vi "Beampointing_BELLA_PICObooster2.vi"() -> ()   [LabVIEW 2013]
uses:
  shared programs/GUI_Template/GUI_master/tcp_new_data_event.ctl
  shared programs/GUI_Template/GUI_master/tcp new data cluster.ctl
  Ctrs/beam detection.ctl
  GUI_Beampointing_single_TRA/Ctrs/move.ctl
  GUI_Stage_Cameras/Controls/Crosshair type def.ctl
  <vilib>/Utility/file.llb/Read From Spreadsheet File (string).vi
  <userlib>/_OpenG.lib/array/array.llb/Filter 1D Array with Scalar (String)__ogtk.vi
  <vilib>/Utility/file.llb/Write To Spreadsheet File (string).vi
  <vilib>/Analysis/NI_AALBase.lvlib
  <vilib>/vision/NI_Vision_Development_Module.lvlib
panel:
  in  "Position.Axis 121::98":dbl caption="Motor Axis 1" min=-10000.0 max=10000.0 format="%#_6f"
  in  "Position.Axis 122::98":dbl caption="Motor Axis 1" min=-10000.0 max=10000.0 format="%#_6f"
  in  "Position.Axis 111::98":dbl caption="Motor Axis 1" min=-10000.0 max=10000.0 format="%#_6f"
  in  "Position.Axis 112::98":dbl caption="Motor Axis 1" min=-10000.0 max=10000.0 format="%#_6f"
  in  "GUIdevice 98":string="LB-Picopad1"
  in  "Position.device 1::99":dbl=20.0 caption="Motor Axis 1" min=-10000.0 max=10000.0 format="%#_6f"
  in  "Position.device 2::99":dbl=-20.0 caption="Motor Axis 1" min=-10000.0 max=10000.0 format="%#_6f"
  in  "Position.device 4::99":dbl caption="Motor Axis 1" min=-10000.0 max=10000.0 format="%#_6f"
  in  "Position.device 5::99":dbl caption="Motor Axis 1" min=-10000.0 max=10000.0 format="%#_6f"
  out "error out 3":errorcluster
  out "error out":errorcluster
  out "Array 3":sgl[](array[numeric])=[35.01637, 16.987305, 27.281555, 56.5656, 0.0, 12.310791, 0.0, 0.0, 0.0, 0.0, 0.0, 0.0]
  in  "save path":path=path "W:/BP_DATA"
  out "size(s) 6":i32=12
  out "config path":string
  out "motor refs 7":refnum<vi>[](array[refnum])
  out "Moving Y":string
  out "Moving X":string
  out "particles":T1(array[cluster])=[{"Area"=13625.0, "Number of Holes"=0.0, "Bounding Rect"={"Left"=100.0, "Top"=93.0, "Right"=241.0, "Bottom"=225.0}, "Center of Mass"={"X"=171.3850275229358, "Y"=158.37277064220183}, "Orientation"=31.450434142859965, "Dimensions"={"Width"=141.0, "Height"=132.0}}]
  out "motor refs 6":refnum<vi>[](array[refnum])
  out "millisecond timer value":u32=150056294
  out "motor refs 5":refnum<vi>[](array[refnum])
  out "appended path":path=path "C:/Users/loasis.BELLANET/Documents/000 Labview/Developers Version/Interface/GUI_Beampointing_multi/defaultDevices_PICObooster.txt"
  out "motor refs 4":refnum<vi>[](array[refnum])
  in  "active Axis ref 3":cluster{"Ref X":refnum<vi>, "Ref Y":refnum<vi>}
  out "motor refs 3":refnum<vi>[](array[refnum])
  in  "active man refs":cluster{"Ref X":refnum<vi>, "Ref Y":refnum<vi>}
  out "motor refs 2":refnum<vi>[](array[refnum])
  in  "Numeric":dbl=2.0
  out "Current State":string="Exit"
  in  "output cluster 2":T5 {"detection para"."smal para"."Measurement Parameter" items=["Center of Mass X", "Center of Mass Y", "First Pixel X", "First Pixel Y", "Bounding Rect Left", "Bounding Rect Top", "Bounding Rect Right", "Bounding Rect Bottom", "Max Feret Diameter Start X", "Max Feret Diameter Start Y", "Max Feret Diameter End X", "Max Feret Diameter End Y", "Max Horiz. Segment Length Left", "Max Horiz. Segment Length Right", "Max Horiz. Segment Length Row", "-", "Bounding Rect Width", "Bounding Rect Height", "Bounding Rect Diagonal", "Perimeter", "Convex Hull Perimeter", "Holes' Perimeter", "Max Feret Diameter", "Equivalent Ellipse Major Axis", "Equivalent Ellipse Minor Axis", "Equivalent Ellipse Minor Axis (Feret)", "Equivalent Rect Long Side", "Equivalent Rect Short Side", "Equivalent Rect Diagonal", "Equivalent Rect Short Side (Feret)", "Average Horiz. Segment Length", "Average Vert. Segment Length", "Hydraulic Radius", "Waddel Disk Diameter", "-", "Area", "Holes' Area", "Particle & Holes' Area", "Convex Hull Area", "Image Area", "-", "Number of Holes", "Number of Horiz. Segments", "Number of Vert. Segments", "-", "Orientation", "Max Feret Diameter Orientation", "-", "% Area/Image Area", "% Area/(Particle & Holes' Area)", "Ratio of Equivalent Ellipse Axes", "Ratio of Equivalent Rect Sides", "-", "Elongation Factor", "Compactness Factor", "Heywood Circularity Factor", "Type Factor", "-", "Sum X", "Sum Y", "Sum XX", "Sum XY", "Sum YY", "Sum XXX", "Sum XXY", "Sum XYY", "Sum YYY", "-", "Moment of Inertia XX", "Moment of Inertia XY", "Moment of Inertia YY", "Moment of Inertia XXX", "Moment of Inertia XXY", "Moment of Inertia XYY", "Moment of Inertia YYY", "Norm. Moment of Inertia XX", "Norm. Moment of Inertia XY", "Norm. Moment of Inertia YY", "Norm. Moment of Inertia XXX", "Norm. Moment of Inertia XXY", "Norm. Moment of Inertia XYY", "Norm. Moment of Inertia YYY", "Hu Moment 1", "Hu Moment 2", "Hu Moment 3", "Hu Moment 4", "Hu Moment 5", "Hu Moment 6", "Hu Moment 7"]; "detection para"."smal para"."Range Lower Value" format="%.2f"; "detection para"."smal para"."Range Upper Value" format="%.2f"; "detection para"."detection method" items=["clustering", "entropy", "metric", "moments", "inter-class variance"]; "detection para"."Filter" items=["No Filter", "Median Filter", "Low Pass Filter"]}
  out "CCDs":string[](array[string])=["RegenCam", "BoosterCam", "PreampCam", "Amp1Cam", "Amp2Cam", "Amp3Cam", "", "", "", "", "", ""]
  in  "GUIdevice 12":string
  in  "GUIdevice 11":string
  in  "GUIdevice 10":string
  in  "GUIdevice 9":string
  out "error out 2":errorcluster
  in  "active cams":string[](array[string])
  in  "Motor Y":dbl[][](array[numeric])
  in  "Motor X":dbl[][](array[numeric])
  out "Names":string[](array[string])=["device12", "device45", "", ""]
  in  "Offset X stats":dbl[][](array[numeric])
  in  "Offset Y stats":dbl[][](array[numeric])
  out "Box":T6(array[cluster])=[{"Left"=100.0, "Top"=93.0, "Right"=241.0, "Bottom"=225.0}, {"Left"=87.0, "Top"=22.0, "Right"=220.0, "Bottom"=185.0}, {"Left"=80.0, "Top"=37.0, "Right"=220.0, "Bottom"=176.0}, {"Left"=78.0, "Top"=52.0, "Right"=221.0, "Bottom"=209.0}, {"Left"=0.0, "Top"=0.0, "Right"=0.0, "Bottom"=0.0}]
  in  "Tab Control 2":enum32{"Config ", "Main", "History"}(tab)=enum."Main"
  in  "associated motors":T7={"Motor CCD 1"=0, "Motor CCD 2"=0, "Motor CCD 3"=1, "Motor CCD 4"=0, "Motor CCD 5"=0, "Motor CCD 6"=0, "Motor CCD 7"=0, "Motor CCD 8"=0, "Motor CCD 9"=0, "Motor CCD 10"=0, "Motor CCD 11"=0, "Motor CCD 12"=0} {"Motor CCD 12" items=["Booster_pico", "Preamp_pico", "M21_pico", "Amp1out_pico"]; "Motor CCD 11" items=["Booster_pico", "Preamp_pico", "M21_pico", "Amp1out_pico"]; "Motor CCD 10" items=["Booster_pico", "Preamp_pico", "M21_pico", "Amp1out_pico"]; "Motor CCD 9" items=["Booster_pico", "Preamp_pico", "M21_pico", "Amp1out_pico"]; "Motor CCD 8" items=["Booster_pico", "Preamp_pico", "M21_pico", "Amp1out_pico"]; "Motor CCD 7" items=["Booster_pico", "Preamp_pico", "M21_pico", "Amp1out_pico"]; "Motor CCD 6" items=["Booster_pico", "Preamp_pico", "M21_pico", "Amp1out_pico"]; "Motor CCD 5" items=["Booster_pico", "Preamp_pico", "M21_pico", "Amp1out_pico"]; "Motor CCD 4" items=["Booster_pico", "Preamp_pico", "M21_pico", "Amp1out_pico"]; "Motor CCD 3" items=["Booster_pico", "Preamp_pico", "M21_pico", "Amp1out_pico"]; "Motor CCD 2" items=["Booster_pico", "Preamp_pico", "M21_pico", "Amp1out_pico"]; "Motor CCD 1" items=["Booster_pico", "Preamp_pico", "M21_pico", "Amp1out_pico"]}
  out "Cameras":T8={"[0]"="RegenCam", "[1]"="BoosterCam", "[2]"="PreampCam", "[3]"="Amp1Cam", "[4]"="Amp2Cam", "[5]"="Amp3Cam", "[6]"="", "[7]"="", "[8]"="", "[8] 2"="", "[8] 3"="", "[8] 4"=""}
  out "Status":cluster{i32, i32, "Centroid X":dbl[][]}(graph)={0, 1, "Centroid X"=[[171.87383691112902, 0.0, 0.0], [153.80799798158193, 0.0, 0.0], [147.97157969527117, 0.0, 0.0], [147.97285865350722, 0.0, 0.0], [0.0, 0.0, 0.0], [0.0, 0.0, 0.0], [0.0, 0.0, 0.0], [0.0, 0.0, 0.0], [0.0, 0.0, 0.0], [0.0, 0.0, 0.0], [0.0, 0.0, 0.0], [0.0, 0.0, 0.0]]}
  in  "Exposure:12":dbl=0.095 min=0.0001 max=1.0 format="%#_6f"
  in  "Triggerdelay::12":dbl=0.003 min=0.0 max=0.09 format="%#_6f"
  in  "Exposure::11":dbl=0.095 min=0.0001 max=1.0 format="%#_6f"
  in  "Triggerdelay::11":dbl=0.003 min=0.0 max=0.09 format="%#_6f"
  in  "Exposure::10":dbl=0.095 min=0.0001 max=1.0 format="%#_6f"
  in  "Triggerdelay::10":dbl=0.003 min=0.0 max=0.09 format="%#_6f"
  in  "Exposure::9":dbl=0.095 min=0.0001 max=1.0 format="%#_6f"
  in  "Triggerdelay::9":dbl=0.003 min=0.0 max=0.09 format="%#_6f"
  in  "Trigger::9":bool
  in  "Trigger::10":bool caption="Trigger:10"
  in  "Trigger::11":bool
  in  "Trigger::12":bool
  in  "Target.Y::9":dbl=45.0 caption="T9y" min=0.0 max=2000.0 format="%#_6f"
  in  "Target.X::9":dbl=47.0 caption="Tx9" min=0.0 max=2000.0 format="%#_6f"
  in  "Target.Y::10":dbl=45.0 caption="T10y" min=0.0 max=2000.0 format="%#_6f"
  in  "Target.X::10":dbl=47.0 caption="T10x" min=0.0 max=2000.0 format="%#_6f"
  in  "Target.Y::11":dbl=45.0 caption="T11y" min=0.0 max=2000.0 format="%#_6f"
  in  "Target.X::11":dbl=47.0 caption="T11x" min=0.0 max=2000.0 format="%#_6f"
  in  "Target.Y::12":dbl=45.0 caption="T12y" min=0.0 max=2000.0 format="%#_6f"
  in  "Target.X::12":dbl=47.0 caption="T12x" min=0.0 max=2000.0 format="%#_6f"
  in  "Exposure::8":dbl=0.095 min=0.0001 max=1.0 format="%#_6f"
  in  "Triggerdelay::8":dbl=0.003 min=0.0 max=0.09 format="%#_6f"
  in  "Trigger::8":bool
  in  "Target.Y::8":dbl=45.0 caption="T8y" min=0.0 max=2000.0 format="%#_6f"
  in  "Target.X::8":dbl=47.0 caption="T8x" min=0.0 max=2000.0 format="%#_6f"
  in  "Target.Y::7":dbl=45.0 caption="T7x" min=0.0 max=2000.0 format="%#_6f"
  in  "Target.X::7":dbl=47.0 caption="T7y" min=0.0 max=2000.0 format="%#_6f"
  in  "Target.Y::6":dbl=142.0 caption="T6y" min=0.0 max=5000.0 format="%#_6f"
  in  "Target.X::6":dbl=123.0 caption="T6x" min=0.0 max=5000.0 format="%#_6f"
  in  "Target.Y::5":dbl=108.0 caption="T5y" min=0.0 max=2000.0 format="%#_6f"
  in  "Target.X::5":dbl=172.0 caption="T5x" min=0.0 max=2000.0 format="%#_6f"
  in  "Target.Y::4":dbl=130.0 caption="T4y" min=0.0 max=5000.0 format="%#_6f"
  in  "Target.X::4":dbl=148.0 caption="T4x" min=0.0 max=5000.0 format="%#_6f"
  in  "Target.Y::3":dbl=110.0 caption="T3y" min=0.0 max=5000.0 format="%#_6f"
  in  "Target.X::3":dbl=154.0 caption="T3x" min=0.0 max=5000.0 format="%#_6f"
  in  "Target.Y::2":dbl=106.0 caption="T2y" min=0.0 max=5000.0 format="%#_6f"
  in  "Target.X::2":dbl=163.0 caption="T2x" min=0.0 max=5000.0 format="%#_6f"
  in  "Target.Y::1":dbl=162.0 caption="T1y" min=0.0 max=5000.0 format="%#_6f"
  in  "Target.X::1":dbl=171.0 caption="T1x" min=0.0 max=5000.0 format="%#_6f"
  in  "Exposure::7":dbl=0.095 min=3.8e-05 max=1.0 format="%#_6f"
  in  "Triggerdelay::7":dbl=0.003 min=0.0 max=0.09 format="%#_6f"
  in  "Trigger::7":bool
  in  "Exposure::6":dbl=0.095 min=3.8e-05 max=1.0 format="%#_6f"
  in  "Triggerdelay::6":dbl=0.003 min=0.0 max=0.09 format="%#_6f"
  in  "Trigger::6":bool
  in  "Exposure::5":dbl=0.095 min=3.8e-05 max=1.0 format="%#_6f"
  in  "Triggerdelay::5":dbl=0.003 min=0.0 max=0.09 format="%#_6f"
  in  "Trigger::5":bool
  in  "Exposure::4":dbl=0.095 min=3.8e-05 max=1.0 format="%#_6f"
  in  "Triggerdelay::4":dbl=0.003 min=0.0 max=0.09 format="%#_6f"
  in  "Trigger::4":bool
  in  "Exposure::3":dbl=0.095 min=3.8e-05 max=1.0 format="%#_6f"
  in  "Triggerdelay::3":dbl=0.003 min=0.0 max=0.09 format="%#_6f"
  in  "Trigger::3":bool
  in  "Exposure::2":dbl=0.095 min=3.8e-05 max=2.0 format="%#_6f"
  in  "Triggerdelay::2":dbl=0.003 min=0.0 max=0.09 format="%#_6f"
  in  "Trigger::2":bool
  out "image::1":T9(plugin-control) caption="RegenCam"
  out "image::2":T9(plugin-control) caption="BoosterCam"
  out "image::3":T9(plugin-control) caption="PreampCam"
  out "image::4":T9(plugin-control) caption="Amp1Cam"
  out "image::5":T9(plugin-control) caption="Tel4_Cam"
  out "image::6":T9(plugin-control)
  out "image::7":T9(plugin-control)
  out "image::8":T9(plugin-control)
  in  "Exposure::1":dbl=0.095 min=3.8e-05 max=1.0 format="%#_6f"
  in  "Triggerdelay::1":dbl=0.003 min=0.0 max=0.09 format="%#_6f"
  in  "Trigger::1":bool
  in  "UDP error message":string
  out "required Y":bool[](array[boolean])=[FALSE, TRUE, FALSE, FALSE, FALSE]
  out "required X":bool[](array[boolean])=[FALSE, TRUE, FALSE, FALSE, FALSE]
  out "detected":bool[](array[boolean])=[TRUE, TRUE, TRUE, TRUE, FALSE]
  out "name array":string[](array[string])=["RegenCam", "BoosterCam", "PreampCam", "Amp1Cam", "Amp3Cam"]
  out "image::9":T9(plugin-control)
  out "image::10":T9(plugin-control)
  out "image::11":T9(plugin-control)
  out "image::12":T9(plugin-control)
  out "speedmode X":bool[](array[boolean])=[TRUE, TRUE, TRUE, TRUE, FALSE]
  out "speedmode Y":bool[](array[boolean])=[TRUE, FALSE, TRUE, TRUE, FALSE]
  out "CCD 9":cluster{timestamp[], dbl[]}[](graph)=[{[timestamp(3549547983.3591223 s since 1904-01-01)], [0.0]}, {[timestamp(3549547983.3591223 s since 1904-01-01)], [0.0]}, {[timestamp(3549547983.3591223 s since 1904-01-01)], [20.0]}, {[timestamp(3549547983.3591223 s since 1904-01-01)], [-20.0, -20.0, -20.0, -20.0]}]
  out "CCD 10":cluster{timestamp[], dbl[]}[](graph)=[{[timestamp(3549547983.360123 s since 1904-01-01)], [0.0]}, {[timestamp(3549547983.360123 s since 1904-01-01)], [0.0]}, {[timestamp(3549547983.360123 s since 1904-01-01)], [20.0]}, {[timestamp(3549547983.360123 s since 1904-01-01)], [-20.0, -20.0, -20.0, -20.0]}]
  out "CCD 11":cluster{timestamp[], dbl[]}[](graph)=[{[timestamp(3549547983.360123 s since 1904-01-01)], [0.0]}, {[timestamp(3549547983.360123 s since 1904-01-01)], [0.0]}, {[timestamp(3549547983.360123 s since 1904-01-01)], [20.0]}, {[timestamp(3549547983.360123 s since 1904-01-01)], [-20.0, -20.0, -20.0, -20.0]}]
  out "CCD 12":cluster{timestamp[], dbl[]}[](graph)=[{[timestamp(3549547983.360123 s since 1904-01-01)], [0.0]}, {[timestamp(3549547983.360123 s since 1904-01-01)], [0.0]}, {[timestamp(3549547983.360123 s since 1904-01-01)], [20.0]}, {[timestamp(3549547983.360123 s since 1904-01-01)], [-20.0, -20.0, -20.0, -20.0]}]
  out "CCD 5":cluster{timestamp[], dbl[]}[](graph)=[{[timestamp(3549547983.358122 s since 1904-01-01)], [0.0]}, {[timestamp(3549547983.358122 s since 1904-01-01)], [0.0]}, {[timestamp(3549547983.358122 s since 1904-01-01)], [20.0]}, {[timestamp(3549547983.358122 s since 1904-01-01)], [-20.0, -20.0, -20.0, -20.0]}] caption="Tel4_Cam"
  out "CCD 6":cluster{timestamp[], dbl[]}[](graph)=[{[timestamp(3549547983.3591223 s since 1904-01-01)], [0.0]}, {[timestamp(3549547983.3591223 s since 1904-01-01)], [0.0]}, {[timestamp(3549547983.3591223 s since 1904-01-01)], [20.0]}, {[timestamp(3549547983.3591223 s since 1904-01-01)], [-20.0, -20.0, -20.0, -20.0]}]
  out "CCD 7":cluster{timestamp[], dbl[]}[](graph)=[{[timestamp(3549547983.3591223 s since 1904-01-01)], [0.0]}, {[timestamp(3549547983.3591223 s since 1904-01-01)], [0.0]}, {[timestamp(3549547983.3591223 s since 1904-01-01)], [20.0]}, {[timestamp(3549547983.3591223 s since 1904-01-01)], [-20.0, -20.0, -20.0, -20.0]}]
  out "CCD 8":cluster{timestamp[], dbl[]}[](graph)=[{[timestamp(3549547983.3591223 s since 1904-01-01)], [0.0]}, {[timestamp(3549547983.3591223 s since 1904-01-01)], [0.0]}, {[timestamp(3549547983.3591223 s since 1904-01-01)], [20.0]}, {[timestamp(3549547983.3591223 s since 1904-01-01)], [-20.0, -20.0, -20.0, -20.0]}]
  out "CCD 2":cluster{timestamp[], dbl[]}[](graph)=[{[timestamp(3549547983.358122 s since 1904-01-01)], [3.0783937413765585]}, {[timestamp(3549547983.358122 s since 1904-01-01)], [8.883046862591215]}, {[timestamp(3549547983.358122 s since 1904-01-01)], [20.0]}, {[timestamp(3549547983.358122 s since 1904-01-01)], [-20.0, -20.0, -20.0, -20.0]}] caption="BoosterCam"
  out "CCD 1":cluster{timestamp[], dbl[]}[](graph)=[{[timestamp(3549547983.357121 s since 1904-01-01)], [3.1654865062995725]}, {[timestamp(3549547983.357121 s since 1904-01-01)], [-0.42630614615123363]}, {[timestamp(3549547983.357121 s since 1904-01-01)], [20.0]}, {[timestamp(3549547983.357121 s since 1904-01-01)], [-20.0, -20.0, -20.0, -20.0]}] caption="RegenCam"
  out "CCD 3":cluster{timestamp[], dbl[]}[](graph)=[{[timestamp(3549547983.358122 s since 1904-01-01)], [5.607599326451648]}, {[timestamp(3549547983.358122 s since 1904-01-01)], [4.73033759911138]}, {[timestamp(3549547983.358122 s since 1904-01-01)], [0.0]}, {[timestamp(3549547983.358122 s since 1904-01-01)], [0.0, 0.0, 0.0, 0.0]}] caption="PreampCam"
  out "CCD 4":cluster{timestamp[], dbl[]}[](graph)=[{[timestamp(3549547983.358122 s since 1904-01-01)], [1.2734976836249814]}, {[timestamp(3549547983.358122 s since 1904-01-01)], [-0.6350086940318818]}, {[timestamp(3549547983.358122 s since 1904-01-01)], [20.0]}, {[timestamp(3549547983.358122 s since 1904-01-01)], [-20.0, -20.0, -20.0, -20.0]}] caption="Amp1Cam"
  in  "History Size":i32=2000
  out "History Index":i32=1
  in  "Feedback Global":bool
  in  "detection para":T3[](array[typedef])=[{"Filter"=1, "Filter Para"={"X Size"=5, "Y Size"=5, "% Tolerance"=1}, "detection method"=4, "smal para"=[{"Measurement Parameter"=35, "Range Lower Value"=0.0, "Range Upper Value"=0.0, "Range"=TRUE, "Measurement Type"=FALSE}], "Remove small Objects"=TRUE, "Restrict to round Objects"=FALSE}, {"Filter"=1, "Filter Para"={"X Size"=5, "Y Size"=5, "% Tolerance"=1}, "detection method"=4, "smal para"=[{"Measurement Parameter"=35, "Range Lower Value"=0.0, "Range Upper Value"=500.0, "Range"=FALSE, "Measurement Type"=FALSE}], "Remove small Objects"=TRUE, "Restrict to round Objects"=FALSE}, {"Filter"=1, "Filter Para"={"X Size"=5, "Y Size"=5, "% Tolerance"=1}, "detection method"=4, "smal para"=[{"Measurement Parameter"=35, "Range Lower Value"=0.0, "Range Upper Value"=500.0, "Range"=TRUE, "Measurement Type"=FALSE}], "Remove small Objects"=TRUE, "Restrict to round Objects"=FALSE}, {"Filter"=1, "Filter Para"={"X Size"=5, "Y Size"=5, "% Tolerance"=1}, "detection method"=4, "smal para"=[{"Measurement Parameter"=35, "Range Lower Value"=0.0, "Range Upper Value"=500.0, "Range"=TRUE, "Measurement Type"=FALSE}], "Remove small Objects"=TRUE, "Restrict to round Objects"=FALSE}, {"Filter"=1, "Filter Para"={"X Size"=5, "Y Size"=5, "% Tolerance"=1}, "detection method"=4, "smal para"=[{"Measurement Parameter"=35, "Range Lower Value"=0.0, "Range Upper Value"=500.0, "Range"=TRUE, "Measurement Type"=FALSE}], "Remove small Objects"=TRUE, "Restrict to round Objects"=FALSE}, {"Filter"=1, "Filter Para"={"X Size"=5, "Y Size"=5, "% Tolerance"=1}, "detection method"=4, "smal para"=[{"Measurement Parameter"=35, "Range Lower Value"=0.0, "Range Upper Value"=500.0, "Range"=TRUE, "Measurement Type"=FALSE}], "Remove small Objects"=TRUE, "Restrict to round Objects"=FALSE}, {"Filter"=1, "Filter Para"={"X Size"=5, "Y Size"=5, "% Tolerance"=1}, "detection method"=4, "smal para"=[{"Measurement Parameter"=35, "Range Lower Value"=0.0, "Range Upper Value"=500.0, "Range"=TRUE, "Measurement Type"=FALSE}], "Remove small Objects"=TRUE, "Restrict to round Objects"=FALSE}, {"Filter"=1, "Filter Para"={"X Size"=5, "Y Size"=5, "% Tolerance"=1}, "detection method"=3, "smal para"=[{"Measurement Parameter"=35, "Range Lower Value"=0.0, "Range Upper Value"=0.0, "Range"=FALSE, "Measurement Type"=FALSE}], "Remove small Objects"=TRUE, "Restrict to round Objects"=FALSE}, {"Filter"=1, "Filter Para"={"X Size"=5, "Y Size"=5, "% Tolerance"=1}, "detection method"=4, "smal para"=[{"Measurement Parameter"=35, "Range Lower Value"=0.0, "Range Upper Value"=0.0, "Range"=FALSE, "Measurement Type"=FALSE}], "Remove small Objects"=TRUE, "Restrict to round Objects"=FALSE}, {"Filter"=1, "Filter Para"={"X Size"=5, "Y Size"=5, "% Tolerance"=1}, "detection method"=4, "smal para"=[{"Measurement Parameter"=35, "Range Lower Value"=0.0, "Range Upper Value"=500.0, "Range"=TRUE, "Measurement Type"=FALSE}], "Remove small Objects"=TRUE, "Restrict to round Objects"=FALSE}, {"Filter"=1, "Filter Para"={"X Size"=5, "Y Size"=5, "% Tolerance"=1}, "detection method"=4, "smal para"=[{"Measurement Parameter"=35, "Range Lower Value"=0.0, "Range Upper Value"=500.0, "Range"=TRUE, "Measurement Type"=FALSE}], "Remove small Objects"=TRUE, "Restrict to round Objects"=FALSE}, {"Filter"=1, "Filter Para"={"X Size"=5, "Y Size"=5, "% Tolerance"=1}, "detection method"=4, "smal para"=[{"Measurement Parameter"=35, "Range Lower Value"=0.0, "Range Upper Value"=500.0, "Range"=TRUE, "Measurement Type"=FALSE}], "Remove small Objects"=TRUE, "Restrict to round Objects"=FALSE}] {"smal para"."Measurement Parameter" items=["Center of Mass X", "Center of Mass Y", "First Pixel X", "First Pixel Y", "Bounding Rect Left", "Bounding Rect Top", "Bounding Rect Right", "Bounding Rect Bottom", "Max Feret Diameter Start X", "Max Feret Diameter Start Y", "Max Feret Diameter End X", "Max Feret Diameter End Y", "Max Horiz. Segment Length Left", "Max Horiz. Segment Length Right", "Max Horiz. Segment Length Row", "-", "Bounding Rect Width", "Bounding Rect Height", "Bounding Rect Diagonal", "Perimeter", "Convex Hull Perimeter", "Holes' Perimeter", "Max Feret Diameter", "Equivalent Ellipse Major Axis", "Equivalent Ellipse Minor Axis", "Equivalent Ellipse Minor Axis (Feret)", "Equivalent Rect Long Side", "Equivalent Rect Short Side", "Equivalent Rect Diagonal", "Equivalent Rect Short Side (Feret)", "Average Horiz. Segment Length", "Average Vert. Segment Length", "Hydraulic Radius", "Waddel Disk Diameter", "-", "Area", "Holes' Area", "Particle & Holes' Area", "Convex Hull Area", "Image Area", "-", "Number of Holes", "Number of Horiz. Segments", "Number of Vert. Segments", "-", "Orientation", "Max Feret Diameter Orientation", "-", "% Area/Image Area", "% Area/(Particle & Holes' Area)", "Ratio of Equivalent Ellipse Axes", "Ratio of Equivalent Rect Sides", "-", "Elongation Factor", "Compactness Factor", "Heywood Circularity Factor", "Type Factor", "-", "Sum X", "Sum Y", "Sum XX", "Sum XY", "Sum YY", "Sum XXX", "Sum XXY", "Sum XYY", "Sum YYY", "-", "Moment of Inertia XX", "Moment of Inertia XY", "Moment of Inertia YY", "Moment of Inertia XXX", "Moment of Inertia XXY", "Moment of Inertia XYY", "Moment of Inertia YYY", "Norm. Moment of Inertia XX", "Norm. Moment of Inertia XY", "Norm. Moment of Inertia YY", "Norm. Moment of Inertia XXX", "Norm. Moment of Inertia XXY", "Norm. Moment of Inertia XYY", "Norm. Moment of Inertia YYY", "Hu Moment 1", "Hu Moment 2", "Hu Moment 3", "Hu Moment 4", "Hu Moment 5", "Hu Moment 6", "Hu Moment 7"]; "smal para"."Range Lower Value" format="%.2f"; "smal para"."Range Upper Value" format="%.2f"; "detection method" items=["clustering", "entropy", "metric", "moments", "inter-class variance"]; "Filter" items=["No Filter", "Median Filter", "Low Pass Filter"]}
  in  "GUIdevice 8":string
  in  "Tab Control":T10(tab)
  in  "new tdms":bool
  in  "Save Stats":bool
  in  "Save Config":bool
  in  "Load Config":bool
  in  "update speed [ms]":i32=2000
  in  "img to avg":i32=6 min=3 max=200
  in  "Reset History":bool
  in  "autodetect":bool
  in  "Detection Rate":dbl=0.8 min=0.001 max=1.0
  in  "Center":bool
  in  "Align":bool
  in  "Speedmode @":dbl=5.0 min=1.0 max=20.0
  in  "device ini":bool
  in  "beam detection para":T3={"Filter"=1, "Filter Para"={"X Size"=5, "Y Size"=5, "% Tolerance"=1}, "detection method"=4, "smal para"=[{"Measurement Parameter"=35, "Range Lower Value"=0.0, "Range Upper Value"=500.0, "Range"=FALSE, "Measurement Type"=FALSE}], "Remove small Objects"=TRUE, "Restrict to round Objects"=FALSE} {"smal para"."Measurement Parameter" items=["Center of Mass X", "Center of Mass Y", "First Pixel X", "First Pixel Y", "Bounding Rect Left", "Bounding Rect Top", "Bounding Rect Right", "Bounding Rect Bottom", "Max Feret Diameter Start X", "Max Feret Diameter Start Y", "Max Feret Diameter End X", "Max Feret Diameter End Y", "Max Horiz. Segment Length Left", "Max Horiz. Segment Length Right", "Max Horiz. Segment Length Row", "-", "Bounding Rect Width", "Bounding Rect Height", "Bounding Rect Diagonal", "Perimeter", "Convex Hull Perimeter", "Holes' Perimeter", "Max Feret Diameter", "Equivalent Ellipse Major Axis", "Equivalent Ellipse Minor Axis", "Equivalent Ellipse Minor Axis (Feret)", "Equivalent Rect Long Side", "Equivalent Rect Short Side", "Equivalent Rect Diagonal", "Equivalent Rect Short Side (Feret)", "Average Horiz. Segment Length", "Average Vert. Segment Length", "Hydraulic Radius", "Waddel Disk Diameter", "-", "Area", "Holes' Area", "Particle & Holes' Area", "Convex Hull Area", "Image Area", "-", "Number of Holes", "Number of Horiz. Segments", "Number of Vert. Segments", "-", "Orientation", "Max Feret Diameter Orientation", "-", "% Area/Image Area", "% Area/(Particle & Holes' Area)", "Ratio of Equivalent Ellipse Axes", "Ratio of Equivalent Rect Sides", "-", "Elongation Factor", "Compactness Factor", "Heywood Circularity Factor", "Type Factor", "-", "Sum X", "Sum Y", "Sum XX", "Sum XY", "Sum YY", "Sum XXX", "Sum XXY", "Sum XYY", "Sum YYY", "-", "Moment of Inertia XX", "Moment of Inertia XY", "Moment of Inertia YY", "Moment of Inertia XXX", "Moment of Inertia XXY", "Moment of Inertia XYY", "Moment of Inertia YYY", "Norm. Moment of Inertia XX", "Norm. Moment of Inertia XY", "Norm. Moment of Inertia YY", "Norm. Moment of Inertia XXX", "Norm. Moment of Inertia XXY", "Norm. Moment of Inertia XYY", "Norm. Moment of Inertia YYY", "Hu Moment 1", "Hu Moment 2", "Hu Moment 3", "Hu Moment 4", "Hu Moment 5", "Hu Moment 6", "Hu Moment 7"]; "smal para"."Range Lower Value" format="%.2f"; "smal para"."Range Upper Value" format="%.2f"; "detection method" items=["clustering", "entropy", "metric", "moments", "inter-class variance"]; "Filter" items=["No Filter", "Median Filter", "Low Pass Filter"]}
  in  "move config":T2={"Tolerance [%]"=0.1, "Stepsize"=0.0001, "Invert Axis"=TRUE, "Invert Direction X"=FALSE, "Invert Direction Y"=TRUE, "enable feedback"=FALSE, "Set Centriod Target"=FALSE}
  in  "Position 2":dbl=-20.0 caption="Stepsize" min=0.0 max=999999.0 format="%_6f"
  in  "Position 1":dbl=20.0 caption="Stepsize" min=0.0 max=999999.0 format="%_6f"
  in  "Right":bool caption="RelativeMove.Axis 1.CCW::1"
  in  "Left":bool caption="RelativeMove.Axis 1.CW::1"
  in  "Down":bool caption="RelativeMove.Axis. 2.CCW::1"
  in  "Up":bool caption="RelativeMove.Axis 2.CW::1"
  in  "StepSize":dbl=5.0 caption="Stepsize" min=0.0 max=500.0 format="%#.4f"
  in  "active axis refs 2":T11(array[cluster])
  in  "active Axis ref":cluster{"Ref X":refnum<vi>, "Ref Y":refnum<vi>}
  in  "CCDs":u16(ring) items=["RegenCam", "BoosterCam", "PreampCam", "Amp1Cam", "Tel4_Cam", "", "", "", "", "", "", ""]
  out "motor refs":refnum<vi>[](array[refnum])
  in  "GUIdevice 99":string="LB-Pico-Booster"
  in  "move properties":T2[](array[typedef])=[{"Tolerance [%]"=0.1, "Stepsize"=0.0001, "Invert Axis"=TRUE, "Invert Direction X"=FALSE, "Invert Direction Y"=TRUE, "enable feedback"=FALSE, "Set Centriod Target"=FALSE}, {"Tolerance [%]"=0.1, "Stepsize"=0.0001, "Invert Axis"=TRUE, "Invert Direction X"=FALSE, "Invert Direction Y"=TRUE, "enable feedback"=FALSE, "Set Centriod Target"=FALSE}, {"Tolerance [%]"=0.1, "Stepsize"=0.0001, "Invert Axis"=TRUE, "Invert Direction X"=FALSE, "Invert Direction Y"=TRUE, "enable feedback"=FALSE, "Set Centriod Target"=FALSE}, {"Tolerance [%]"=0.1, "Stepsize"=0.0001, "Invert Axis"=TRUE, "Invert Direction X"=FALSE, "Invert Direction Y"=TRUE, "enable feedback"=FALSE, "Set Centriod Target"=FALSE}, {"Tolerance [%]"=0.1, "Stepsize"=0.0001, "Invert Axis"=TRUE, "Invert Direction X"=FALSE, "Invert Direction Y"=TRUE, "enable feedback"=FALSE, "Set Centriod Target"=FALSE}, {"Tolerance [%]"=0.1, "Stepsize"=0.0001, "Invert Axis"=TRUE, "Invert Direction X"=FALSE, "Invert Direction Y"=TRUE, "enable feedback"=FALSE, "Set Centriod Target"=FALSE}, {"Tolerance [%]"=0.1, "Stepsize"=0.0001, "Invert Axis"=TRUE, "Invert Direction X"=FALSE, "Invert Direction Y"=TRUE, "enable feedback"=FALSE, "Set Centriod Target"=FALSE}, {"Tolerance [%]"=0.1, "Stepsize"=0.0001, "Invert Axis"=TRUE, "Invert Direction X"=FALSE, "Invert Direction Y"=TRUE, "enable feedback"=FALSE, "Set Centriod Target"=FALSE}, {"Tolerance [%]"=0.1, "Stepsize"=0.0001, "Invert Axis"=TRUE, "Invert Direction X"=FALSE, "Invert Direction Y"=TRUE, "enable feedback"=FALSE, "Set Centriod Target"=FALSE}, {"Tolerance [%]"=0.1, "Stepsize"=0.0001, "Invert Axis"=TRUE, "Invert Direction X"=FALSE, "Invert Direction Y"=TRUE, "enable feedback"=FALSE, "Set Centriod Target"=FALSE}, {"Tolerance [%]"=0.1, "Stepsize"=0.0001, "Invert Axis"=TRUE, "Invert Direction X"=FALSE, "Invert Direction Y"=TRUE, "enable feedback"=FALSE, "Set Centriod Target"=FALSE}, {"Tolerance [%]"=0.1, "Stepsize"=0.0001, "Invert Axis"=TRUE, "Invert Direction X"=FALSE, "Invert Direction Y"=TRUE, "enable feedback"=FALSE, "Set Centriod Target"=FALSE}, {"Tolerance [%]"=0.1, "Stepsize"=0.0001, "Invert Axis"=TRUE, "Invert Direction X"=FALSE, "Invert Direction Y"=TRUE, "enable feedback"=FALSE, "Set Centriod Target"=FALSE}]
  in  "Time":timestamp[][](array[timestamp])
  in  "Mean Size":dbl[][](array[numeric])
  in  "Size":dbl[][](array[numeric])
  in  "active CCDs":i32(listbox)=-1
  in  "Offset Y":dbl[][](array[numeric])
  in  "Offset X":dbl[][](array[numeric])
  in  "Mean Centroid X":dbl[][](array[numeric])
  in  "Mean Centroid Y":dbl[][](array[numeric])
  in  "Centroid Y":dbl[][](array[numeric])
  in  "Centroid X":dbl[][](array[numeric])
  in  "GUIdevice 7":string
  in  "GUIdevice 6":string="Amp3Cam"
  in  "GUIdevice 5":string="Amp2Cam"
  in  "GUIdevice 4":string="Amp1Cam"
  in  "GUIdevice 3":string="PreampCam"
  in  "GUIdevice 2":string="BoosterCam"
  in  "insert tag":bool=TRUE
  in  "stop":bool
  in  "GUIdevice 1":string="RegenCam"
  out "tcp data event":T12
  out "error IO 2":errorcluster
  # "x [Tolerance]"
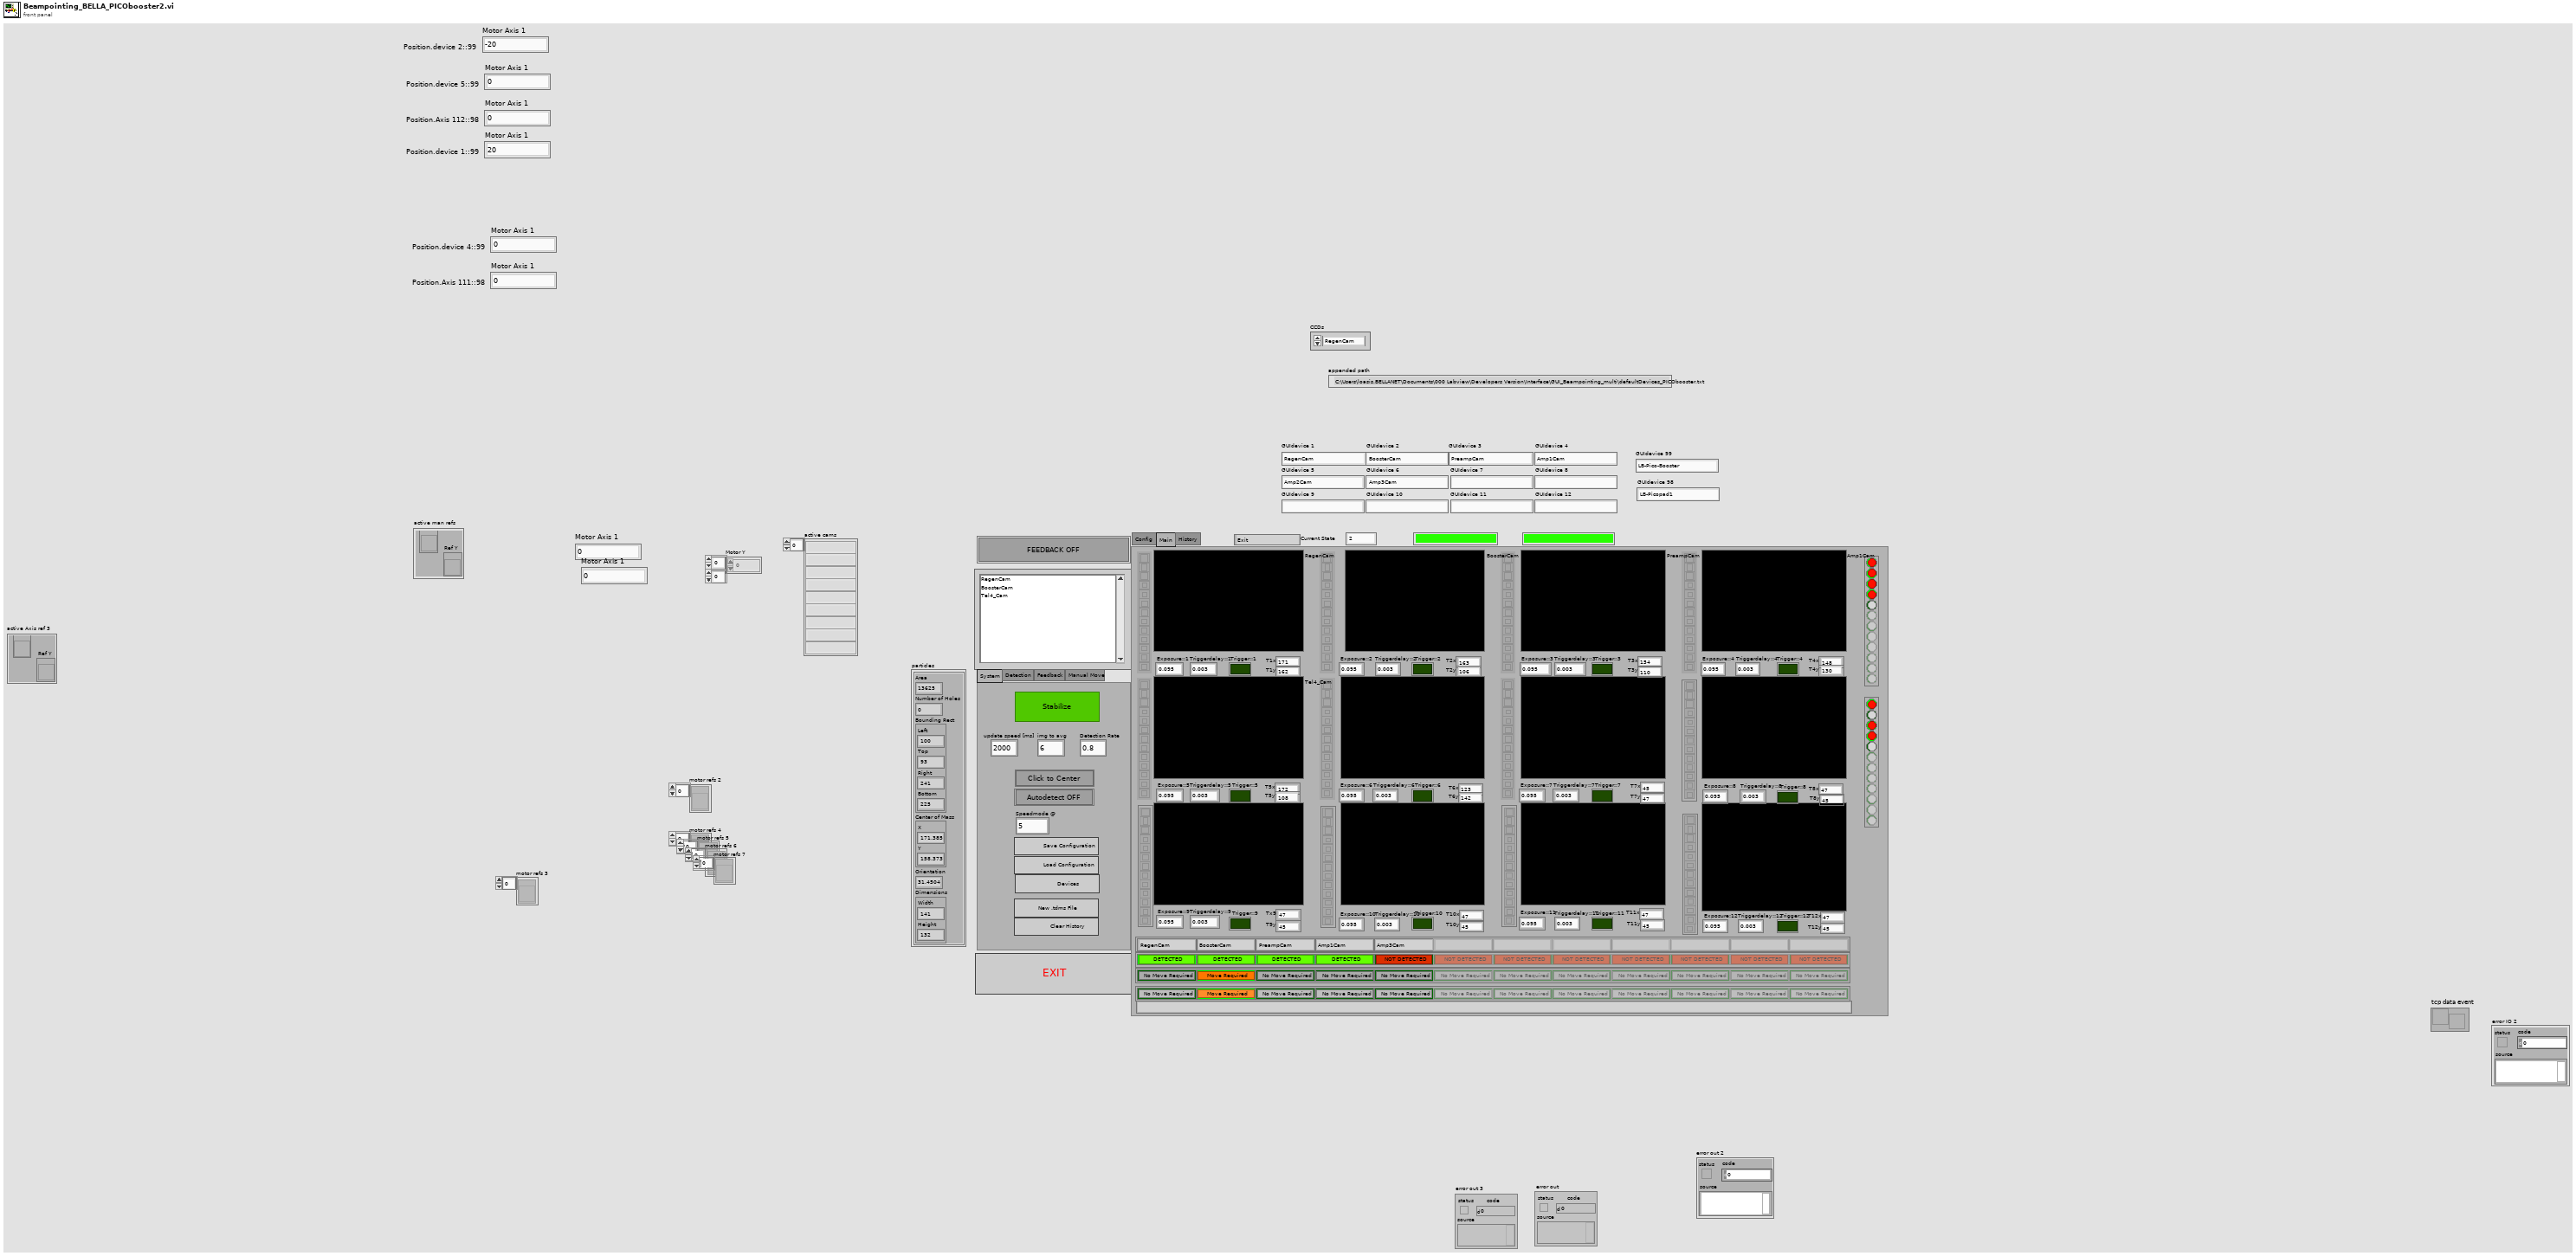
[diagram p1: front panel]
types:
  T1 = cluster{"Area":dbl, "Number of Holes":dbl, "Bounding Rect":cluster{"Left":dbl, "Top":dbl, "Right":dbl, "Bottom":dbl}, "Center of Mass":cluster{"X":dbl, "Y":dbl}, "Orientation":dbl, "Dimensions":cluster{"Width":dbl, "Height":dbl}}[]
  T2 = typedef "move.ctl" = cluster{"Tolerance [%]":dbl, "Stepsize":dbl, "Invert Axis":bool, "Invert Direction X":bool, "Invert Direction Y":bool, "enable feedback":bool, "Set Centriod Target":bool}
  T3 = typedef "beam detection.ctl" = cluster{"Filter":u16, "Filter Para":cluster{"X Size":i32, "Y Size":i32, "% Tolerance":i32}, "detection method":i32, "smal para":cluster{"Measurement Parameter":T4, "Range Lower Value":dbl, "Range Upper Value":dbl, "Range":bool, "Measurement Type":bool}[], "Remove small Objects":bool, "Restrict to round Objects":bool}
  T4 = typedef "Particle Parameters" = i32
  T5 = cluster{"CCDs":string[], "move properties":T2[], "detection para":T3[], "thresholds":cluster{"Lower value":sgl, "Upper value":sgl}[], "Value":cluster{"Motor CCD 1":u16, "Motor CCD 2":u16, "Motor CCD 3":u16, "Motor CCD 4":u16, "Motor CCD 5":u16, "Motor CCD 6":u16, "Motor CCD 7":u16, "Motor CCD 8":u16, "Motor CCD 9":u16, "Motor CCD 10":u16, "Motor CCD 11":u16, "Motor CCD 12":u16}}
  T6 = cluster{"Left":dbl, "Top":dbl, "Right":dbl, "Bottom":dbl}[]
  T7 = cluster{"Motor CCD 1":u16, "Motor CCD 2":u16, "Motor CCD 3":u16, "Motor CCD 4":u16, "Motor CCD 5":u16, "Motor CCD 6":u16, "Motor CCD 7":u16, "Motor CCD 8":u16, "Motor CCD 9":u16, "Motor CCD 10":u16, "Motor CCD 11":u16, "Motor CCD 12":u16}
  T8 = cluster{"[0]":string, "[1]":string, "[2]":string, "[3]":string, "[4]":string, "[5]":string, "[6]":string, "[7]":string, "[8]":string, "[8] 2":string, "[8] 3":string, "[8] 4":string}
  T9 = typedef "IMAQ Image.ctl" = refnum<image>
  T10 = enum32{"System", "Detection", "Feedback", "Manual Move"}
  T11 = cluster{"Ref X":refnum<vi>, "Ref Y":refnum<vi>}[]
  T12 = typedef "tcp_new_data_event.ctl" = refnum<user-event>
  T13 = typedef "tcp new data cluster.ctl" = cluster{"EventEnum":enum16{"new data", "connection status update"}, "Device name":string}
  T14 = typedef "Crosshair type def.ctl" = cluster{"Draw":bool, "Target":cluster{"x":dbl, "y":dbl}, "Size":cluster{"x":dbl, "y":dbl}, "Angle":dbl, "Color":u32}
  T15 = cluster{"Left":i32, "Top":i32, "Right":i32, "Bottom":i32}
  T16 = enum32{"invalid app kind", "Development System", "Run Time System", "Student Edition", "Embedded LabVIEW", "Evaluation", "Custom"}
  T17 = enum16{"open", "open or create", "create or replace", "create", "open (read-only)"}
  T18 = enum32{"Invalid", "Standard", "Closed", "Hidden", "Minimized", "Maximized"}
  T19 = enum16{"open", "replace", "create", "open or create", "replace or create", "replace or create with confirmation"}
  T20 = enum8{"Enabled", "Disabled", "Disabled and Grayed Out"}
  T21 = typedef "Image Type" = u32
  T22 = cluster{"[0]":string, "[1]":string, "[2]":string, "[3]":string, "[4]":string, "[5]":string, "[6]":string, "[7]":string, "[8]":string, "[9]":string, "[10]":string, "[11]":string}
  T23 = cluster{"Target.X::1":refnum<vi>, "Target.Y::1":refnum<vi>}
  T24 = cluster{"Target.X::2":refnum<vi>, "Target.Y::2":refnum<vi>}
  T25 = cluster{"Target.X::3":refnum<vi>, "Target.Y::3":refnum<vi>}
  T26 = cluster{"Target.X::4":refnum<vi>, "Target.Y::4":refnum<vi>}
  T27 = cluster{"Target.X::5":refnum<vi>, "Target.Y::5":refnum<vi>}
  T28 = cluster{"Target.X::6":refnum<vi>, "Target.Y::6":refnum<vi>}
  T29 = cluster{"Target.X::7":refnum<vi>, "Target.Y::7":refnum<vi>}
  T30 = cluster{"Target.X::8":refnum<vi>, "Target.Y::8":refnum<vi>}
  T31 = cluster{"Target.X::12":refnum<vi>, "Target.Y::12":refnum<vi>}
  T32 = cluster{"Target.X::9":refnum<vi>, "Target.Y::9":refnum<vi>}
  T33 = cluster{"Target.X::10":refnum<vi>, "Target.Y::10":refnum<vi>}
  T34 = cluster{"Target.X::11":refnum<vi>, "Target.Y::11":refnum<vi>}
  T35 = cluster{"Target.X::12":refnum<vi>, "Target.Y::12":refnum<vi>}[]
  T36 = cluster{"Left":dbl, "Top":dbl, "Right":dbl, "Bottom":dbl}
  T37 = cluster{"Core":cluster{"Current VI Reference":refnum<vi>, "Close Panel on Exit?":bool}, "detection para":T3[], "thresholds":cluster{"Lower value":sgl, "Upper value":sgl}[], "Centroid X":dbl[][], "Centroid Y":dbl[][], "img to avg":i32, "Mean Centroid X":dbl[][], "Mean Centroid Y":dbl[][], "Offset X":dbl[][], "Offset Y":dbl[][], "Offset X stats ":dbl[][], "Offset Y stats ":dbl[][], "Size":dbl[][], "Mean Size":dbl[][], "Time":timestamp[][], "move properties":T2[], "active axis refs 2":cluster{"Ref X":refnum<vi>, "Ref Y":refnum<vi>}[], "active ccd":i32, "Feedback global":bool, "Motor X":dbl[][], "Motor Y":dbl[][], "active cams":string[], "Data Value Reference out":refnum<k34>, "active man refs":cluster{"Ref X":refnum<vi>, "Ref Y":refnum<vi>}, "detected":bool[], "speedmode X":bool[], "speedmode Y":bool[], "steps speed X":dbl[], "steps speed Y":dbl[]}
  T38 = cluster{"Current VI Reference":refnum<vi>, "Close Panel on Exit?":bool}
  T39 = cluster{"appended array":timestamp[], "appended array":dbl[]}
  T40 = cluster{"appended array":timestamp[], "appended array":dbl[]}[]
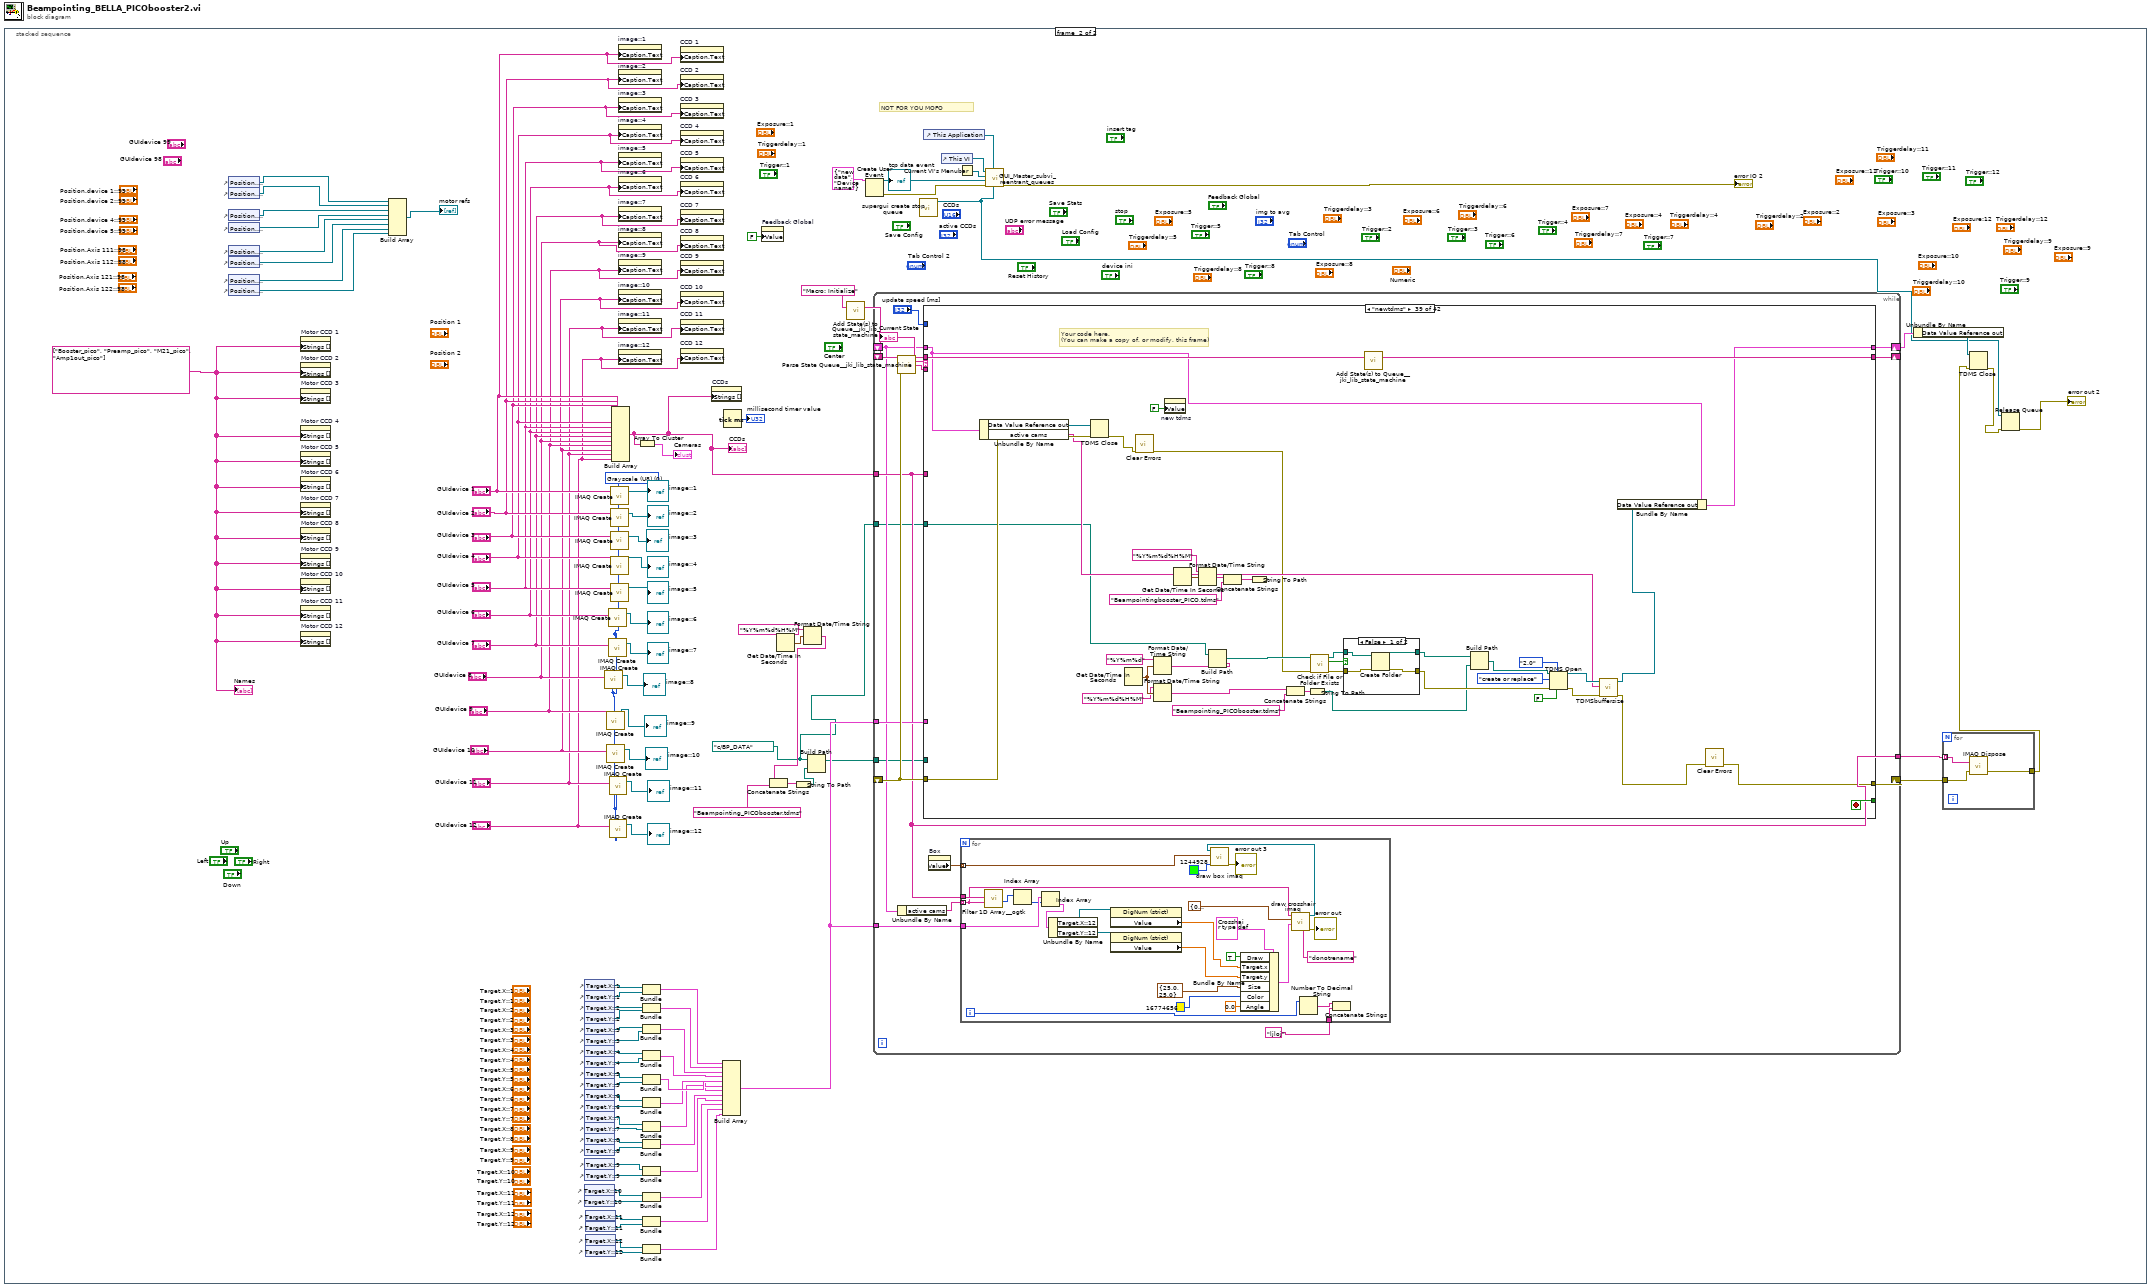
[diagram p0: block diagram]
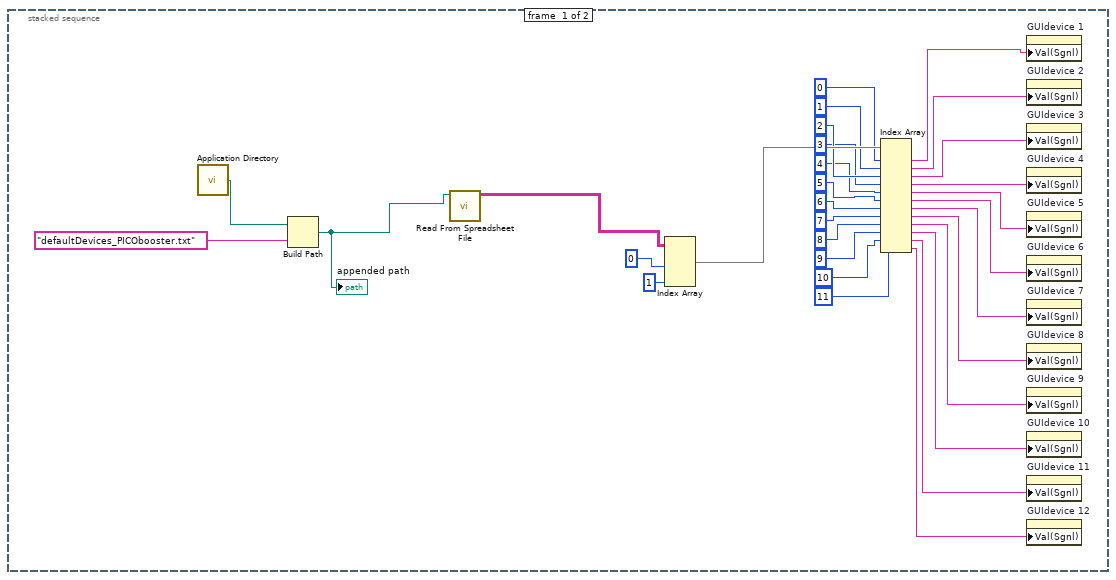
[diagram p2: hidden frame]
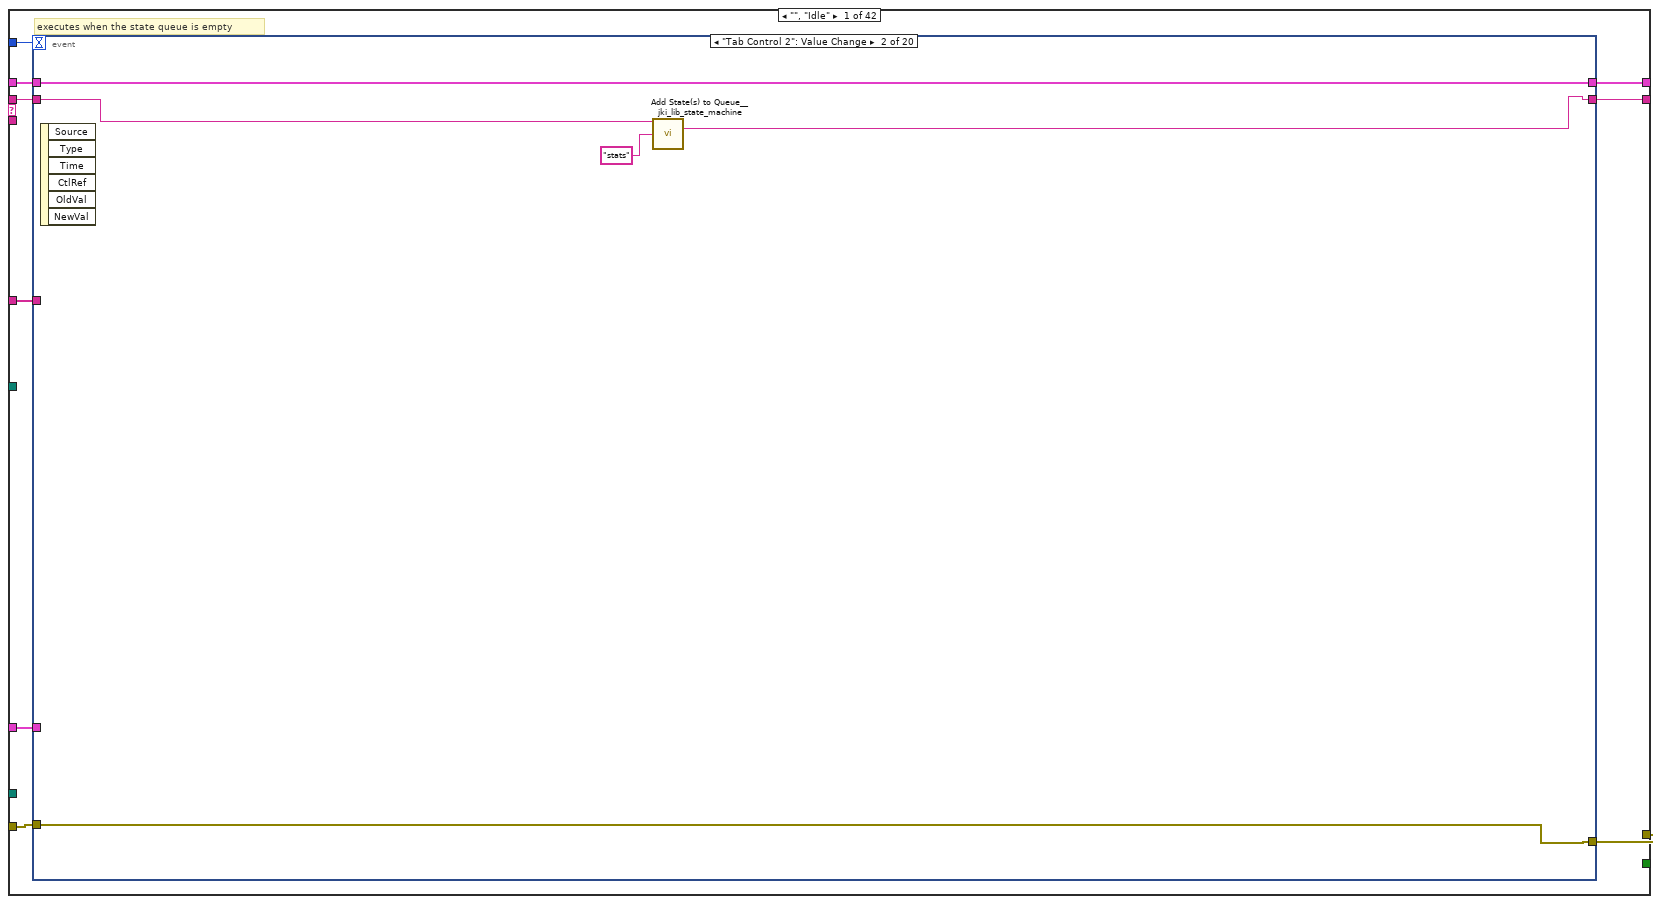
[diagram p3: hidden frame]
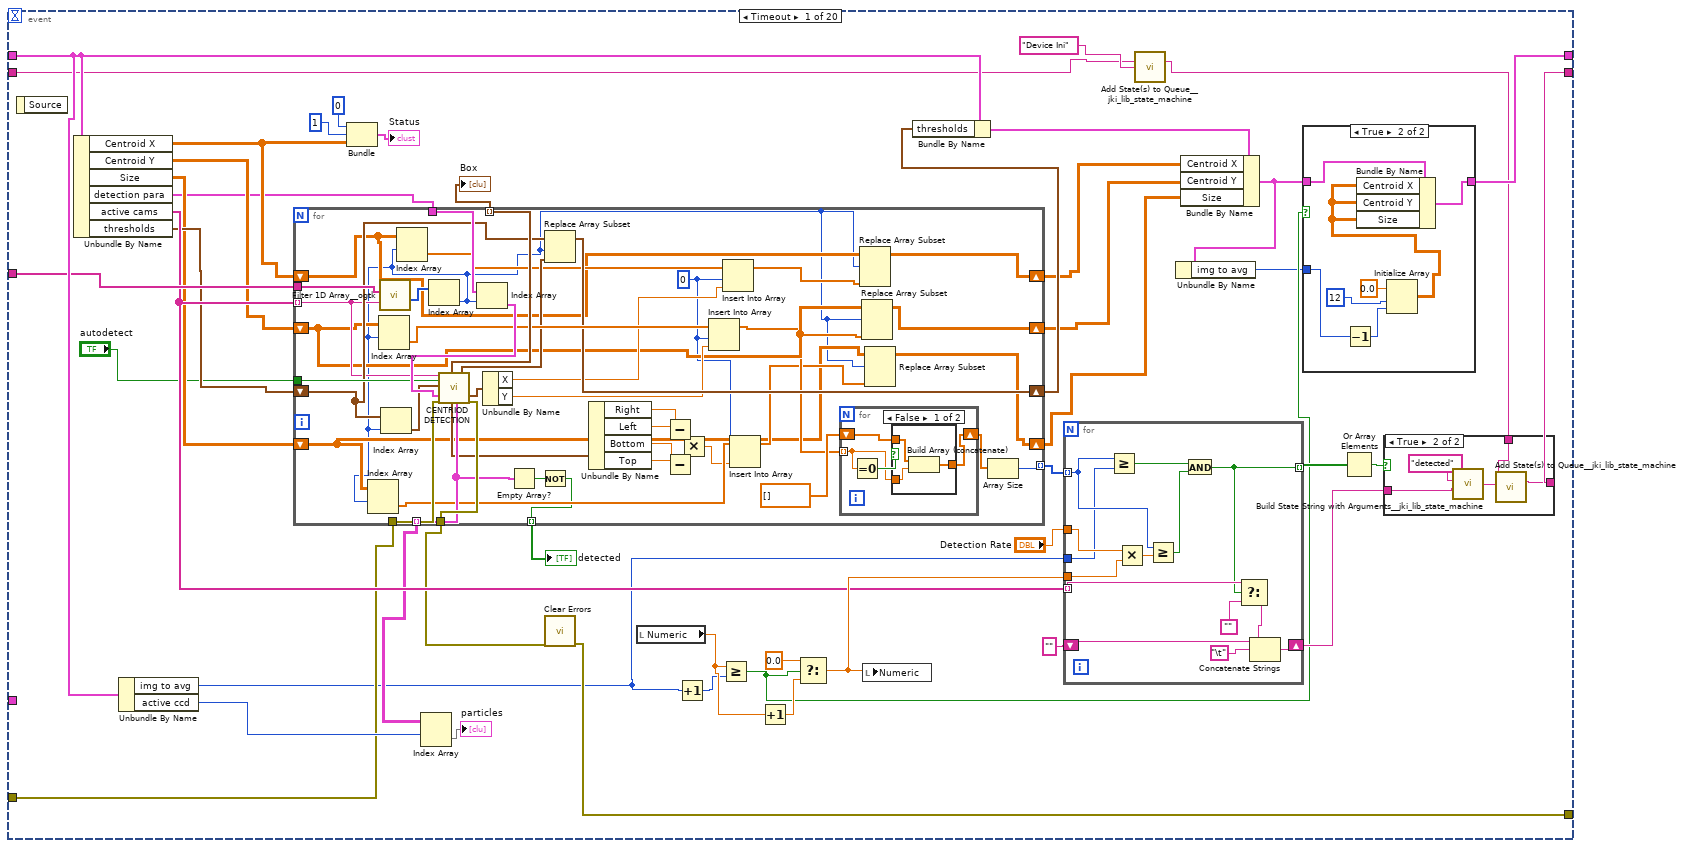
[diagram p4: hidden frame]
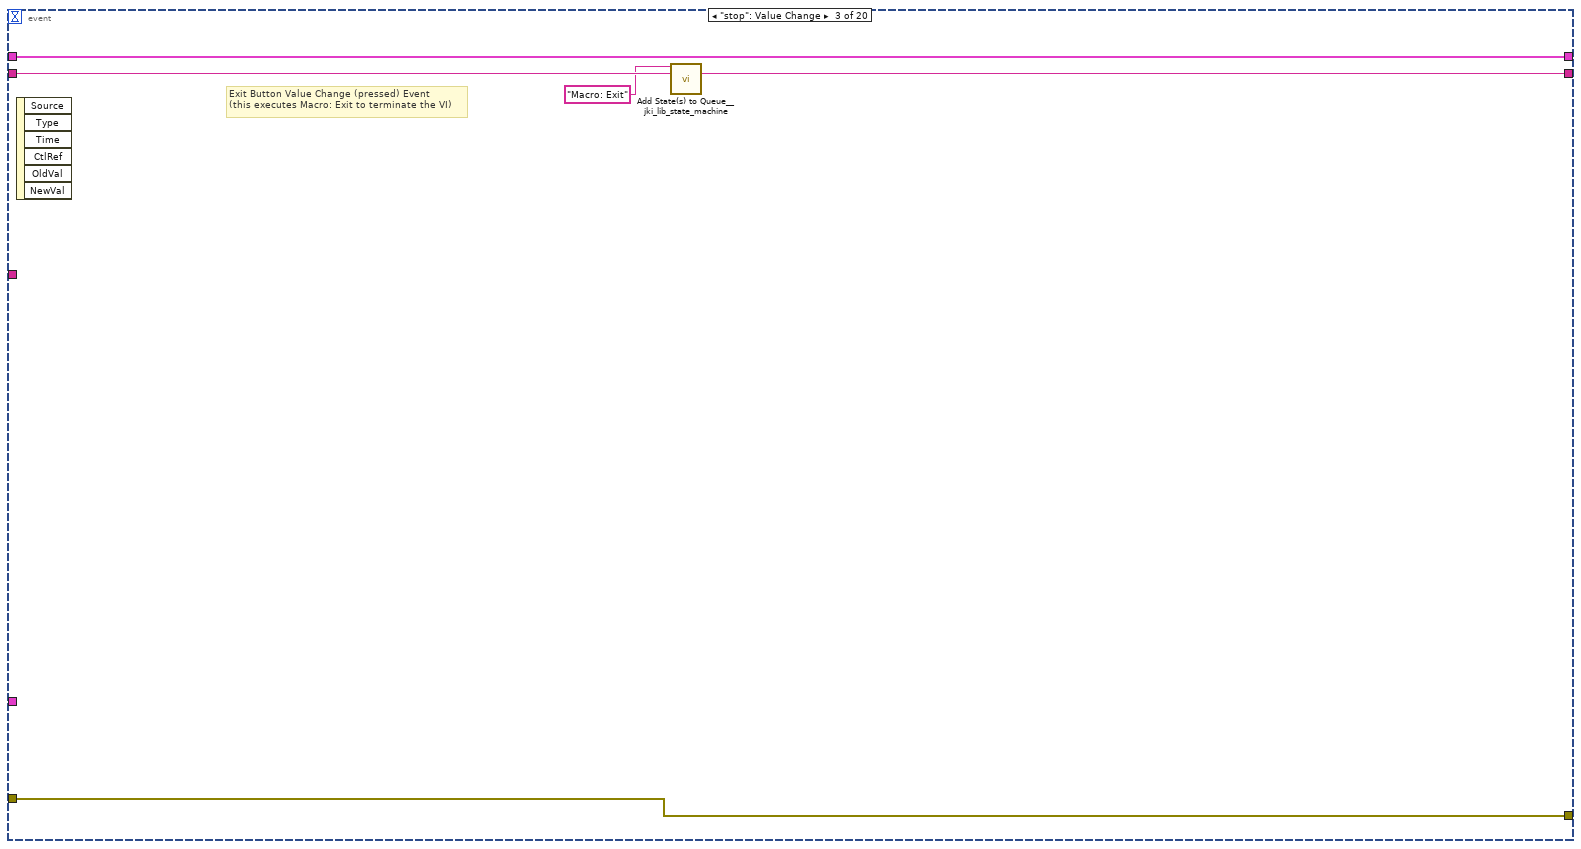
[diagram p8: hidden frame]
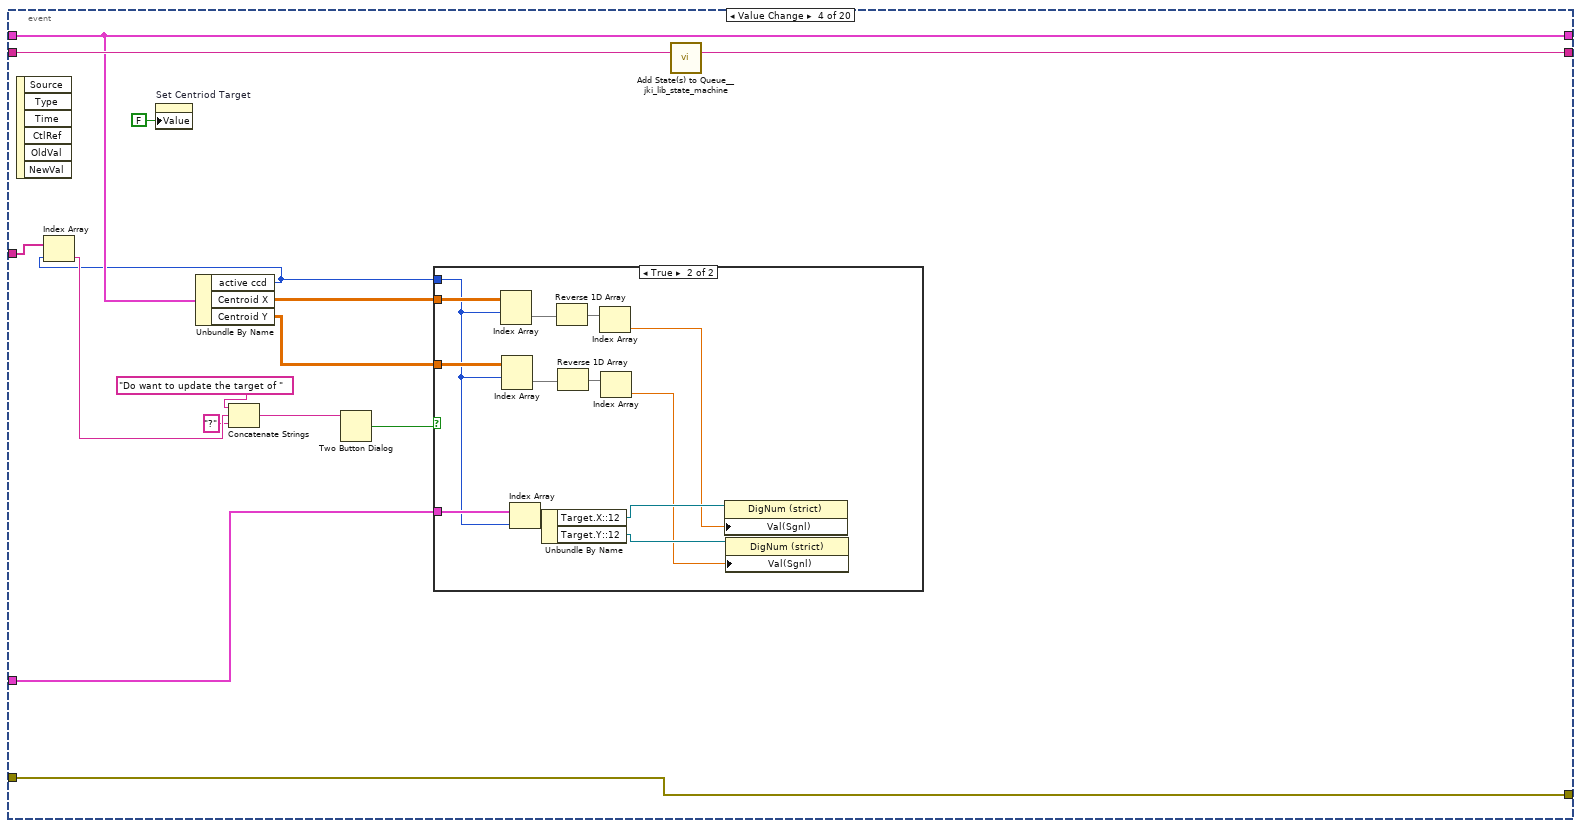
[diagram p9: hidden frame]
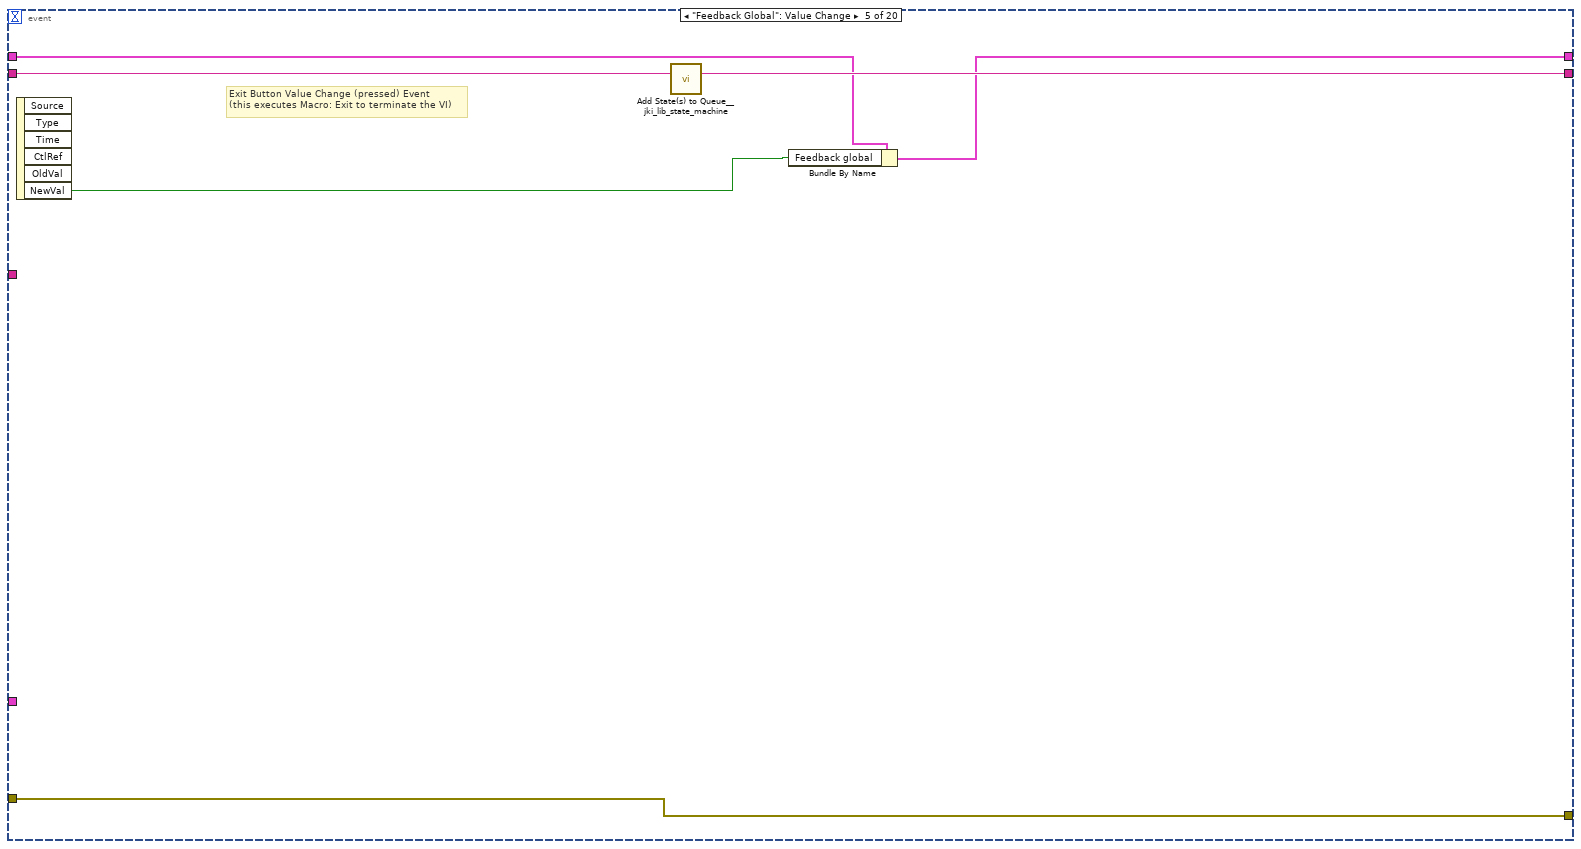
[diagram p11: hidden frame]
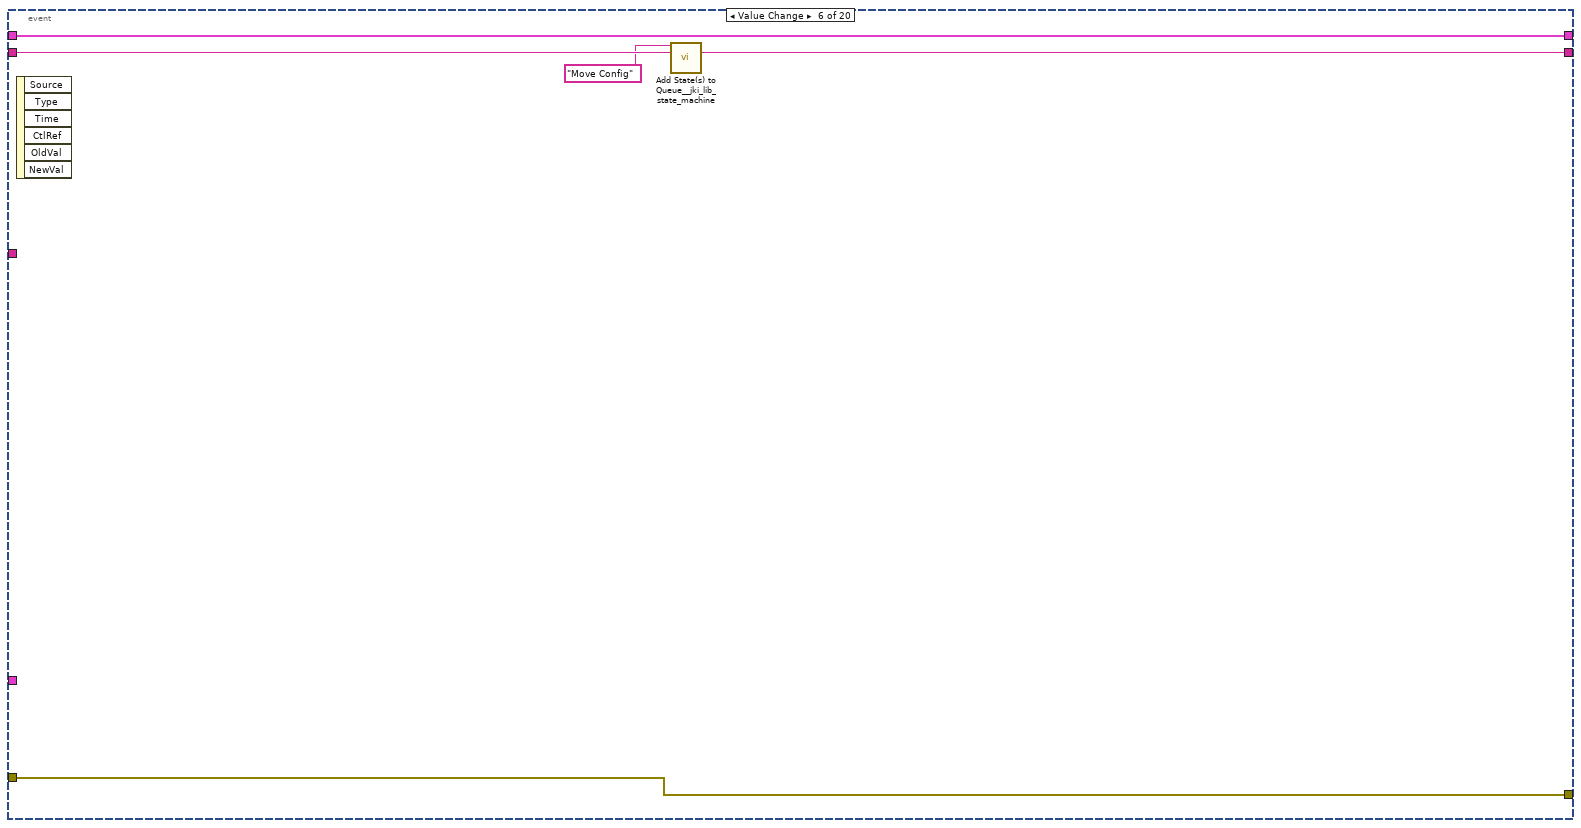
[diagram p12: hidden frame]
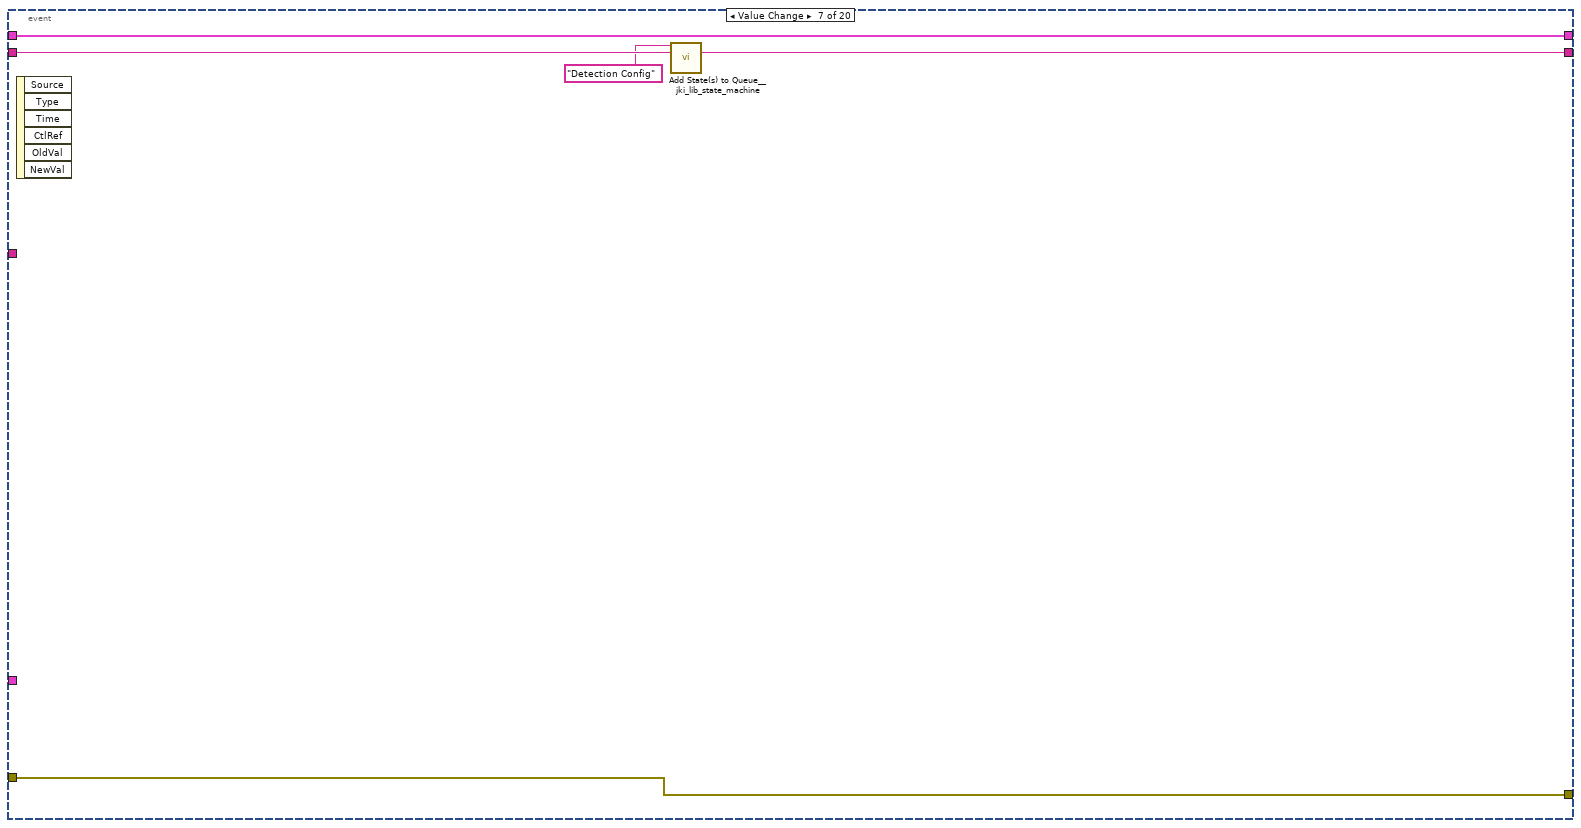
[diagram p13: hidden frame]
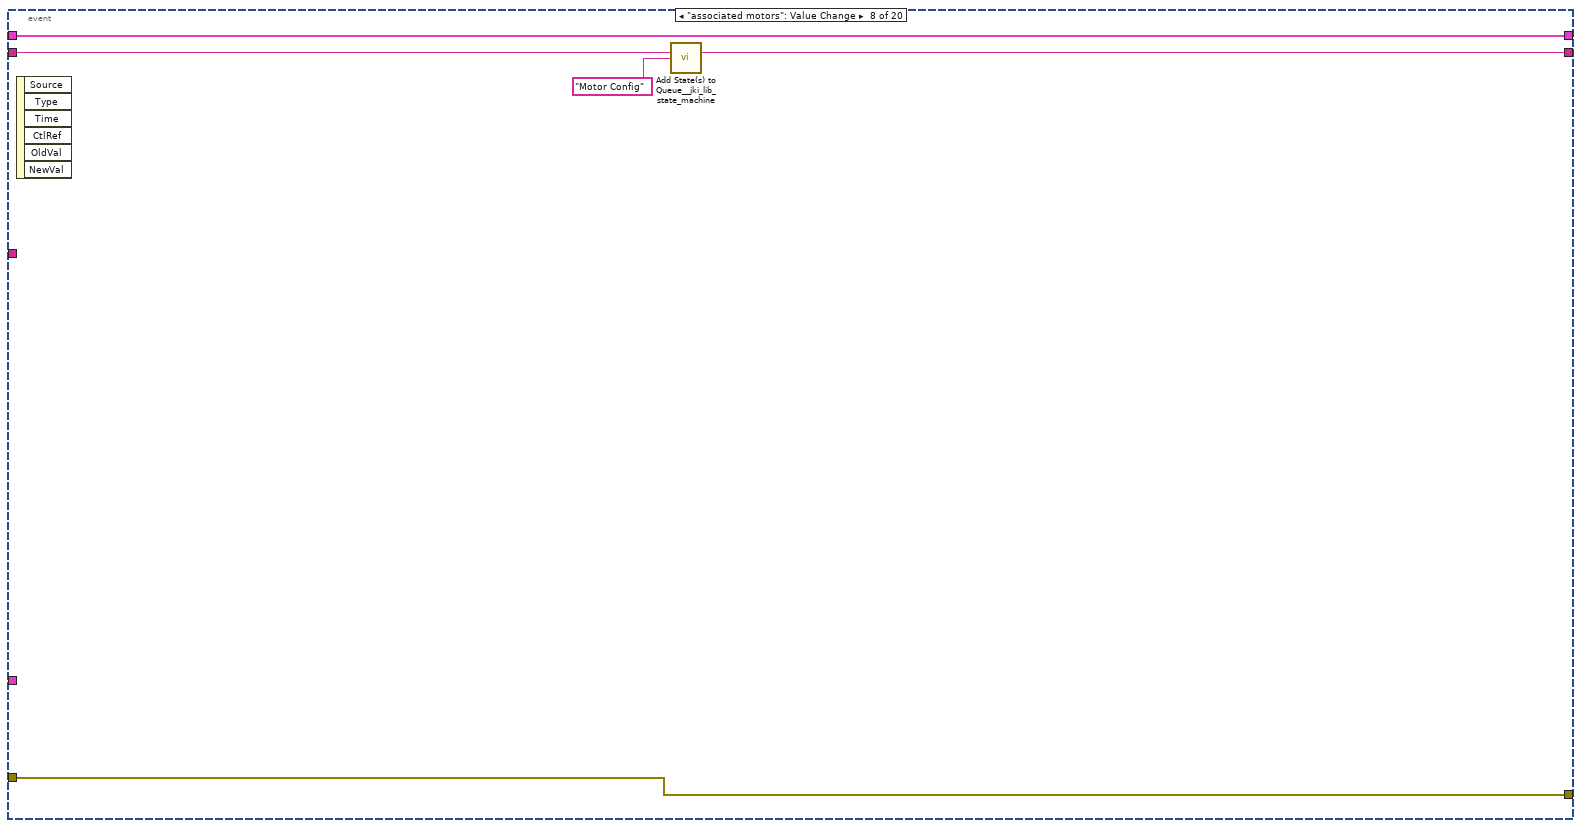
[diagram p14: hidden frame]
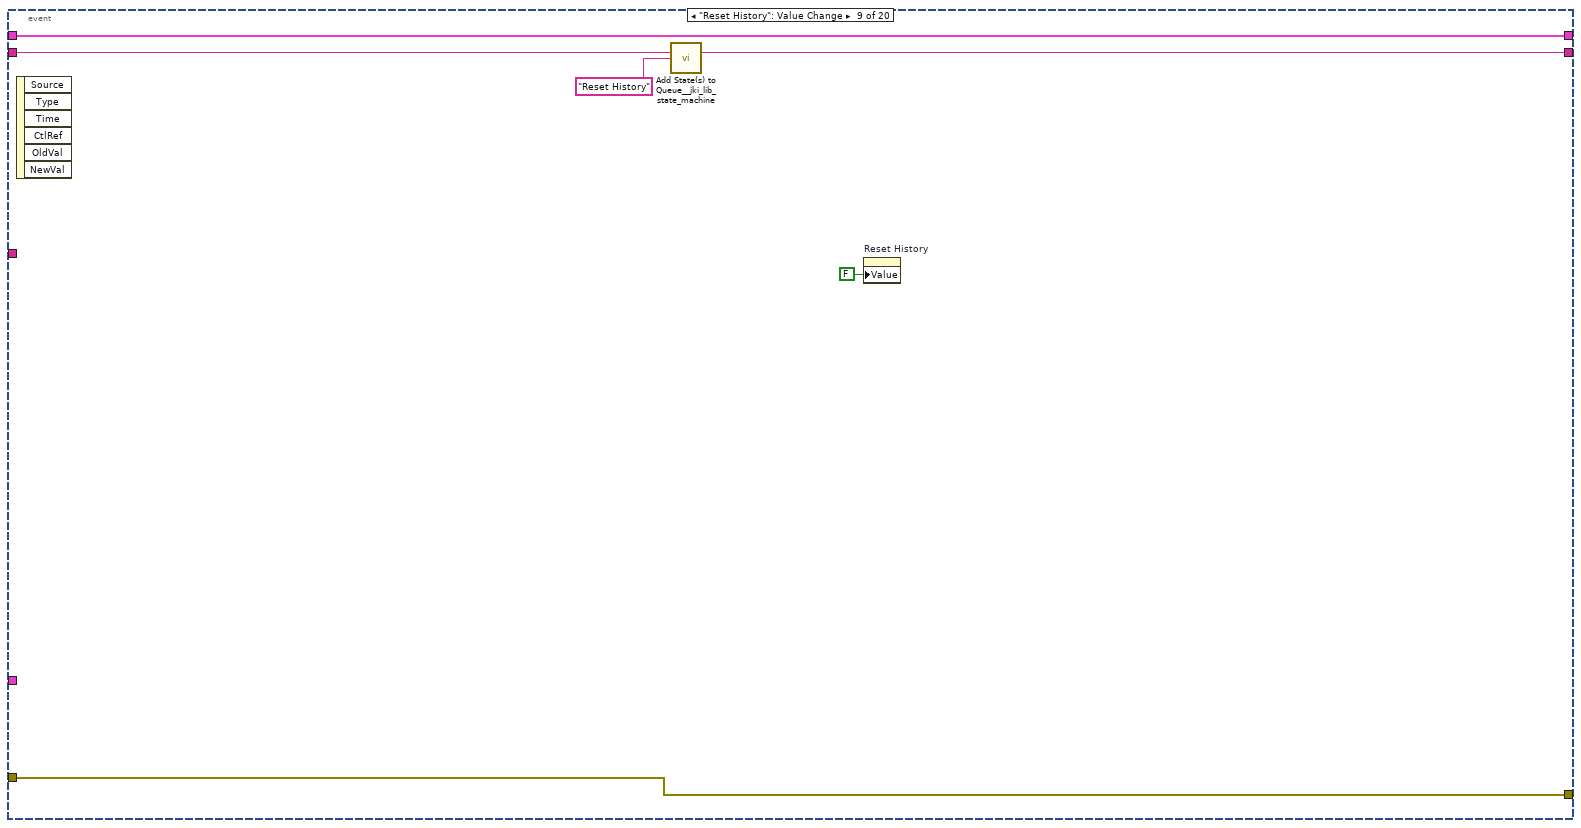
[diagram p15: hidden frame]
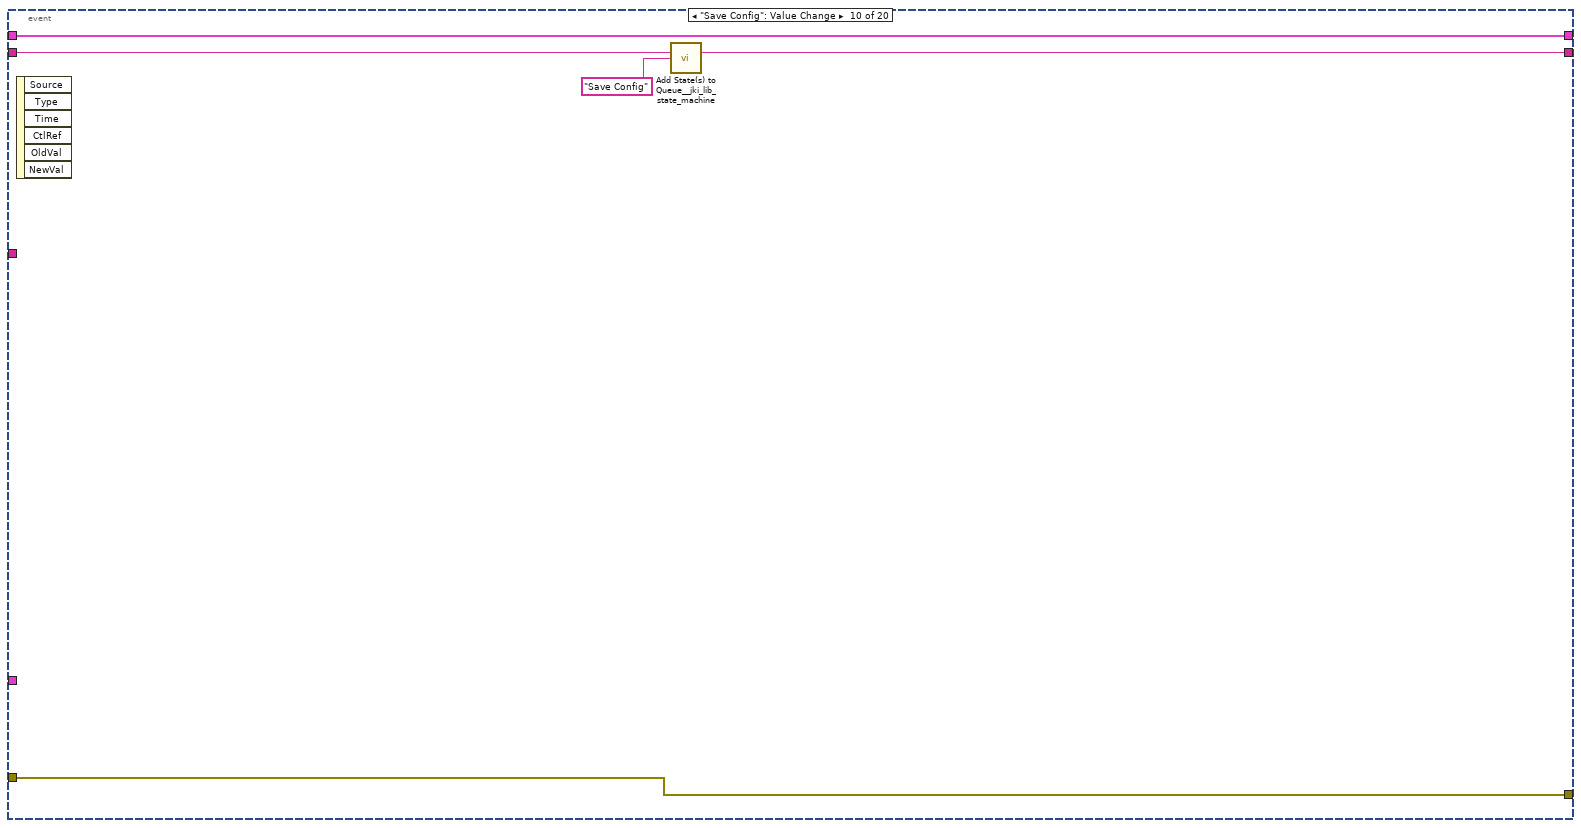
[diagram p16: hidden frame]
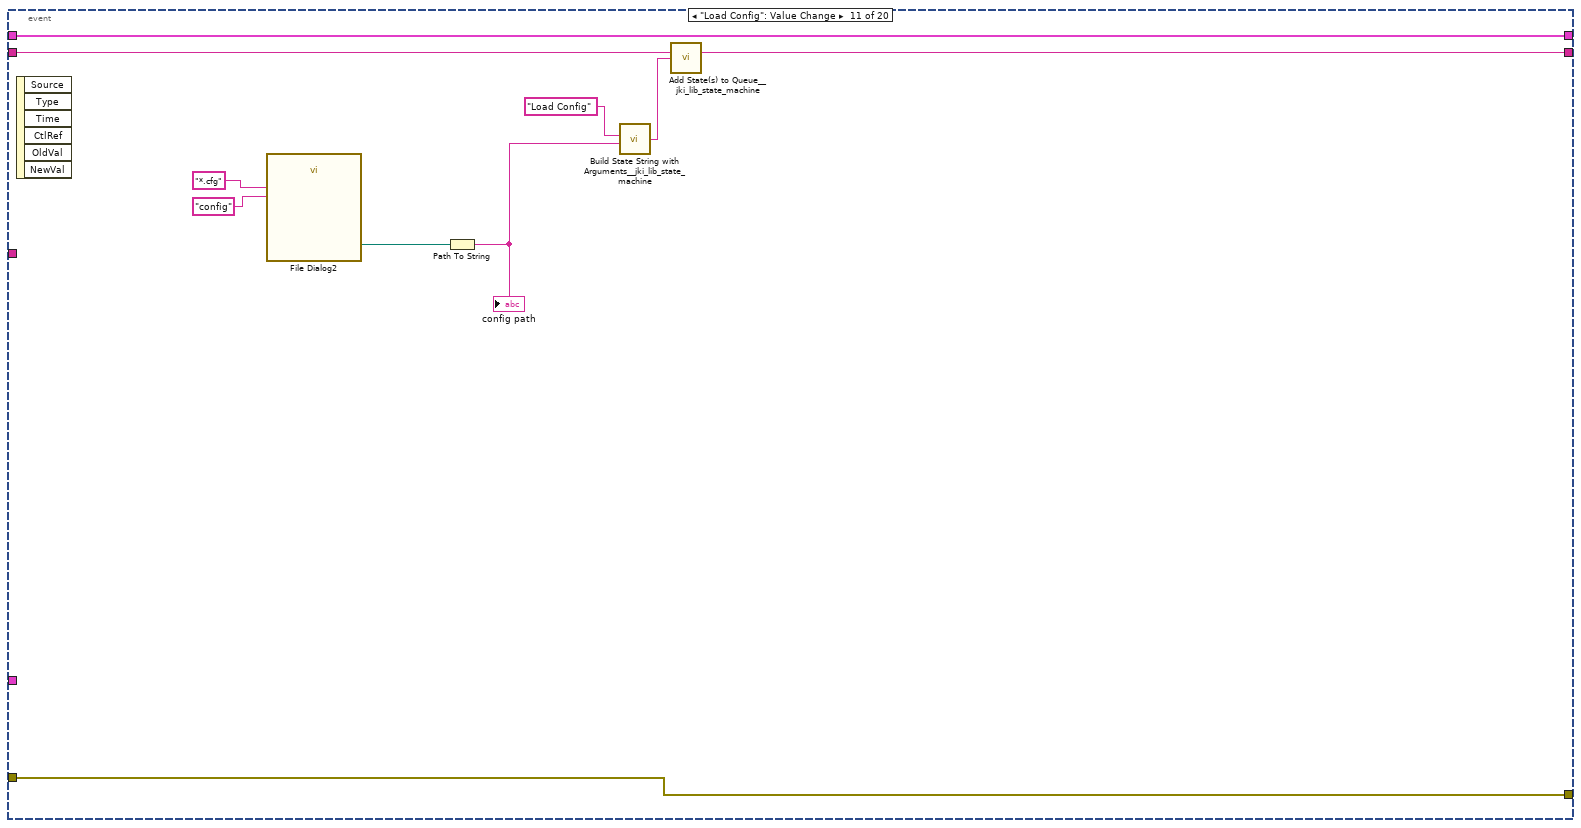
[diagram p17: hidden frame]
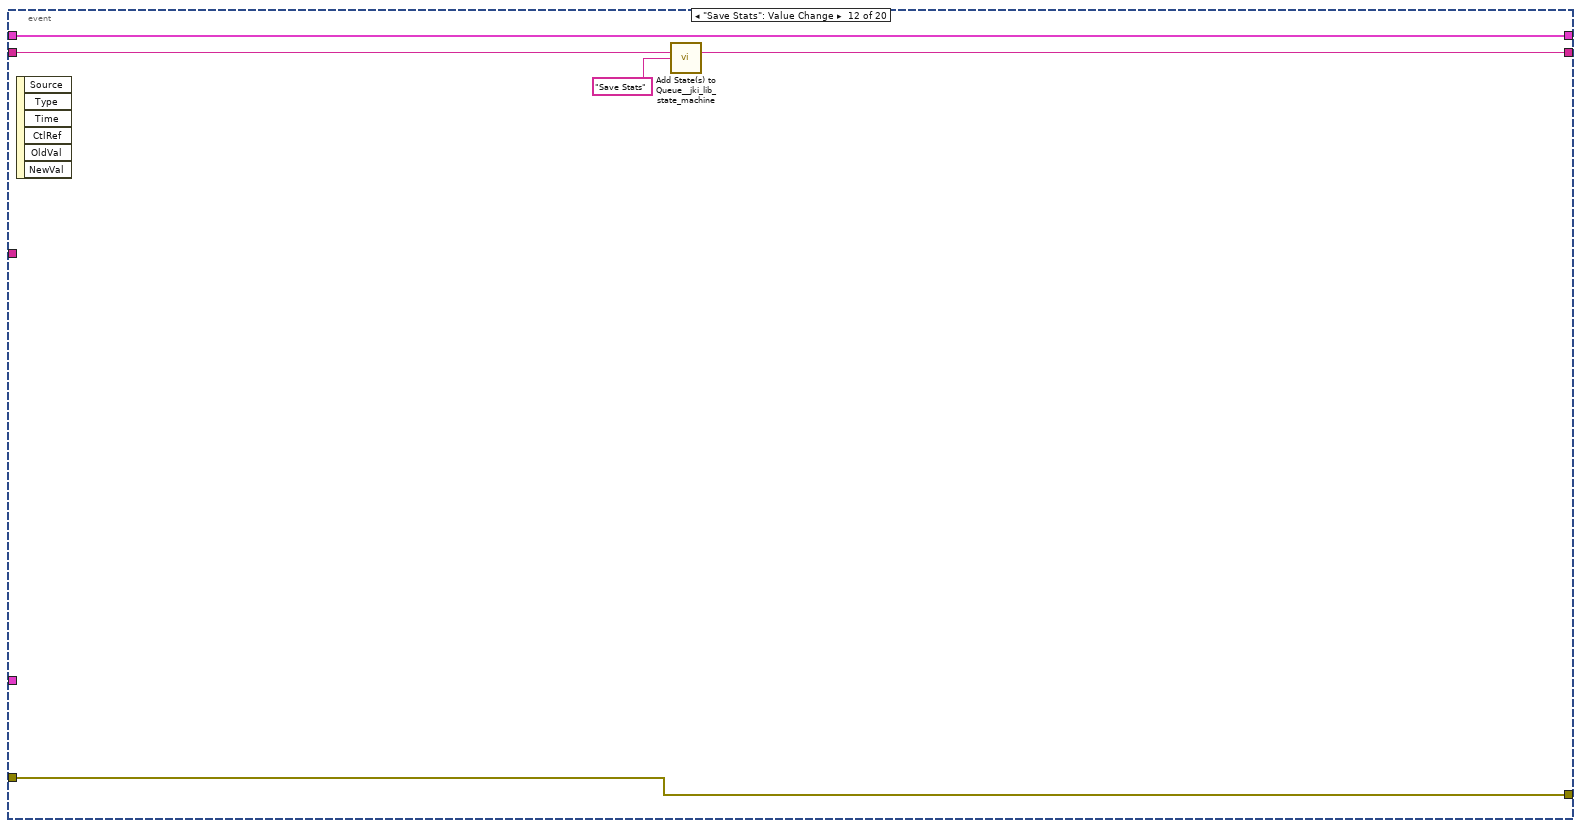
[diagram p18: hidden frame]
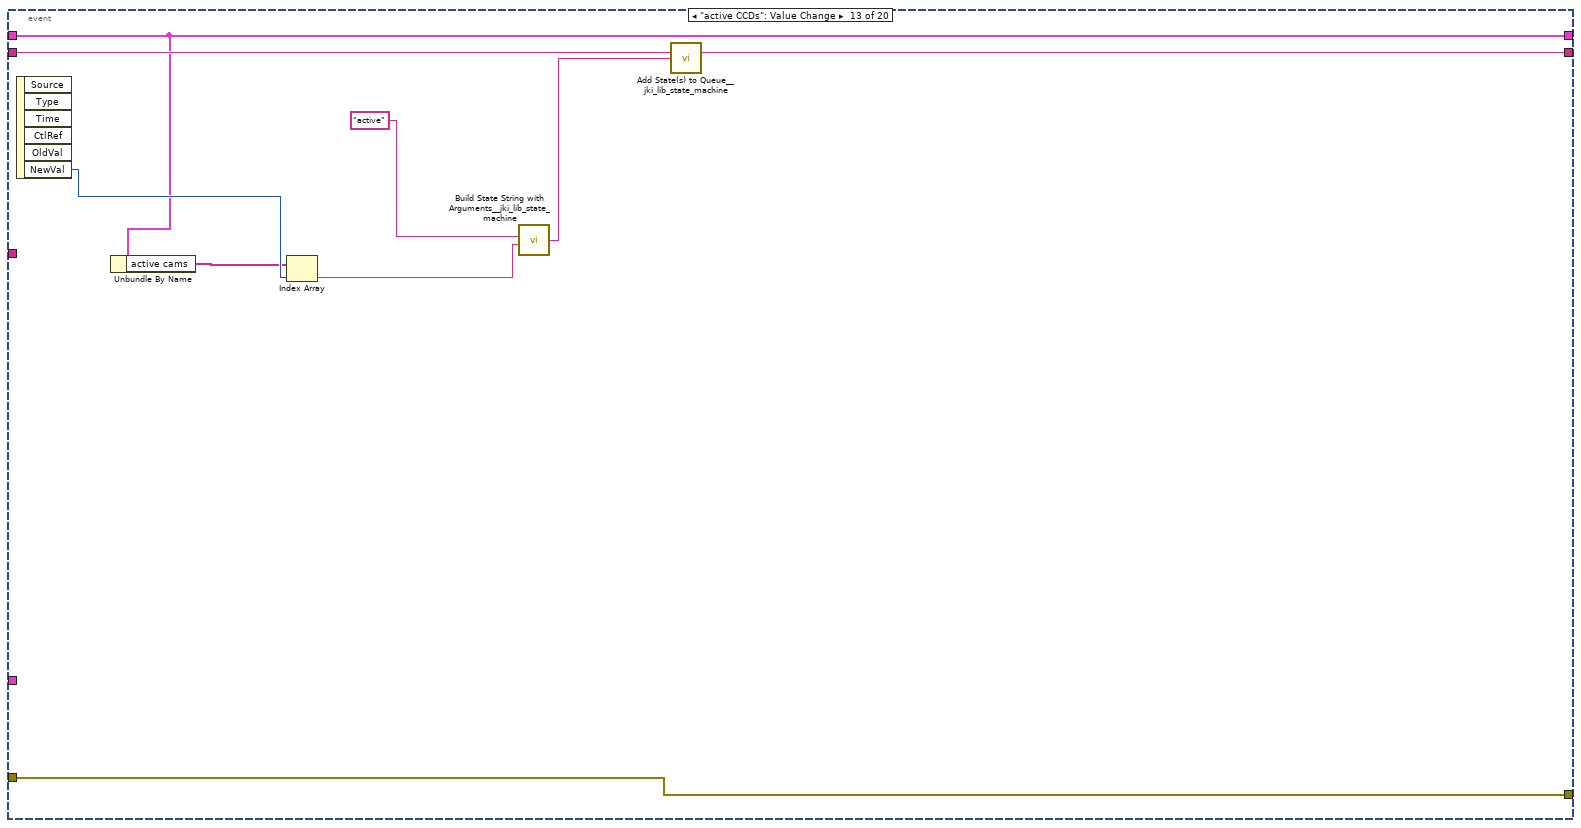
[diagram p19: hidden frame]
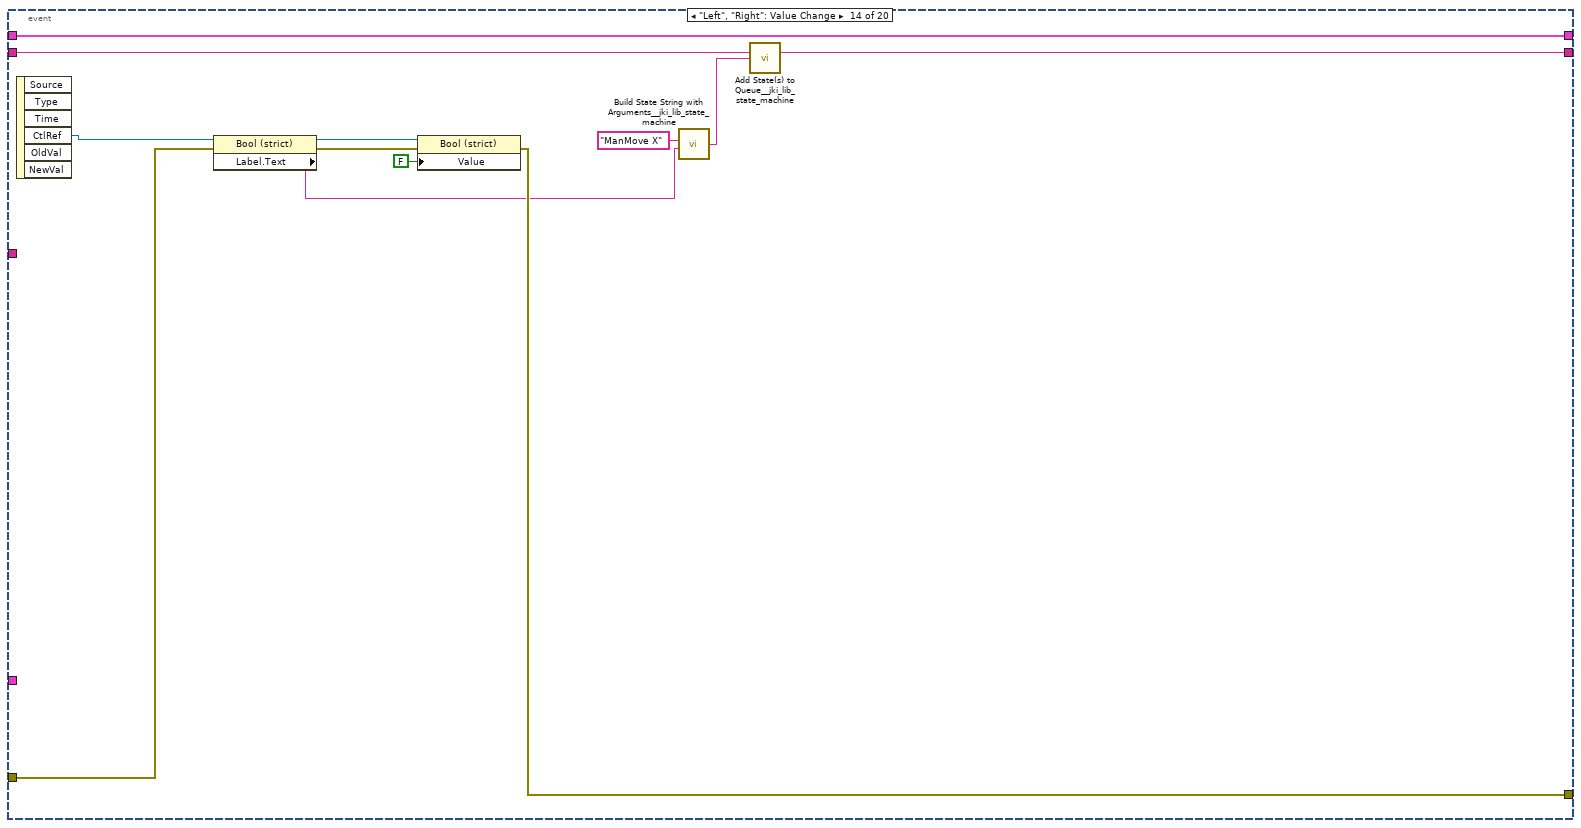
[diagram p20: hidden frame]
diagram:
  n1 = stacked-sequence {
    frame #0 {
      n2 = call <vilib>:"Application Directory.vi"() -> ("Application Directory"=w31:path)
      n3 = Build Path(base path=w31, name or relative path="defaultDevices_PICObooster.txt") -> (appended path=w29:path)
      "appended path" <- w29
      n4 = call-poly <vilib>:"Read From Spreadsheet File.vi"("file path (dialog if empty)"=w29) -> ("all rows"=w28:string[][])  [unwired: 6 in, 4 out]
      n5 = Index Array(array=w28, index (col) #1=0 ("disabled index (col)"), index (col) #2=1 ("index (col)")) -> (element #1=w25:string[])  [unwired: 2 in, 1 out]
      n6 = Index Array(array=w25, index #1=0 ("index"), index #2=1 ("index"), index #3=2 ("index"), index #4=3 ("index"), index #5=4 ("index"), index #6=5 ("index"), index #7=6 ("index"), index #8=7 ("index"), index #9=8 ("index"), index #10=9 ("index"), index #11=10 ("index"), index #12=11 ("index")) -> (element #1=w12:string, element #2=w11:string, element #3=w10:string, element #4=w9:string, element #5=w8:string, element #6=w7:string, element #7=w6:string, element #8=w5:string, element #9=w4:string, element #10=w3:string, element #11=w2:string, element #12=w1:string)
      n7 = property on="GUIdevice 1" class="Str"("Val(Sgnl)"=w12) -> ()  [unwired: 2 in, 2 out]
      n8 = property on="GUIdevice 2" class="Str"("Val(Sgnl)"=w11) -> ()  [unwired: 2 in, 2 out]
      n9 = property on="GUIdevice 3" class="Str"("Val(Sgnl)"=w10) -> ()  [unwired: 2 in, 2 out]
      n10 = property on="GUIdevice 4" class="Str"("Val(Sgnl)"=w9) -> ()  [unwired: 2 in, 2 out]
      n11 = property on="GUIdevice 5" class="Str"("Val(Sgnl)"=w8) -> ()  [unwired: 2 in, 2 out]
      n12 = property on="GUIdevice 6" class="Str"("Val(Sgnl)"=w7) -> ()  [unwired: 2 in, 2 out]
      n13 = property on="GUIdevice 7" class="Str"("Val(Sgnl)"=w6) -> ()  [unwired: 2 in, 2 out]
      n14 = property on="GUIdevice 8" class="Str"("Val(Sgnl)"=w5) -> ()  [unwired: 2 in, 2 out]
      n15 = property on="GUIdevice 9" class="Str"("Val(Sgnl)"=w4) -> ()  [unwired: 2 in, 2 out]
      n16 = property on="GUIdevice 10" class="Str"("Val(Sgnl)"=w3) -> ()  [unwired: 2 in, 2 out]
      n17 = property on="GUIdevice 11" class="Str"("Val(Sgnl)"=w2) -> ()  [unwired: 2 in, 2 out]
      n18 = property on="GUIdevice 12" class="Str"("Val(Sgnl)"=w1) -> ()  [unwired: 2 in, 2 out]
    }
    frame #1 {
      w55 = path "c:/BP_DATA" ("base path")
      w57 = string[] ["Booster_pico", "Preamp_pico", "M21_pico", "Amp1out_pico"] ("elements")
      w58 = T21 0 items=["Grayscale (U8)", "Grayscale (I16)", "Grayscale (SGL)", "Complex (CSG)", "RGB (U32)", "HSL (U32)", "RGB (U64)", "Grayscale (U16)"] ("Image Type")
      # "NOT FOR YOU MOFO"
      n19 = control-ref of="Position.device 1::99"() -> (w51:refnum<vi>)
      n20 = control-ref of="Position.device 2::99"() -> (w50:refnum<vi>)
      n21 = control-ref of="Position.device 4::99"() -> (w49:refnum<vi>)
      n22 = control-ref of="Position.device 5::99"() -> (w48:refnum<vi>)
      n23 = control-ref of="Position.Axis 111::98"() -> (w47:refnum<vi>)
      n24 = control-ref of="Position.Axis 112::98"() -> (w46:refnum<vi>)
      n25 = control-ref of="Position.Axis 121::98"() -> (w45:refnum<vi>)
      n26 = control-ref of="Position.Axis 122::98"() -> (w44:refnum<vi>)
      n27 = property on="Motor CCD 1" class="Ring (strict)"("Strings []"=w57) -> ()  [unwired: 2 in, 2 out]
      n28 = property on="Motor CCD 2" class="Ring (strict)"("Strings []"=w57) -> ()  [unwired: 2 in, 2 out]
      n29 = property on="Motor CCD 3" class="Ring (strict)"("Strings []"=w57) -> ()  [unwired: 2 in, 2 out]
      n30 = property on="Motor CCD 4" class="Ring (strict)"("Strings []"=w57) -> ()  [unwired: 2 in, 2 out]
      n31 = property on="Motor CCD 5" class="Ring (strict)"("Strings []"=w57) -> ()  [unwired: 2 in, 2 out]
      n32 = property on="Motor CCD 6" class="Ring (strict)"("Strings []"=w57) -> ()  [unwired: 2 in, 2 out]
      n33 = property on="Motor CCD 7" class="Ring (strict)"("Strings []"=w57) -> ()  [unwired: 2 in, 2 out]
      n34 = property on="Motor CCD 8" class="Ring (strict)"("Strings []"=w57) -> ()  [unwired: 2 in, 2 out]
      n35 = property on="Motor CCD 9" class="Ring (strict)"("Strings []"=w57) -> ()  [unwired: 2 in, 2 out]
      n36 = property on="Motor CCD 10" class="Ring (strict)"("Strings []"=w57) -> ()  [unwired: 2 in, 2 out]
      n37 = property on="Motor CCD 11" class="Ring (strict)"("Strings []"=w57) -> ()  [unwired: 2 in, 2 out]
      n38 = property on="Motor CCD 12" class="Ring (strict)"("Strings []"=w57) -> ()  [unwired: 2 in, 2 out]
      n39 = Build Array(w51, w50, w49, w48, w47, w46, w45, w44) -> (→"motor refs":refnum<vi>[])
      n40 = control-ref of="Target.X::1"() -> (w111:refnum<vi>)
      n41 = control-ref of="Target.Y::1"() -> (w110:refnum<vi>)
      n42 = control-ref of="Target.X::2"() -> (w109:refnum<vi>)
      n43 = control-ref of="Target.Y::2"() -> (w108:refnum<vi>)
      n44 = control-ref of="Target.X::3"() -> (w107:refnum<vi>)
      n45 = control-ref of="Target.Y::3"() -> (w106:refnum<vi>)
      n46 = control-ref of="Target.X::4"() -> (w105:refnum<vi>)
      n47 = control-ref of="Target.Y::4"() -> (w104:refnum<vi>)
      n48 = control-ref of="Target.X::5"() -> (w103:refnum<vi>)
      n49 = control-ref of="Target.Y::5"() -> (w102:refnum<vi>)
      n50 = control-ref of="Target.X::6"() -> (w101:refnum<vi>)
      n51 = control-ref of="Target.Y::6"() -> (w100:refnum<vi>)
      n52 = control-ref of="Target.X::7"() -> (w99:refnum<vi>)
      n53 = control-ref of="Target.Y::7"() -> (w98:refnum<vi>)
      n54 = control-ref of="Target.X::8"() -> (w97:refnum<vi>)
      n55 = control-ref of="Target.Y::8"() -> (w96:refnum<vi>)
      n56 = control-ref of="Target.X::9"() -> (w74:refnum<vi>)
      n57 = control-ref of="Target.Y::9"() -> (w73:refnum<vi>)
      n58 = control-ref of="Target.X::10"() -> (w72:refnum<vi>)
      n59 = control-ref of="Target.Y::10"() -> (w71:refnum<vi>)
      n60 = control-ref of="Target.X::11"() -> (w70:refnum<vi>)
      n61 = control-ref of="Target.Y::11"() -> (w69:refnum<vi>)
      n62 = control-ref of="Target.X::12"() -> (w68:refnum<vi>)
      n63 = control-ref of="Target.Y::12"() -> (w67:refnum<vi>)
      n64 = call "IMAQ Create"("Image Name"="GUIdevice 8", "Image Type"=w58) -> ("New Image"=→"image::8":T9)  [unwired: 3 in, 1 out]
      n65 = call "IMAQ Create"("Image Name"="GUIdevice 9", "Image Type"=w58) -> ("New Image"=→"image::9":T9)  [unwired: 3 in, 1 out]
      n66 = call "IMAQ Create"("Image Name"="GUIdevice 10", "Image Type"=w58) -> ("New Image"=→"image::10":T9)  [unwired: 3 in, 1 out]
      n67 = call "IMAQ Create"("Image Name"="GUIdevice 6", "Image Type"=w58) -> ("New Image"=→"image::6":T9)  [unwired: 3 in, 1 out]
      n68 = call "IMAQ Create"("Image Name"="GUIdevice 7", "Image Type"=w58) -> ("New Image"=→"image::7":T9)  [unwired: 3 in, 1 out]
      n69 = call "IMAQ Create"("Image Name"="GUIdevice 11", "Image Type"=w58) -> ("New Image"=→"image::11":T9)  [unwired: 3 in, 1 out]
      n70 = call "IMAQ Create"("Image Name"="GUIdevice 12", "Image Type"=w58) -> ("New Image"=→"image::12":T9)  [unwired: 3 in, 1 out]
      n71 = call "IMAQ Create"("Image Name"="GUIdevice 2") -> ("New Image"=→"image::2":T9)  [unwired: 4 in, 1 out]
      n72 = call "IMAQ Create"("Image Name"="GUIdevice 4", "Image Type"=w58) -> ("New Image"=→"image::4":T9)  [unwired: 3 in, 1 out]
      n73 = call "IMAQ Create"("Image Name"="GUIdevice 1", "Image Type"=w58) -> ("New Image"=→"image::1":T9)  [unwired: 3 in, 1 out]
      n74 = call "IMAQ Create"("Image Name"="GUIdevice 3", "Image Type"=w58) -> ("New Image"=→"image::3":T9)  [unwired: 3 in, 1 out]
      n75 = call "IMAQ Create"("Image Name"="GUIdevice 5", "Image Type"=w58) -> ("New Image"=→"image::5":T9)  [unwired: 3 in, 1 out]
      n76 = Build Array("GUIdevice 1", "GUIdevice 2", "GUIdevice 3", "GUIdevice 4", "GUIdevice 5", "GUIdevice 6", "GUIdevice 7", "GUIdevice 8", "GUIdevice 9", "GUIdevice 10", "GUIdevice 11", "GUIdevice 12") -> (w85:string[])
      "CCDs" <- w85
      n77 = property on="image::1" class="ImageControl"("Caption.Text"="GUIdevice 1") -> ()  [unwired: 2 in, 2 out]
      n78 = property on="image::2" class="ImageControl"("Caption.Text"="GUIdevice 2") -> ()  [unwired: 2 in, 2 out]
      n79 = property on="image::3" class="ImageControl"("Caption.Text"="GUIdevice 3") -> ()  [unwired: 2 in, 2 out]
      n80 = property on="image::4" class="ImageControl"("Caption.Text"="GUIdevice 4") -> ()  [unwired: 2 in, 2 out]
      n81 = property on="image::5" class="ImageControl"("Caption.Text"="GUIdevice 5") -> ()  [unwired: 2 in, 2 out]
      n82 = property on="image::6" class="ImageControl"("Caption.Text"="GUIdevice 6") -> ()  [unwired: 2 in, 2 out]
      n83 = property on="image::7" class="ImageControl"("Caption.Text"="GUIdevice 7") -> ()  [unwired: 2 in, 2 out]
      n84 = property on="image::8" class="ImageControl"("Caption.Text"="GUIdevice 8") -> ()  [unwired: 2 in, 2 out]
      n85 = property on="image::9" class="ImageControl"("Caption.Text"="GUIdevice 9") -> ()  [unwired: 2 in, 2 out]
      n86 = property on="image::10" class="ImageControl"("Caption.Text"="GUIdevice 10") -> ()  [unwired: 2 in, 2 out]
      n87 = property on="image::11" class="ImageControl"("Caption.Text"="GUIdevice 11") -> ()  [unwired: 2 in, 2 out]
      n88 = property on="image::12" class="ImageControl"("Caption.Text"="GUIdevice 12") -> ()  [unwired: 2 in, 2 out]
      n89 = Array To Cluster(array=w85) -> (cluster=→"Cameras":T22)
      n90 = Bundle("Target.X::1"=w111, "Target.Y::1"=w110) -> (w95:T23)  [unwired: 1 in]
      n91 = Bundle("Target.X::2"=w109, "Target.Y::2"=w108) -> (w94:T24)  [unwired: 1 in]
      n92 = Bundle("Target.X::3"=w107, "Target.Y::3"=w106) -> (w93:T25)  [unwired: 1 in]
      n93 = Bundle("Target.X::4"=w105, "Target.Y::4"=w104) -> (w86:T26)  [unwired: 1 in]
      n94 = Bundle("Target.X::5"=w103, "Target.Y::5"=w102) -> (w92:T27)  [unwired: 1 in]
      n95 = Bundle("Target.X::6"=w101, "Target.Y::6"=w100) -> (w91:T28)  [unwired: 1 in]
      n96 = Bundle("Target.X::7"=w99, "Target.Y::7"=w98) -> (w90:T29)  [unwired: 1 in]
      n97 = Bundle("Target.X::8"=w97, "Target.Y::8"=w96) -> (w89:T30)  [unwired: 1 in]
      n98 = Bundle("Target.X::12"=w68, "Target.Y::12"=w67) -> (w63:T31)  [unwired: 1 in]
      n99 = Bundle("Target.X::9"=w74, "Target.Y::9"=w73) -> (w66:T32)  [unwired: 1 in]
      n100 = Bundle("Target.X::10"=w72, "Target.Y::10"=w71) -> (w65:T33)  [unwired: 1 in]
      n101 = Bundle("Target.X::11"=w70, "Target.Y::11"=w69) -> (w64:T34)  [unwired: 1 in]
      n102 = property on="CCD 1" class="XYGraph (strict)"("Caption.Text"="GUIdevice 1") -> ()  [unwired: 2 in, 2 out]
      n103 = property on="CCD 2" class="XYGraph (strict)"("Caption.Text"="GUIdevice 2") -> ()  [unwired: 2 in, 2 out]
      n104 = property on="CCD 3" class="XYGraph (strict)"("Caption.Text"="GUIdevice 3") -> ()  [unwired: 2 in, 2 out]
      n105 = property on="CCD 4" class="XYGraph (strict)"("Caption.Text"="GUIdevice 4") -> ()  [unwired: 2 in, 2 out]
      n106 = property on="CCD 5" class="XYGraph (strict)"("Caption.Text"="GUIdevice 5") -> ()  [unwired: 2 in, 2 out]
      n107 = property on="CCD 6" class="XYGraph (strict)"("Caption.Text"="GUIdevice 6") -> ()  [unwired: 2 in, 2 out]
      n108 = property on="CCD 7" class="XYGraph (strict)"("Caption.Text"="GUIdevice 7") -> ()  [unwired: 2 in, 2 out]
      n109 = property on="CCD 8" class="XYGraph (strict)"("Caption.Text"="GUIdevice 8") -> ()  [unwired: 2 in, 2 out]
      n110 = property on="CCD 9" class="XYGraph (strict)"("Caption.Text"="GUIdevice 9") -> ()  [unwired: 2 in, 2 out]
      n111 = property on="CCD 10" class="XYGraph (strict)"("Caption.Text"="GUIdevice 10") -> ()  [unwired: 2 in, 2 out]
      n112 = property on="CCD 11" class="XYGraph (strict)"("Caption.Text"="GUIdevice 11") -> ()  [unwired: 2 in, 2 out]
      n113 = property on="CCD 12" class="XYGraph (strict)"("Caption.Text"="GUIdevice 12") -> ()  [unwired: 2 in, 2 out]
      n114 = property on="CCDs" class="Ring (strict)"("Strings []"=w85) -> ()  [unwired: 2 in, 2 out]
      n115 = Build Array(w95, w94, w93, w86, w92, w91, w90, w89, w66, w65, w64, w63) -> (w88:T35)
      n116 = Tick Count (ms)() -> (millisecond timer value=→"millisecond timer value":u32)
      n117 = property on="Feedback Global" class="Bool (strict)"("Value"=FALSE ("Feedback Global")) -> ()  [unwired: 2 in, 2 out]
      n118 = Get Date/Time In Seconds() -> (seconds since 1Jan1904=w76:timestamp)
      n119 = Format Date/Time String(time format string (%c)="%Y%m%d%H%M", seconds (now)=w76) -> (date/time string=w75:string)  [unwired: 1 in]
      n120 = Concatenate Strings(w75, "Beampointing_PICObooster.tdms" ("string")) -> (w79:string)
      n121 = String To Path(string=w79) -> (path=w78:path)
      n122 = Build Path(base path=w55, name or relative path=w78) -> (appended path=w81:path)
      n123 = call <vilib>:"Add State(s) to Queue__jki_lib_state_machine.vi"("State(s) in (\"\")"="Macro: Initialize") -> ("States Out"=w118:string)  [unwired: 14 in]
      n124 = Create User Event(user event datatype=T13 {"EventEnum"=enum."new data", "Device name"="Device name"} ("New Event")) -> (user event=w126:refnum<user-event>, error out=w128:errorcluster)  [unwired: 1 in]
      "tcp data event" <- w126
      n125 = while "JKI - String-Based Queued State Machine (Basic) v1.0" {
        shift-right: [w147] -> w84
        shift-left: _ -> [w140]
        shift-right: [w150] -> w112
        shift-left: _ -> [w146]
        shift-right: [w149] -> _
        shift-left: w118 -> [w151]
        tunnel: w88 -> [w144]
        tunnel: w85 -> [w142]
        tunnel: [w142] -> w113
        tunnel: w88 -> [w143]
        tunnel: w81 -> [w138]
        tunnel: w55 -> [w137]
        stop <- w148 stop-if-true
        n126 = Unbundle By Name(w140) -> ("active cams"=w139:string[])
        n127 = call <vilib>:"Parse State Queue__jki_lib_state_machine.vi"("State Queue"=w151, "Error In (no error)"=w146) -> ("Remaining States"=w153:string, "Current State"=w154:string, "Arguments"=w152:string)  [unwired: 11 in]
        "Current State" <- w154
        n128 = case shown="\"newtdms\"" w154 {
          selector: w154 -> [_ _ w466 _ _ _ _ _ _ _ _ _ _ _ _ _ _ _ _ _ _ _ _ _ _ _ _ _ _ _ _ _ _ _ _ _ _ _ _ _ _ _]
          tunnel: w153 -> [w189 w465 w470 w488 w494 w499 w503 w544 w560 w564 w568 w574 w585 w609 w618 w628 w632 w660 w780 w832 w862 w871 w893 w914 w918 w934 w1083 w1232 w1312 w1376 w1451 w1527 w1551 w1566 w1640 w1692 w1702 w1742 w1838 w1864 w1878 w1901]
          tunnel: w152 -> [_ _ _ _ _ _ _ _ _ _ _ w569 w580 _ _ _ _ w638 w733 _ w847 _ _ _ _ w935 _ w1211 w1298 w1362 w1430 w1521 _ _ _ _ _ _ _ _ w1882 _]
          tunnel: w140 -> [w187 w462 w468 w478 w491 w497 w500 _ w555 w561 w566 w572 w579 w606 w615 w620 w629 w654 w770 w830 w843 w867 w885 w907 w915 w923 w1062 w1205 w1308 w1372 w1428 w1523 w1548 w1563 w1636 w1689 w1699 w1716 w1836 w1861 w1881 w1892]
          tunnel: [w186 w463 w472 w486 errorcluster {"status"=FALSE, "code"=0, "source"=""} ("error out") w496 w501 w511 w557 w562 w565 w570 w582 w607 w616 w626 w630 w656 w736 w821 w851 w869 w891 w912 w916 w968 w1096 w1230 w1310 w1374 w1449 w1516 w1549 w1564 w1637 w1690 w1700 w1703 w1800 w1862 w1876 w1899] -> w150
          tunnel: w146 -> [w185 w463 w471 w486 w490 w496 w501 w512 w558 w562 w565 w571 w583 w607 w616 w626 w630 w657 w734 w822 w850 w869 w891 w912 w916 w968 w1096 w1230 w1310 w1374 w1449 w1517 w1549 w1564 w1638 w1690 w1700 w1705 w1834 w1862 w1876 w1899]
          tunnel: [w188 w464 w469 w487 w493 w498 w502 w543 w559 w563 w567 w573 w584 w608 w617 w627 w631 w648 w779 w831 w861 w870 w892 w913 w917 w939 w1097 w1231 w1311 w1375 w1450 w1526 w1550 w1565 w1639 w1691 w1701 w1741 w1837 w1863 w1877 w1900] -> w149
          tunnel: [_ _ _ _ _ TRUE _ _ _ _ _ _ _ _ _ _ _ _ _ _ _ _ _ _ _ _ _ _ _ _ _ _ _ _ _ _ _ _ _ _ _ _] -> w148
          tunnel: [w182 w462 w468 w477 w491 w497 w500 w513 w555 w561 w566 w572 w579 w606 w615 w620 w629 w659 w769 w830 w856 w866 w884 w906 w915 w961 w1064 w1205 w1308 w1372 w1428 w1525 w1548 w1563 w1636 w1688 w1699 w1716 w1835 w1861 w1880 w1891] -> w147
          tunnel: "update speed [ms]" -> [w184 _ _ _ _ _ _ _ _ _ _ _ _ _ _ _ _ _ _ _ _ _ _ _ _ _ _ _ _ _ _ _ _ _ _ _ _ _ _ _ _ _]
          tunnel: w144 -> [w181 _ _ _ _ _ _ _ _ _ _ _ _ _ _ _ _ _ _ _ _ _ _ _ _ w959 _ _ _ _ _ _ _ _ _ _ _ _ _ w1846 _ _]
          tunnel: w142 -> [w183 _ _ _ _ _ _ w508 _ _ _ _ _ _ _ _ _ w641 w768 _ w857 _ _ _ _ w927 w1063 w1229 _ _ w1448 w1522 _ w1553 _ _ _ w1715 _ _ _ _]
          tunnel: w138 -> [_ _ _ _ _ _ _ w510 _ _ _ _ _ _ _ _ _ w658 _ _ _ _ _ _ _ _ _ _ _ _ _ _ _ _ _ _ _ _ _ _ _ _]
          tunnel: w137 -> [_ _ _ _ _ _ _ _ _ _ _ _ _ _ _ _ _ _ _ _ _ _ _ _ _ _ _ _ _ _ _ _ _ _ _ _ _ _ w1806 _ _ _]
          frame "", "Idle" {
            # "executes when the state queue is empty"
            n129 = event shown="[1] \"Tab Control 2\": Value Change" {
              selector: _ -> [_ _ _ _ _ _ _ _ _ _ _ _ _ _ _ _ _ _ _ _]
              dyn-events: _ -> [_ _ _ _ _ _ _ _ _ _ _ _ _ _ _ _ _ _ _ _]
              timeout: w184 -> [_ _ _ _ _ _ _ _ _ _ _ _ _ _ _ _ _ _ _ _]
              tunnel: w189 -> [w192 w316 w323 w338 w357 w362 w367 w372 w378 w383 w393 w398 w407 w419 w431 w436 w441 w447 w451 w461]
              tunnel: [w219 w315 w322 w337 w356 w361 w366 w371 w377 w382 w392 w397 w406 w418 w430 w435 w440 w446 w449 w460] -> w188
              tunnel: w187 -> [w215 w318 w320 w334 w353 w359 w364 w369 w375 w380 w390 w395 w400 w417 w429 w434 w439 w445 w452 w458]
              tunnel: [w230 w314 w321 w336 w355 w360 w365 w370 w376 w381 w391 w396 w405 w412 w424 w433 w438 w444 w448 w459] -> w186
              tunnel: w185 -> [w206 w314 w321 w336 w355 w360 w365 w370 w376 w381 w391 w396 w405 w413 w425 w433 w438 w444 w448 w459]
              tunnel: [w218 w318 w320 w334 w352 w359 w364 w369 w375 w380 w390 w395 w400 w417 w429 w434 w439 w445 w452 w458] -> w182
              tunnel: w183 -> [w211 _ _ w330 _ _ _ _ _ _ _ _ _ _ _ _ _ _ _ _]
              tunnel: w181 -> [_ _ _ w332 _ _ _ _ _ _ _ _ _ _ _ _ _ _ _ _]
              event Timeout {
                n130 = event-data() -> ()  [unwired: 1 in, 1 out]
                n131 = Unbundle By Name(w215) -> ("Centroid X"=w212:dbl[][], "Centroid Y"=w209:dbl[][], "Size"=w207:dbl[][], "detection para"=w202:T3[], "active cams"=w210:string[], "thresholds"=w208:cluster{"Lower value":sgl, "Upper value":sgl}[])
                n132 = Unbundle By Name(w215) -> ("img to avg"=w190:i32, "active ccd"=w214:i32)
                n133 = for {
                  tunnel: w210 -> [w251] mode=indexing
                  tunnel: [w252] -> w197 mode=indexing
                  tunnel: w211 -> [w274]
                  tunnel: w202 -> [w272]
                  tunnel: [w235] -> w196 mode=indexing
                  tunnel: [w270] -> w205 mode=indexing
                  tunnel: [w268] -> w213 mode=indexing
                  tunnel: "autodetect" -> [w262]
                  tunnel: w206 -> [w275]
                  tunnel: [w276] -> w204
                  shift-right: [w259] -> w201
                  shift-left: w208 -> [w261]
                  shift-right: [w246] -> w200
                  shift-left: w212 -> [w248]
                  shift-right: [w242] -> w199
                  shift-left: w209 -> [w244]
                  shift-right: [w236] -> w198
                  shift-left: w207 -> [w238]
                  w240 = 0 ("index")
                  n134 = call-poly <userlib>:"Filter 1D Array__ogtk.vi"("items to filter"=w251, "array"=w274) -> ("filtered item indices"=w273:i32[])  [unwired: 4 in, 1 out]
                  n135 = Index Array(array=w273) -> (element=w237:i32)  [unwired: 1 in]
                  n136 = Index Array(array=w238, index (row)=w237) -> (element=w266:dbl[])  [unwired: 1 in]
                  n137 = Index Array(array=w244, index (row)=w237) -> (element=w267:dbl[])  [unwired: 1 in]
                  n138 = Index Array(array=w261, index=w237) -> (element=w265:cluster{"Lower value":sgl, "Upper value":sgl})
                  n139 = Index Array(array=w248, index (row)=w237) -> (element=w250:dbl[])  [unwired: 1 in]
                  n140 = Index Array(array=w272, index=w237) -> (element=w269:T3)
                  n141 = call "CENTRIOD DETECTION.vi"("Refnum in"=w251, "auto threshold"=w262, "Threshold Range In"=w265, "beam detection para"=w269, "error in (no error)"=w275) -> ("Bounding Rect"=w268:T36, "Particle Reports (Pixels)"=w270:T1, "Threshold Range Out"=w260:cluster{"Lower value":sgl, "Upper value":sgl}, "Centriod"=w277:cluster{"X":dbl, "Y":dbl}, "error out"=w276:errorcluster)  [unwired: 7 in, 3 out]
                  n142 = Unbundle By Name(w277) -> ("X"=w249:dbl, "Y"=w245:dbl)
                  n143 = Empty Array?(array=w270) -> (empty?=w271:bool)
                  n144 = Not(x=w271) -> (.not. x?=w235:bool)
                  n145 = Replace Array Subset(array=w261, new element=w260, index=w237) -> (w259:cluster{"Lower value":sgl, "Upper value":sgl}[])
                  n146 = Unbundle By Name(w268) -> ("Right"=w258:dbl, "Left"=w257:dbl, "Bottom"=w256:dbl, "Top"=w255:dbl)
                  n147 = Subtract(x=w258, y=w257) -> (x-y=w253:dbl)
                  n148 = Subtract(x=w256, y=w255) -> (x-y=w254:dbl)
                  n149 = Multiply(x=w253, y=w254) -> (x*y=w241:dbl)
                  n150 = Insert Into Array(array=w267, index=w240, new element=w245) -> (w243:dbl[])
                  n151 = Insert Into Array(array=w250, index=w240, new element=w249) -> (w247:dbl[])
                  n152 = Insert Into Array(array=w266, index=w240, new element=w241) -> (w239:dbl[])
                  n153 = for {
                    shift-right: [w278] -> w263
                    shift-left: dbl[] [] ("Array 4") -> [w281]
                    tunnel: w243 -> [w279] mode=indexing
                    n154 = Equal To 0?(x=w279) -> (x = 0?=w280:bool)
                    n155 = case shown="False" w280 {
                      tunnel: w281 -> [w284 w285]
                      tunnel: w279 -> [w283 _]
                      tunnel: [w282 w285] -> w278
                      frame False {
                        n156 = Build Array (concatenate)(w284, w283) -> (w282:dbl[])
                      }
                      frame True {
                      }
                    }
                  }
                  n157 = Replace Array Subset(array=w248, new element=w247, index (row)=w237) -> (w246:dbl[][])  [unwired: 1 in]
                  n158 = Replace Array Subset(array=w244, new element=w243, index (row)=w237) -> (w242:dbl[][])  [unwired: 1 in]
                  n159 = Replace Array Subset(array=w238, new element=w239, index (row)=w237) -> (w236:dbl[][])  [unwired: 1 in]
                  n160 = Array Size(array=w263) -> (size(s)=w252:i32)
                }
                "detected" <- w196
                "Box" <- w213
                n161 = Bundle(0, 1, "Centroid X"=w212) -> (→"Status":cluster{i32, i32, "Centroid X":dbl[][]})  [unwired: 1 in]
                n162 = Index Array(array=w205, index (row)=w214) -> (element=→"particles":T1)  [unwired: 1 in]
                n163 = call <vilib>:"Clear Errors.vi"("error in (no error)"=w204) -> ("error out"=w230:errorcluster)  [unwired: 6 in]
                n164 = local read "Numeric"() -> (w223:dbl)
                n165 = Increment(x=w190) -> (x+1=w220:i32)
                n166 = Greater Or Equal?(x=w223, y=w220) -> (x >= y?=w217:bool)
                n167 = Increment(x=w223) -> (x+1=w222:dbl)
                n168 = Select(t=0.0, s=w217, f=w222) -> (s? t:f=w221:dbl)
                n169 = local write "Numeric"(w221) -> ()
                n170 = Bundle By Name(cluster=w215, "thresholds"=w201) -> (w226:T37)
                n171 = for {
                  tunnel: w197 -> [w307] mode=indexing
                  tunnel: w210 -> [w313] mode=indexing
                  shift-right: [w308] -> w231
                  shift-left: "" ("GUIdevice 7") -> [w311]
                  tunnel: [w302] -> w233 mode=indexing
                  tunnel: "Detection Rate" -> [w306]
                  tunnel: w221 -> [w304]
                  tunnel: w190 -> [w300]
                  n172 = Greater Or Equal?(x=w307, y=w300) -> (x >= y?=w303:bool)
                  n173 = Multiply(x=w306, y=w304) -> (x*y=w305:dbl)
                  n174 = Greater Or Equal?(x=w307, y=w305) -> (x >= y?=w301:bool)
                  n175 = And(x=w303, y=w301) -> (x .and. y?=w302:bool)
                  n176 = Select(t=w313, s=w302, f="") -> (s? t:f=w309:string)
                  n177 = Concatenate Strings(w311, "\t", w309) -> (w308:string)
                }
                n178 = call <vilib>:"Add State(s) to Queue__jki_lib_state_machine.vi"("State(s) in (\"\")"=w192, "State(s) at Back (\"\")"="Device Ini" ("State(s) at Back (\"\")")) -> ("States Out"=w191:string)  [unwired: 13 in]
                n179 = Bundle By Name(cluster=w226, "Centroid X"=w200, "Centroid Y"=w199, "Size"=w198) -> (w195:T37)
                n180 = Unbundle By Name(w195) -> ("img to avg"=w194:i32)
                n181 = case shown="True" w217 {
                  tunnel: w195 -> [w286 w293]
                  tunnel: [w286 w292] -> w218
                  tunnel: w194 -> [_ w288]
                  frame False {
                  }
                  frame True {
                    n182 = Decrement(x=w288) -> (x-1=w291:i32)
                    n183 = Initialize Array(0.0 ("element"), 12 ("dimension size"), w291) -> (w287:dbl[][])
                    n184 = Bundle By Name(cluster=w293, "Centroid X"=w287, "Centroid Y"=w287, "Size"=w287) -> (w292:T37)
                  }
                }
                n185 = Or Array Elements(Boolean array=w233) -> (logical OR=w232:bool)
                n186 = case shown="True" w232 {
                  tunnel: w231 -> [_ w298]
                  tunnel: w191 -> [w294 w296]
                  tunnel: [w294 w295] -> w219
                  frame False {
                  }
                  frame True {
                    n187 = call <vilib>:"Build State String with Arguments__jki_lib_state_machine.vi"("Arguments (\"\")"=w298, "State"="detected") -> ("State with Arguments"=w297:string)  [unwired: 4 in]
                    n188 = call <vilib>:"Add State(s) to Queue__jki_lib_state_machine.vi"("State(s) in (\"\")"=w296, "State(s) at Back (\"\")"=w297) -> ("States Out"=w295:string)  [unwired: 13 in]
                  }
                }
              }
              event "Tab Control 2": Value Change {
                n189 = event-data() -> ()  [unwired: 1 in, 6 out]
                n190 = call <vilib>:"Add State(s) to Queue__jki_lib_state_machine.vi"("State(s) in Front (\"\")"=w316, "State(s) at Back (\"\")"="stats" ("State")) -> ("States Out"=w315:string)  [unwired: 13 in]
              }
              event "stop": Value Change {
                # "Exit Button Value Change (pressed) Event\n(this executes Macro: Exit to terminate the VI)"
                n191 = event-data() -> ()  [unwired: 1 in, 6 out]
                n192 = call <vilib>:"Add State(s) to Queue__jki_lib_state_machine.vi"("State(s) in Front (\"\")"="Macro: Exit", "State(s) in (\"\")"=w323) -> ("States Out"=w322:string)  [unwired: 13 in]
              }
              event Value Change {
                n193 = event-data() -> ()  [unwired: 1 in, 6 out]
                n194 = property on="Set Centriod Target" class="Bool (strict)"("Value"=FALSE) -> ()  [unwired: 2 in, 2 out]
                n195 = Unbundle By Name(w334) -> ("active ccd"=w326:i32, "Centroid X"=w325:dbl[][], "Centroid Y"=w324:dbl[][])
                n196 = Index Array(array=w330, index=w326) -> (element=w329:string)
                n197 = Concatenate Strings("Do want to update the target of " ("message"), w329, "?" ("string")) -> (w327:string)
                n198 = Two Button Dialog(message=w327) -> (T button?=w333:bool)  [unwired: 2 in]
                n199 = case shown="True" w333 {
                  tunnel: w332 -> [_ w345]
                  tunnel: w326 -> [_ w344]
                  tunnel: w325 -> [_ w351]
                  tunnel: w324 -> [_ w346]
                  frame False {
                  }
                  frame True {
                    n200 = Index Array(array=w351, index (row)=w344) -> (element=w350:dbl[])  [unwired: 1 in]
                    n201 = Index Array(array=w346, index (row)=w344) -> (element=w347:dbl[])  [unwired: 1 in]
                    n202 = Index Array(array=w345, index=w344) -> (element=w343:T31)
                    n203 = Unbundle By Name(w343) -> ("Target.X::12"=w342:refnum<vi>, "Target.Y::12"=w340:refnum<vi>)
                    n204 = Reverse 1D Array(array=w350) -> (reversed array=w349:dbl[])
                    n205 = Reverse 1D Array(array=w347) -> (reversed array=w348:dbl[])
                    n206 = Index Array(array=w349) -> (element=w341:dbl)  [unwired: 1 in]
                    n207 = Index Array(array=w348) -> (element=w339:dbl)  [unwired: 1 in]
                    n208 = property class="DigNum (strict)"(reference=w342, "Val(Sgnl)"=w341) -> ()  [unwired: 1 in, 2 out]
                    n209 = property class="DigNum (strict)"(reference=w340, "Val(Sgnl)"=w339) -> ()  [unwired: 1 in, 2 out]
                  }
                }
                n210 = call <vilib>:"Add State(s) to Queue__jki_lib_state_machine.vi"("State(s) in (\"\")"=w338) -> ("States Out"=w337:string)  [unwired: 14 in]
              }
              event "Feedback Global": Value Change {
                # "Exit Button Value Change (pressed) Event\n(this executes Macro: Exit to terminate the VI)"
                n211 = event-data() -> ("NewVal"=w354:bool)  [unwired: 1 in, 5 out]
                n212 = call <vilib>:"Add State(s) to Queue__jki_lib_state_machine.vi"("State(s) in (\"\")"=w357) -> ("States Out"=w356:string)  [unwired: 14 in]
                n213 = Bundle By Name(cluster=w353, "Feedback global"=w354) -> (w352:T37)
              }
              event Value Change {
                n214 = event-data() -> ()  [unwired: 1 in, 6 out]
                n215 = call <vilib>:"Add State(s) to Queue__jki_lib_state_machine.vi"("State(s) in Front (\"\")"="Move Config", "State(s) in (\"\")"=w362) -> ("States Out"=w361:string)  [unwired: 13 in]
              }
              event Value Change {
                n216 = event-data() -> ()  [unwired: 1 in, 6 out]
                n217 = call <vilib>:"Add State(s) to Queue__jki_lib_state_machine.vi"("State(s) in Front (\"\")"="Detection Config", "State(s) in (\"\")"=w367) -> ("States Out"=w366:string)  [unwired: 13 in]
              }
              event "associated motors": Value Change {
                n218 = event-data() -> ()  [unwired: 1 in, 6 out]
                n219 = call <vilib>:"Add State(s) to Queue__jki_lib_state_machine.vi"("State(s) in (\"\")"=w372, "State(s) at Back (\"\")"="Motor Config" ("State(s) at Back (\"\")")) -> ("States Out"=w371:string)  [unwired: 13 in]
              }
              event "Reset History": Value Change {
                n220 = event-data() -> ()  [unwired: 1 in, 6 out]
                n221 = call <vilib>:"Add State(s) to Queue__jki_lib_state_machine.vi"("State(s) in (\"\")"=w378, "State(s) at Back (\"\")"="Reset History" ("State(s) at Back (\"\")")) -> ("States Out"=w377:string)  [unwired: 13 in]
                n222 = property on="Reset History" class="Bool (strict)"("Value"=FALSE ("Reset History")) -> ()  [unwired: 2 in, 2 out]
              }
              event "Save Config": Value Change {
                n223 = event-data() -> ()  [unwired: 1 in, 6 out]
                n224 = call <vilib>:"Add State(s) to Queue__jki_lib_state_machine.vi"("State(s) in (\"\")"=w383, "State(s) at Back (\"\")"="Save Config" ("State(s) at Back (\"\")")) -> ("States Out"=w382:string)  [unwired: 13 in]
              }
              event "Load Config": Value Change {
                n225 = event-data() -> ()  [unwired: 1 in, 6 out]
                n226 = call "File Dialog2"("pattern (all files)"="*.cfg", "pattern label"="config") -> ("selected path"=w387:path)  [unwired: 10 in, 3 out]
                n227 = Path To String(path=w387) -> (string=w385:string)
                "config path" <- w385
                n228 = call <vilib>:"Build State String with Arguments__jki_lib_state_machine.vi"("Arguments (\"\")"=w385, "State"="Load Config" ("State(s) at Back (\"\")")) -> ("State with Arguments"=w384:string)  [unwired: 4 in]
                n229 = call <vilib>:"Add State(s) to Queue__jki_lib_state_machine.vi"("State(s) in (\"\")"=w393, "State(s) at Back (\"\")"=w384) -> ("States Out"=w392:string)  [unwired: 13 in]
              }
              event "Save Stats": Value Change {
                n230 = event-data() -> ()  [unwired: 1 in, 6 out]
                n231 = call <vilib>:"Add State(s) to Queue__jki_lib_state_machine.vi"("State(s) in (\"\")"=w398, "State(s) at Back (\"\")"="Save Stats" ("State(s) at Back (\"\")")) -> ("States Out"=w397:string)  [unwired: 13 in]
              }
              event "active CCDs": Value Change {
                n232 = event-data() -> ("NewVal"=w404:i32)  [unwired: 1 in, 5 out]
                n233 = Unbundle By Name(w400) -> ("active cams"=w399:string[])
                n234 = Index Array(array=w399, index=w404) -> (element=w402:string)
                n235 = call <vilib>:"Build State String with Arguments__jki_lib_state_machine.vi"("Arguments (\"\")"=w402, "State"="active" ("State(s) at Back (\"\")")) -> ("State with Arguments"=w401:string)  [unwired: 4 in]
                n236 = call <vilib>:"Add State(s) to Queue__jki_lib_state_machine.vi"("State(s) in (\"\")"=w407, "State(s) at Back (\"\")"=w401) -> ("States Out"=w406:string)  [unwired: 13 in]
              }
              event "Left", "Right": Value Change {
                n237 = event-data() -> ("CtlRef"=w416:refnum<vi>)  [unwired: 1 in, 5 out]
                n238 = property class="Bool (strict)"(reference=w416, error in=w413) -> (reference out=w415:refnum<vi>, error out=w414:errorcluster, "Label.Text"=w410:string)
                n239 = property class="Bool (strict)"(reference=w415, error in=w414, "Value"=FALSE) -> (error out=w412:errorcluster)  [unwired: 1 out]
                n240 = call <vilib>:"Build State String with Arguments__jki_lib_state_machine.vi"("Arguments (\"\")"=w410, "State"="ManMove X") -> ("State with Arguments"=w409:string)  [unwired: 4 in]
                n241 = call <vilib>:"Add State(s) to Queue__jki_lib_state_machine.vi"("State(s) in (\"\")"=w419, "State(s) at Back (\"\")"=w409) -> ("States Out"=w418:string)  [unwired: 13 in]
              }
              event "Up", "Down": Value Change {
                n242 = event-data() -> ("CtlRef"=w428:refnum<vi>)  [unwired: 1 in, 5 out]
                n243 = property class="Bool (strict)"(reference=w428, error in=w425) -> (reference out=w427:refnum<vi>, error out=w426:errorcluster, "Label.Text"=w422:string)
                n244 = property class="Bool (strict)"(reference=w427, error in=w426, "Value"=FALSE) -> (error out=w424:errorcluster)  [unwired: 1 out]
                n245 = call <vilib>:"Build State String with Arguments__jki_lib_state_machine.vi"("Arguments (\"\")"=w422, "State"="ManMove Y") -> ("State with Arguments"=w421:string)  [unwired: 4 in]
                n246 = call <vilib>:"Add State(s) to Queue__jki_lib_state_machine.vi"("State(s) in (\"\")"=w431, "State(s) at Back (\"\")"=w421) -> ("States Out"=w430:string)  [unwired: 13 in]
              }
              event "Center": Value Change {
                n247 = event-data() -> ()  [unwired: 1 in, 6 out]
                n248 = call <vilib>:"Add State(s) to Queue__jki_lib_state_machine.vi"("State(s) in (\"\")"=w436, "State(s) at Back (\"\")"="Center" ("State(s) at Back (\"\")")) -> ("States Out"=w435:string)  [unwired: 13 in]
              }
              event "new tdms": Value Change {
                n249 = event-data() -> ()  [unwired: 1 in, 6 out]
                n250 = call <vilib>:"Add State(s) to Queue__jki_lib_state_machine.vi"("State(s) in (\"\")"=w441, "State(s) at Back (\"\")"="newtdms" ("State(s) at Back (\"\")")) -> ("States Out"=w440:string)  [unwired: 13 in]
              }
              event "device ini": Value Change {
                n251 = event-data() -> ()  [unwired: 1 in, 6 out]
                n252 = property on="device ini" class="Bool (strict)"("Value"=FALSE ("test")) -> ()  [unwired: 2 in, 2 out]
                n253 = call <vilib>:"Add State(s) to Queue__jki_lib_state_machine.vi"("State(s) in (\"\")"=w447, "State(s) at Back (\"\")"="Device Ini" ("State(s) at Back (\"\")")) -> ("States Out"=w446:string)  [unwired: 13 in]
              }
              event "img to avg": Value Change {
                n254 = event-data() -> ("NewVal"=w453:i32)  [unwired: 1 in, 5 out]
                n255 = Number To Decimal String(number=w453) -> (decimal integer string=w455:string)  [unwired: 1 in]
                n256 = call <vilib>:"Build State String with Arguments__jki_lib_state_machine.vi"("Arguments (\"\")"=w455, "State"="ImgToAvg" ("State(s) at Back (\"\")")) -> ("State with Arguments"=w450:string)  [unwired: 4 in]
                n257 = call <vilib>:"Add State(s) to Queue__jki_lib_state_machine.vi"("State(s) in (\"\")"=w451, "State(s) at Back (\"\")"=w450) -> ("States Out"=w449:string)  [unwired: 13 in]
              }
              event Panel Close? {
                # "Discard the event because we'll close the front panel ourselves in Macro: Exit"
                # "Close Panel button (pressed) Event\n(this executes Macro: Exit to terminate the VI)"
                n258 = event-data() -> ()  [unwired: 1 in, 1 out]
                n259 = call <vilib>:"Add State(s) to Queue__jki_lib_state_machine.vi"("State(s) in Front (\"\")"="Macro: Exit", "State(s) in (\"\")"=w461) -> ("States Out"=w460:string)  [unwired: 13 in]
                n260 = event-data("Discard?"=TRUE) -> ()  [unwired: 1 in, 1 out]
              }
            }
          }
          frame "---------- Core ----------" {
            # "Do not put any code in this frame.\n(it is a separator no-op)"
            n261 = call <vilib>:"Add State(s) to Queue__jki_lib_state_machine.vi"("State(s) in (\"\")"=w465) -> ("States Out"=w464:string)  [unwired: 14 in]
          }
          frame Default {
            w475 = 42 items=["No error", "Argument error", "Memory is full", "Out of zone", "End of file", "File already open", "Generic file I/O error", "File not found", "File permission error", "Disk is full", "Duplicate path", "Too many files open", "System feature not enabled", "Resource file not found", "Cannot add resource", "Resource not found", "Image not found", "Image memory error", "Pen does not exist", "Config type invalid", "Config token not found", "Config parse error", "Config memory error", "Bad external code format", "Bad external code offset", "External code not present", "Null window", "Destroy window error", "Null menu", "Print aborted", "Bad print record", "Print driver error", "Windows error during printing", "Memory error during printing", "Print dialog error", "Generic print error", "Invalid device refnum", "Device not found", "Device parameter error", "Device unit error", "Cannot open device", "Device call aborted", "Generic error", "Cancelled by user", "Object ID too low", "Object ID too high", "Object not in heap", "Unknown heap", "Unknown object (invalid DefProc)", "Unknown object (DefProc not in table)", "Message out of range", "Invalid (null) method", "Unknown message", "Manager call not supported", "Bad address", "Network operation in progress", "Network operation timed out", "Connection is busy", "Network attribute not supported", "Network error", "Address in use", "System out of memory", "Connection aborted", "Connection refused", "Not connected", "Already connected", "Connection closed", "Initialization error (interapplication manager)", "Bad occurrence", "Wait on unbound occurrence handler", "Occurrence queue overflow", "Datalog type conflict", "Unused", "Unrecognized type (interapplication manager)", "Memory corrupt", "Failed to make temporary DLL", "Old CIN version", "Drag socket not found", "Failed to load drop-object", "Failed to register OLE object", "Failed to release OLE object", "Format specifier type mismatch", "Unknown format specifier", "Too few format specifiers", "Too many format specifiers", "Scan failed", "Newer CIN version", "Error converting to variant", "Runtime menu error", "Password tampered", "Variant attribute not found", "Incompatible variant data type", "Event data is not available", "Event Store is not present", "Occurrence is not found", "Event Queue is not created", "Event info is not available", "Refnum passed is NULL", "Error retrieving Class GUID", "Error retrieving CoClass GUID", "Error retrieving TypeLib GUID.", "Bad built application magic bytes.", "Specific driver is different from the specific driver associated with the Logical Name.", "There is no session opened to the class driver.", "Max Error", "MAX - Error with config objects", "MAX - Error loading configuration", "MAX - Group not supported"]
            # "Current State"
            # "Do not delete, rename, or modify this frame.\n(this is used to capture unhandled states and typos)"
            # "Handle mistyped state name (developer tool)"
            n262 = Format Into String(format string="Software Exception: Unhandled State \"%s\"." ("message"), error in=w471, w466) -> (resulting string=w474:string, error out=w473:errorcluster)  [unwired: 1 in]
            n263 = call <vilib>:"Error Cluster From Error Code.vi"("show call chain? (False)"=TRUE, "error in (no error)"=w473, "error message (\"\")"=w474, "error code (0)"=w475) -> ("error out"=w472:errorcluster)  [unwired: 5 in]
            n264 = call <vilib>:"Add State(s) to Queue__jki_lib_state_machine.vi"("State(s) in (\"\")"=w470) -> ("States Out"=w469:string)  [unwired: 14 in]
          }
          frame "Initialize Core Data" {
            # "Do not delete, rename, or modify this frame.\n(this is used to determine panel behavior on exit)"
            # "originally closed?"
            # "exe?"
            # "If panel starts closed or is an EXE, then close it when we exit"
            n265 = property class="VI"() -> ("Front Panel.Open"=w485:bool)  [unwired: 2 in, 2 out]
            n266 = property class="App"() -> ("App.Kind"=w484:T16)  [unwired: 2 in, 2 out]
            n267 = control-ref of="Current VI Reference"() -> (w479:refnum<vi>)
            n268 = Not(x=w485) -> (.not. x?=w482:bool)
            n269 = Equal?(x=w484, y=T16."Run Time System" ("Application:Kind")) -> (x = y?=w481:bool)
            n270 = Or(x=w482, y=w481) -> (x .or. y?=w480:bool)
            n271 = Bundle By Name(cluster=w478, "Core.Current VI Reference"=w479, "Core.Close Panel on Exit?"=w480) -> (w477:T37)
            n272 = call <vilib>:"Add State(s) to Queue__jki_lib_state_machine.vi"("State(s) in (\"\")"=w488) -> ("States Out"=w487:string)  [unwired: 14 in]
          }
          frame "Error Handler" {
            # "Unhandled Error -- Display it"
            # "Handle any errors here.\nYou can also output any states to clean-up after errors occur"
            # "Clear error"
            n273 = call <vilib>:"General Error Handler.vi"("error in (no error)"=w490) -> ()  [unwired: 10 in, 5 out]
            n274 = call <vilib>:"Add State(s) to Queue__jki_lib_state_machine.vi"("State(s) in Front (\"\")"="/* Post Error States", "State(s) in (\"\")"=w494) -> ("States Out"=w493:string)  [unwired: 13 in]
          }
          frame "Exit" {
            # "Do not put any code in this frame.\n(No errors that occur here will be handled.)"
            n275 = call <vilib>:"Add State(s) to Queue__jki_lib_state_machine.vi"("State(s) in (\"\")"=w499) -> ("States Out"=w498:string)  [unwired: 14 in]
          }
          frame "---------- Data ----------" {
            # "Do not put any code in this frame.\n(It is a separator no-op. You can make a copy of this frame to create a new Data frame)"
            n276 = call <vilib>:"Add State(s) to Queue__jki_lib_state_machine.vi"("State(s) in (\"\")"=w503) -> ("States Out"=w502:string)  [unwired: 14 in]
          }
          frame "Data: Initialize" {
            w504 = dbl[] [0.0, 0.0, 0.0, 0.0, 0.0, 0.0, 0.0, 0.0, 0.0, 0.0, 0.0, 0.0]  # steps speed Y
            w505 = dbl[] [0.0, 0.0, 0.0, 0.0, 0.0, 0.0, 0.0, 0.0, 0.0, 0.0, 0.0, 0.0]  # steps speed X
            w509 = bool[] [FALSE, FALSE, FALSE, FALSE, TRUE, TRUE, TRUE, FALSE, FALSE, FALSE, FALSE, FALSE]  # detected
            w519 = bool[] [FALSE, FALSE, FALSE, FALSE, FALSE, FALSE, FALSE, FALSE, FALSE, FALSE, FALSE, TRUE]  # speedmode Y
            w520 = bool[] [FALSE, FALSE, FALSE, FALSE, FALSE, FALSE, FALSE, FALSE, FALSE, FALSE, FALSE, TRUE]  # speedmode X
            w522 = cluster{"Lower value":sgl, "Upper value":sgl}[] [{"Lower value"=93.0, "Upper value"=255.0}, {"Lower value"=105.0, "Upper value"=255.0}, {"Lower value"=0.0, "Upper value"=255.0}, {"Lower value"=127.0, "Upper value"=255.0}, {"Lower value"=0.0, "Upper value"=255.0}, {"Lower value"=0.0, "Upper value"=255.0}, {"Lower value"=0.0, "Upper value"=255.0}, {"Lower value"=0.0, "Upper value"=255.0}, {"Lower value"=0.0, "Upper value"=255.0}, {"Lower value"=0.0, "Upper value"=255.0}, {"Lower value"=0.0, "Upper value"=255.0}, {"Lower value"=0.0, "Upper value"=255.0}]  # thresholds
            w529 = FALSE  # Feedback global
            w531 = 0  # active ccd
            w515 = 6  # img to avg
            w542 = T38 {"Current VI Reference"=refnum, "Close Panel on Exit?"=FALSE}  # Core
            # "Initialize the shift-register data, here.\n(data names are defined by what you wire into the bundle function)"
            n277 = disable-structure shown="Disabled" {
              disable-tunnel: w512 -> [w554 _]
              disable-tunnel: [w553 _] -> w511
              disable-tunnel: w510 -> [w552 _]
              disable-tunnel: [w551 _] -> _
              disable-tunnel: w508 -> [w545 _]
              frame Disabled {
                n278 = TDMS Open(6:FALSE ("disable buffering (T)"), 7:enum16{"1.0", "2.0"}."2.0" ("file format version (2.0)"), 8:w554, 10:T17."create or replace" ("operation"), 11:w552) -> (0:w549:errorcluster, 3:w550:refnum<k34>)  [unwired: 2 in]
                n279 = call "TDMSbuffersize.vi"("error in (no error)"=w549, "group names"=w545, "Data Value Reference in"=w550) -> ("error out"=w553:errorcluster, "Data Value Reference out"=w551:refnum<k34>)  [unwired: 7 in]
              }
              frame Enabled {
              }
            }
            n280 = call <vilib>:"Add State(s) to Queue__jki_lib_state_machine.vi"("State(s) in Front (\"\")"="newtdms" ("State(s) in Front (\"\")"), "State(s) in (\"\")"=w544) -> ("States Out"=w543:string)  [unwired: 13 in]
            n281 = Bundle("Core"=w542, "detection para"="detection para", "thresholds"=w522, "Centroid X"="Centroid X", "Centroid Y"="Centroid Y", "img to avg"=w515, "Mean Centroid X"="Mean Centroid X", "Mean Centroid Y"="Mean Centroid Y", "Offset X"="Offset X", "Offset Y"="Offset Y", "Offset X stats"="Offset X stats", "Offset Y stats"="Offset Y stats", "Size"="Size", "Mean Size"="Mean Size", "Time"="Time", "move properties"="move properties", "active axis refs 2"="active axis refs 2", "active ccd"=w531, "Feedback global"=w529, "Motor X"="Motor X", "Motor Y"="Motor Y", "active cams"="active cams", "Data Value Reference out"=refnum<k34> refnum, "active man refs"="active man refs", "detected"=w509, "speedmode X"=w520, "speedmode Y"=w519, "steps speed X"=w505, "steps speed Y"=w504) -> (w514:T37)  [unwired: 1 in]
            n282 = Initialize Array(0.0 ("element"), 12 ("dimension size"), w515) -> (w518:dbl[][])
            n283 = Bundle By Name(cluster=w514, "Centroid X"=w518, "Centroid Y"=w518, "Size"=w518) -> (w513:T37)
          }
          frame "Data: Cleanup" {
            # "Cleanup any data and references, here.\n(this is called automatically, by the Macro: Exit)"
            n284 = Unbundle By Name(w555) -> ("Core.Current VI Reference"=w556:refnum<vi>)
            n285 = Close Reference(reference=w556, error in (no error)=w558) -> (error out=w557:errorcluster)
            n286 = call <vilib>:"Add State(s) to Queue__jki_lib_state_machine.vi"("State(s) in (\"\")"=w560) -> ("States Out"=w559:string)  [unwired: 14 in]
          }
          frame "---------- UI ----------" {
            # "Do not put any code in this frame.\n(It is a separator no-op. You can make a copy of this frame to create a new UI frame)"
            n287 = call <vilib>:"Add State(s) to Queue__jki_lib_state_machine.vi"("State(s) in (\"\")"=w564) -> ("States Out"=w563:string)  [unwired: 14 in]
          }
          frame "UI: Initialize" {
            # "Initialize the User Interface, here.\n(this is called automatically, by the Macro: Init)"
            n288 = call <vilib>:"Add State(s) to Queue__jki_lib_state_machine.vi"("State(s) in (\"\")"=w568) -> ("States Out"=w567:string)  [unwired: 14 in]
          }
          frame "UI: Cursor Set" {
            # "Argument"
            # "Set and Unset Cursor Busy.\n(Usage: \"UI: Cursor Set >> Busy|Idle\")"
            n289 = case shown="\"Idle\", Default" w569 {
              tunnel: w571 -> [w576 w578]
              tunnel: [w575 w577] -> w570
              frame "Idle", Default {
                n290 = call <vilib>:"Unset Busy.vi"("error in (no error)"=w576) -> ("error out"=w575:errorcluster)  [unwired: 10 in]
              }
              frame "Busy" {
                n291 = call <vilib>:"Set Busy.vi"("error in (no error)"=w578) -> ("error out"=w577:errorcluster)  [unwired: 9 in, 1 out]
              }
            }
            n292 = call <vilib>:"Add State(s) to Queue__jki_lib_state_machine.vi"("State(s) in (\"\")"=w574) -> ("States Out"=w573:string)  [unwired: 14 in]
          }
          frame "UI: Front Panel State" {
            # "Argument"
            # "Set Front Panel Open or Closed\n(Usage: \"UI: Front Panel State >> Open|Close\")"
            n293 = Unbundle By Name(w579) -> ("Core.Current VI Reference"=w581:refnum<vi>)
            n294 = case shown="\"Open\", Default" w580 {
              tunnel: w583 -> [w589 w600]
              tunnel: [w590 w601] -> w582
              tunnel: w581 -> [_ _]
              frame "Open", Default {
                n295 = property class="VI"(error in=w589) -> (reference out=w587:refnum<vi>, error out=w588:errorcluster, "Front Panel.Open"=w586:bool)  [unwired: 1 in]
                n296 = case shown="False" w586 {
                  tunnel: [w593 w596] -> w590
                  tunnel: w588 -> [w592 w596]
                  tunnel: w587 -> [w591 _]
                  frame False {
                    n297 = invoke class="VI" method="FP.Open"(reference=w591, error in=w592, "Activate"=TRUE, "State"=T18."Standard") -> (error out=w593:errorcluster)  [unwired: 1 in, 4 out]
                  }
                  frame True {
                  }
                }
              }
              frame "Close" {
                n298 = property class="VI"(error in=w600) -> (reference out=w598:refnum<vi>, error out=w599:errorcluster, "Front Panel.Open"=w597:bool)  [unwired: 1 in]
                n299 = case shown="True" w597 {
                  tunnel: [w602 w605] -> w601
                  tunnel: w599 -> [w602 w604]
                  tunnel: w598 -> [_ w603]
                  frame False {
                  }
                  frame True {
                    n300 = invoke class="VI" method="FP.Close"(reference=w603, error in=w604) -> (error out=w605:errorcluster)  [unwired: 1 in, 2 out]
                  }
                }
              }
            }
            n301 = call <vilib>:"Add State(s) to Queue__jki_lib_state_machine.vi"("State(s) in (\"\")"=w585) -> ("States Out"=w584:string)  [unwired: 14 in]
          }
          frame "---------- Macro ----------" {
            # "Do not put any code in this frame.\n(It is a separator no-op. You can make a copy of this frame to create a new Macro frame)"
            n302 = call <vilib>:"Add State(s) to Queue__jki_lib_state_machine.vi"("State(s) in (\"\")"=w609) -> ("States Out"=w608:string)  [unwired: 14 in]
          }
          frame "Macro: Initialize" {
            # "Initialization Macro\n(This is called once, when the VI starts)"
            n303 = property on="img to avg" class="DigNum (strict)"() -> ("Value"=w611:i32)  [unwired: 2 in, 2 out]
            n304 = Number To Decimal String(number=w611) -> (decimal integer string=w613:string)  [unwired: 1 in]
            n305 = call <vilib>:"Build State String with Arguments__jki_lib_state_machine.vi"("Arguments (\"\")"=w613, "State"="ImgToAvg") -> ("State with Arguments"=w610:string)  [unwired: 4 in]
            n306 = call <vilib>:"Add State(s) to Queue__jki_lib_state_machine.vi"("State(s) in Front (\"\")"="Data: Initialize\nInitialize Core Data\nUI: Initialize\nUI: Front Panel State >> Open\nDevice Ini >> 3000", "State(s) in (\"\")"=w618, "State(s) at Back (\"\")"=w610) -> ("States Out"=w617:string)  [unwired: 12 in]
          }
          frame "Macro: Exit" {
            # "Exit Macro\n(This is called once, when the VI exits)"
            n307 = Unbundle By Name(w620) -> ("Core.Close Panel on Exit?"=w619:bool)
            n308 = Select(t="UI: Front Panel State >> Close", s=w619, f="") -> (s? t:f=w623:string)
            n309 = call <vilib>:"Add State(s) to Queue__jki_lib_state_machine.vi"("State(s) in (\"\")"=w623, "State(s) at Back (\"\")"="Data: Cleanup\nExit") -> ("States Out"=w621:string)  [unwired: 13 in]
            n310 = call <vilib>:"Add State(s) to Queue__jki_lib_state_machine.vi"("State(s) in Front (\"\")"=w621, "State(s) in (\"\")"=w628) -> ("States Out"=w627:string)  [unwired: 13 in]
          }
          frame "---------- Ini and Configure ----------" {
            # "Template Separator\n(You can make a copy of, or modify, this frame)"
            n311 = call <vilib>:"Add State(s) to Queue__jki_lib_state_machine.vi"("State(s) in (\"\")"=w632) -> ("States Out"=w631:string)  [unwired: 14 in]
          }
          frame "Device Ini" {
            # "Your code here.\n(You can make a copy of, or modify, this frame)"
            n312 = Empty String/Path?(string/path=w638) -> (empty?=w655:bool)
            n313 = flat-sequence {
              tunnel: w641 -> [w662]
              tunnel: [w662] -> w642
              tunnel: w640 -> [w661]
              tunnel: w642 -> [w667]
              tunnel: [w665] -> w639
              frame #0 {
                n314 = Wait (ms)(milliseconds to wait=w661) -> ()  [unwired: 1 out]
              }
              frame #1 {
                n315 = local read "Array 3"() -> (w663:sgl[])
                n316 = disable-structure shown="Disabled" {
                  disable-tunnel: w667 -> [w670 _]
                  disable-tunnel: [w668 _] -> _
                  frame Disabled {
                    n317 = for {
                      tunnel: w670 -> [w671] mode=indexing
                      shift-right: [w673] -> w668
                      shift-left: string[] [] -> [w674]
                      n318 = call "send command.vi"("Device Name"=w671) -> ("status"=w675:bool)  [unwired: 4 in]
                      n319 = Wait (ms)(milliseconds to wait=u32 1) -> ()  [unwired: 1 out]
                      n320 = case shown="True" w675 {
                        tunnel: w674 -> [w676 w679]
                        tunnel: [w676 w678] -> w673
                        tunnel: w671 -> [_ w677]
                        frame False {
                        }
                        frame True {
                          n321 = Build Array (concatenate)(w679, w677) -> (w678:string[])
                        }
                      }
                    }
                  }
                  frame Enabled {
                  }
                }
                n322 = for {
                  tunnel: w667 -> [w682] mode=indexing
                  shift-right: [w687] -> w665
                  shift-left: string[] [] -> [w688]
                  tunnel: [w681] -> w664 mode=indexing
                  shift-right: [w685] -> _
                  shift-left: w663 -> [w685]
                  i -> [w686]
                  n323 = call "IMAQ Histograph"("Image"=w682) -> ("error out"=w680:errorcluster, "Mean Value"=w681:sgl)  [unwired: 7 in, 2 out]
                  n324 = Index Array(array=w685, index=w686) -> (element=w684:sgl)
                  n325 = call <vilib>:"Clear Errors.vi"("error in (no error)"=w680) -> ()  [unwired: 6 in, 1 out]
                  n326 = Equal?(x=w681, y=w684) -> (x = y?=w683:bool)
                  n327 = case shown="False" w683 {
                    tunnel: w688 -> [w691 w692]
                    tunnel: [w690 w692] -> w687
                    tunnel: w682 -> [w689 _]
                    frame False {
                      n328 = Build Array (concatenate)(w691, w689) -> (w690:string[])
                    }
                    frame True {
                    }
                  }
                }
                "Array 3" <- w664
              }
            }
            n329 = case shown="False" w655 {
              tunnel: w638 -> [w727 _]
              tunnel: [w726 0] -> w640
              frame False {
                n330 = Decimal String To Number(string=w727) -> (number=w726:i32)  [unwired: 2 in, 1 out]
              }
              frame True {
              }
            }
            n331 = Equal?(x=w638, y="T") -> (x = y?=w635:bool)
            n332 = Unbundle By Name(w654) -> ("active cams"=w647:string[])
            n333 = call <vilib>:"Add State(s) to Queue__jki_lib_state_machine.vi"("State(s) in (\"\")"=w660) -> ("States Out"=w649:string)  [unwired: 14 in]
            n334 = Equal?(x=w647, y=w639) -> (x = y?=w653:bool[])
            n335 = Empty Array?(array=w647) -> (empty?=w652:bool)
            n336 = Not(x=w652) -> (.not. x?=w651:bool)
            n337 = Build Array (concatenate)(w653, w651) -> (w650:bool[])
            n338 = Array Size(array=w639) -> (size(s)=w646:i32)
            n339 = Array Size(array=w647) -> (size(s)=w645:i32)
            n340 = And Array Elements(Boolean array=w650) -> (logical AND=w643:bool)
            n341 = Equal?(x=w646, y=w645) -> (x = y?=w644:bool)
            n342 = And(x=w644, y=w643) -> (x .and. y?=w636:bool)
            n343 = Not(x=w636) -> (.not. x?=w634:bool)
            n344 = Or(x=w635, y=w634) -> (x .or. y?=w633:bool)
            n345 = case shown="True" w633 {
              tunnel: [w695 w711] -> w659
              tunnel: w658 -> [_ _]
              tunnel: w657 -> [w694 w709]
              tunnel: [w694 w709] -> w656
              tunnel: w654 -> [w695 w705]
              tunnel: w639 -> [_ w706]
              tunnel: w649 -> [w693 _]
              tunnel: [w693 w699] -> w648
              frame False {
              }
              frame True {
                n346 = property on="active CCDs" class="LstBox (strict)"("Item Names"=w706) -> ()  [unwired: 2 in, 2 out]
                n347 = Array Size(array=w706) -> (size(s)=w718:i32)
                n348 = Initialize Array(0.0 ("element"), w718, 0 ("dimension size")) -> (w713:dbl[][])
                n349 = Unbundle By Name(w705) -> ("img to avg"=w704:i32)
                n350 = Bundle By Name(cluster=w705, "active cams"=w706) -> (w712:T37)
                n351 = Initialize Array(0.0 ("element"), 12 ("dimension size"), w704) -> (w703:dbl[][])
                n352 = local write "Numeric"(0.0 ("Numeric")) -> ()
                n353 = Bundle By Name(cluster=w712, "Offset X stats"=w713, "Offset Y stats"=w713, "Centroid X"=w703, "Centroid Y"=w703, "Mean Centroid X"=w713, "Mean Centroid Y"=w713, "Offset X"=w713, "Offset Y"=w713, "Size"=w703, "Mean Size"=w713, "Motor X"=w713, "Motor Y"=w713) -> (w711:T37)
                n354 = for {
                  N: 1 -> [_]
                  shift-right: [w720] -> w716
                  shift-left: timestamp[][] [] ("Time") -> [w722]
                  n355 = for {
                    N: 12 -> [_]
                    tunnel: w722 -> [w725] mode=indexing
                    tunnel: [w723] -> w720 mode=indexing
                    n356 = Get Date/Time In Seconds() -> (seconds since 1Jan1904=w724:timestamp)
                    n357 = Build Array (concatenate)(w725, w724) -> (w723:timestamp[])
                  }
                }
                n358 = property on="config path" class="Str"() -> ("Value"=w701:string)  [unwired: 2 in, 2 out]
                n359 = call <vilib>:"Add State(s) to Queue__jki_lib_state_machine.vi"("State(s) in Front (\"\")"="Move Config\nMotor Config\nDetection Config\nactive\nCenter" ("State(s) in Front (\"\")"), "State(s) in (\"\")"="" ("State(s) in (\"\")")) -> ("States Out"=w700:string)  [unwired: 13 in]
                n360 = call <vilib>:"Build State String with Arguments__jki_lib_state_machine.vi"("Arguments (\"\")"=w701, "State"="Load Config" ("State(s) in Front (\"\")")) -> ("State with Arguments"=w698:string)  [unwired: 4 in]
                n361 = call <vilib>:"Add State(s) to Queue__jki_lib_state_machine.vi"("State(s) in (\"\")"=w700, "State(s) at Back (\"\")"=w698) -> ("States Out"=w699:string)  [unwired: 13 in]
                n362 = property on="Time" class="Arr (strict)"("Value"=w716) -> ()  [unwired: 2 in, 2 out]
                "name array" <- w706
              }
            }
          }
          frame "Load Config" {
            # "Your code here.\n(You can make a copy of, or modify, this frame)"
            n363 = Unbundle By Name(w770) -> ("detection para"=w776:T3[], "move properties"=w773:T2[], "thresholds"=w766:cluster{"Lower value":sgl, "Upper value":sgl}[])
            n364 = Empty String/Path?(string/path=w733) -> (empty?=w732:bool)
            n365 = case shown="False" w732 {
              tunnel: [w786 T5 {"CCDs"=[], "move properties"=[], "detection para"=[], "thresholds"=[], "Value"={"Motor CCD 1"=0, "Motor CCD 2"=0, "Motor CCD 3"=0, "Motor CCD 4"=0, "Motor CCD 5"=0, "Motor CCD 6"=0, "Motor CCD 7"=0, "Motor CCD 8"=0, "Motor CCD 9"=0, "Motor CCD 10"=0, "Motor CCD 11"=0, "Motor CCD 12"=0}} ("output cluster 2")] -> w778
              tunnel: [w784 w793] -> w737
              tunnel: w734 -> [w783 w793]
              tunnel: w733 -> [w782 _]
              frame False {
                n366 = String To Path(string=w782) -> (path=w781:path)
                n367 = Open/Create/Replace File(file path (use dialog)=w781, error in=w783, operation (0:open)=T19."open or create") -> (refnum out=w788:refnum<file>, error out=w789:errorcluster)  [unwired: 3 in, 1 out]
                n368 = Read from Binary File(5:"output cluster 2", 8:w789, 11:w788) -> (0:w790:errorcluster, 2:w786:T5, 3:w791:refnum<file>)  [unwired: 3 in, 1 out]
                n369 = Close File(refnum=w791, error in=w790) -> (error out=w784:errorcluster)  [unwired: 1 out]
              }
              frame True {
              }
            }
            n370 = property on="Load Config" class="Bool (strict)"("Value"=FALSE ("Load Config")) -> ()  [unwired: 2 in, 2 out]
            n371 = Unbundle By Name(w778) -> ("Value"=w764:T7, "CCDs"=w777:string[], "detection para"=w775:T3[], "move properties"=w774:T2[], "thresholds"=w767:cluster{"Lower value":sgl, "Upper value":sgl}[])
            n372 = Cluster To Array(cluster=w764) -> (array=w765:u16[])
            n373 = call <vilib>:"Add State(s) to Queue__jki_lib_state_machine.vi"("State(s) in (\"\")"=w780, "State(s) at Back (\"\")"="Motor Config" ("State(s) at Back (\"\")")) -> ("States Out"=w779:string)  [unwired: 13 in]
            n374 = for {
              tunnel: w777 -> [w809]
              tunnel: w775 -> [w811]
              tunnel: w774 -> [w810]
              shift-right: [w803] -> w772
              shift-left: w776 -> [w808]
              shift-right: [w801] -> w771
              shift-left: w773 -> [w807]
              tunnel: w768 -> [w806] mode=indexing
              tunnel: w767 -> [w802]
              shift-right: [w798] -> w730
              shift-left: w766 -> [w800]
              tunnel: w765 -> [w797]
              tunnel: [w794] -> w763 mode=indexing
              i -> [w795]
              n375 = call-poly <userlib>:"Filter 1D Array__ogtk.vi"("items to filter"=w806, "array"=w809) -> ("filtered item indices"=w812:i32[])  [unwired: 4 in, 1 out]
              n376 = Index Array(array=w812) -> (element=w796:i32)  [unwired: 1 in]
              n377 = Index Array(array=w797, index=w796) -> (element=w794:u16)
              n378 = Index Array(array=w811, index=w796) -> (element=w805:T3)
              n379 = Index Array(array=w810, index=w796) -> (element=w804:T2)
              n380 = Index Array(array=w802, index=w796) -> (element=w799:cluster{"Lower value":sgl, "Upper value":sgl})
              n381 = Replace Array Subset(array=w808, new element=w805, index=w795) -> (w803:T3[])
              n382 = Replace Array Subset(array=w807, new element=w804, index=w795) -> (w801:T2[])
              n383 = Replace Array Subset(array=w800, new element=w799, index=w795) -> (w798:cluster{"Lower value":sgl, "Upper value":sgl}[])
            }
            n384 = Array Size(array=w730) -> (size(s)=→"size(s) 6":i32)
            n385 = Index Array(array=w763, index #1=0 ("index (row)"), index #2=1 ("index (row)"), index #3=2 ("index (row)"), index #4=3 ("index (row)"), index #5=4 ("index (row)"), index #6=5 ("index (row)"), index #7=6 ("index (row)"), index #8=7 ("index (row)"), index #9=8 ("index (row)"), index #10=9 ("index (row)"), index #11=10 ("index (row)"), index #12=11 ("index (row)")) -> (element #1=w750:u16, element #2=w749:u16, element #3=w748:u16, element #4=w747:u16, element #5=w746:u16, element #6=w745:u16, element #7=w744:u16, element #8=w743:u16, element #9=w742:u16, element #10=w741:u16, element #11=w740:u16, element #12=w739:u16)
            n386 = Bundle By Name(cluster=w764, "Motor CCD 1"=w750, "Motor CCD 2"=w749, "Motor CCD 3"=w748, "Motor CCD 4"=w747, "Motor CCD 5"=w746, "Motor CCD 6"=w745, "Motor CCD 7"=w744, "Motor CCD 8"=w743, "Motor CCD 9"=w742, "Motor CCD 10"=w741, "Motor CCD 11"=w740, "Motor CCD 12"=w739) -> (w738:T7)
            n387 = Bundle By Name(cluster=w770, "detection para"=w772, "move properties"=w771, "thresholds"=w730) -> (w769:T37)
            n388 = property on="associated motors" class="Clust (strict)"(error in=w737, "Val(Sgnl)"=w738) -> (error out=w736:errorcluster)  [unwired: 1 in, 1 out]
          }
          frame "Save Config" {
            # "Your code here.\n(You can make a copy of, or modify, this frame)"
            n389 = Unbundle By Name(w830) -> ("move properties"=w816:T2[], "detection para"=w825:T3[], "thresholds"=w813:cluster{"Lower value":sgl, "Upper value":sgl}[])
            n390 = property on="associated motors" class="Clust (strict)"() -> ("Value"=w824:T7)  [unwired: 2 in, 2 out]
            n391 = property on="Save Config" class="Bool (strict)"("Value"=FALSE ("Save Config")) -> ()  [unwired: 2 in, 2 out]
            n392 = local read "CCDs"() -> (w814:string[])
            n393 = call "File Dialog"("pattern (all files)"="*.cfg", "pattern label"="config") -> ("selected path"=w818:path)  [unwired: 10 in, 3 out]
            n394 = Bundle("CCDs"=w814, "move properties"=w816, "detection para"=w825, "thresholds"=w813, "Value"=w824) -> (w817:T5)  [unwired: 1 in]
            n395 = Open/Create/Replace File(file path (use dialog)=w818, error in=w822, operation (0:open)=T19."replace or create with confirmation") -> (refnum out=w826:refnum<file>, error out=w827:errorcluster)  [unwired: 3 in, 1 out]
            n396 = Write to Binary File(file (use dialog)=w826, data=w817, error in=w827) -> (refnum out=w829:refnum<file>, error out=w828:errorcluster)  [unwired: 3 in, 1 out]
            n397 = Close File(refnum=w829, error in=w828) -> (error out=w821:errorcluster)  [unwired: 1 out]
            n398 = call <vilib>:"Add State(s) to Queue__jki_lib_state_machine.vi"("State(s) in (\"\")"=w832) -> ("States Out"=w831:string)  [unwired: 14 in]
          }
          frame "active" {
            # "Your code here.\n(You can make a copy of, or modify, this frame)"
            n399 = Empty String/Path?(string/path=w847) -> (empty?=w846:bool)
            n400 = Unbundle By Name(w843) -> ("move properties"=w859:T2[], "detection para"=w855:T3[])  [unwired: 1 out]
            n401 = Unbundle By Name(w843) -> ("active axis refs 2"=w842:T11)
            n402 = call-poly <userlib>:"Filter 1D Array__ogtk.vi"("items to filter"=w847, "array"=w857) -> ("filtered item indices"=w860:i32[])  [unwired: 4 in, 1 out]
            n403 = Index Array(array=w860) -> (element=w844:i32)  [unwired: 1 in]
            n404 = Select(t=0, s=w846, f=w844) -> (s? t:f=w840:i32)
            n405 = Index Array(array=w842, index=w840) -> (element=w841:cluster{"Ref X":refnum<vi>, "Ref Y":refnum<vi>})
            n406 = Unbundle By Name(w841) -> ("Ref X"=w839:refnum<vi>, "Ref Y"=w838:refnum<vi>)
            n407 = Index Array(array=w859, index=w840) -> (element=w858:T2)
            n408 = Index Array(array=w855, index=w840) -> (element=w854:T3)
            n409 = property on="move config" class="Clust (strict)"(error in=w850, "Value"=w858) -> (error out=w848:errorcluster)  [unwired: 1 in, 1 out]
            n410 = property on="beam detection para" class="Clust (strict)"(error in=w848, "Value"=w854) -> (error out=w849:errorcluster)  [unwired: 1 in, 1 out]
            n411 = call <vilib>:"Add State(s) to Queue__jki_lib_state_machine.vi"("State(s) in (\"\")"=w862) -> ("States Out"=w861:string)  [unwired: 14 in]
            n412 = property class="DigNum (strict)"(reference=w839, error in=w849) -> (error out=w835:errorcluster, "Value"=w837:dbl)  [unwired: 1 out]
            n413 = Bundle By Name(cluster="active Axis ref 3", "Ref X"=w839, "Ref Y"=w838) -> (w852:cluster{"Ref X":refnum<vi>, "Ref Y":refnum<vi>})
            n414 = Bundle By Name(cluster=w843, "active ccd"=w840, "active man refs"=w852) -> (w856:T37)
            n415 = property on="Position 1" class="DigNum (strict)"(error in=w835, "Value"=w837) -> (error out=w834:errorcluster)  [unwired: 1 in, 1 out]
            n416 = property class="DigNum (strict)"(reference=w838, error in=w834) -> (error out=w833:errorcluster, "Value"=w836:dbl)  [unwired: 1 out]
            n417 = property on="Position 2" class="DigNum (strict)"(error in=w833, "Value"=w836) -> (error out=w851:errorcluster)  [unwired: 1 in, 1 out]
          }
          frame "Detection Config" {
            # "Your code here.\n(You can make a copy of, or modify, this frame)"
            n418 = Unbundle By Name(w867) -> ("detection para"=w863:T3[], "active ccd"=w868:i32)
            n419 = Replace Array Subset(array=w863, new element="beam detection para", index=w868) -> (w864:T3[])
            n420 = Bundle By Name(cluster=w867, "detection para"=w864) -> (w866:T37)
            n421 = call <vilib>:"Add State(s) to Queue__jki_lib_state_machine.vi"("State(s) in (\"\")"=w871) -> ("States Out"=w870:string)  [unwired: 14 in]
          }
          frame "Motor Config" {
            # "Your code here.\n(You can make a copy of, or modify, this frame)"
            n422 = Unbundle By Name("associated motors") -> ("Motor CCD 1"=w888:u16, "Motor CCD 2"=w889:u16, "Motor CCD 3"=w890:u16, "Motor CCD 4"=w883:u16, "Motor CCD 5"=w882:u16, "Motor CCD 6"=w881:u16, "Motor CCD 7"=w880:u16, "Motor CCD 8"=w879:u16, "Motor CCD 9"=w878:u16, "Motor CCD 10"=w877:u16, "Motor CCD 11"=w876:u16, "Motor CCD 12"=w875:u16)
            n423 = Build Array(w888, w889, w890, w883, w882, w881, w880, w879, w878, w877, w876, w875) -> (w874:u16[])
            n424 = local read "motor refs"() -> (w886:refnum<vi>[])
            n425 = Increment(x=w874) -> (x+1=w873:u16[])
            n426 = for {
              tunnel: w873 -> [w905] mode=indexing
              tunnel: w886 -> [w900]
              tunnel: [w894] -> w872 mode=indexing
              n427 = Multiply(x=w905, y=u16 2) -> (x*y=w901:u16)
              n428 = Subtract(x=w901, y=u16 2) -> (x-y=w899:u16)
              n429 = Subtract(x=w901, y=u16 1) -> (x-y=w898:u16)
              n430 = Index Array(array=w900, index=w899) -> (element=w897:refnum<vi>)
              n431 = Index Array(array=w900, index=w898) -> (element=w896:refnum<vi>)
              n432 = Bundle By Name(cluster="active Axis ref", "Ref X"=w897, "Ref Y"=w896) -> (w894:cluster{"Ref X":refnum<vi>, "Ref Y":refnum<vi>})
            }
            n433 = call <vilib>:"Add State(s) to Queue__jki_lib_state_machine.vi"("State(s) in (\"\")"=w893) -> ("States Out"=w892:string)  [unwired: 14 in]
            n434 = Bundle By Name(cluster=w885, "active axis refs 2"=w872) -> (w884:T37)
          }
          frame "Move Config" {
            # "Your code here.\n(You can make a copy of, or modify, this frame)"
            n435 = Unbundle By Name(w907) -> ("move properties"=w911:T2[], "active ccd"=w910:i32)
            n436 = Replace Array Subset(array=w911, new element="move config", index=w910) -> (w908:T2[])
            n437 = Bundle By Name(cluster=w907, "move properties"=w908) -> (w906:T37)
            n438 = call <vilib>:"Add State(s) to Queue__jki_lib_state_machine.vi"("State(s) in (\"\")"=w914) -> ("States Out"=w913:string)  [unwired: 14 in]
          }
          frame "----------Centroid & Move----------" {
            # "Template Separator\n(You can make a copy of, or modify, this frame)"
            n439 = call <vilib>:"Add State(s) to Queue__jki_lib_state_machine.vi"("State(s) in (\"\")"=w918) -> ("States Out"=w917:string)  [unwired: 14 in]
          }
          frame "detected" {
            n440 = Unbundle By Name(w923) -> ("Offset X"=w958:dbl[][], "Offset Y"=w957:dbl[][], "Size"=w956:dbl[][], "Mean Size"=w955:dbl[][], "Time"=w952:timestamp[][], "Motor X"=w932:dbl[][], "active axis refs 2"=w931:T11, "Motor Y"=w930:dbl[][])
            n441 = Spreadsheet String To Array(format string="%s", spreadsheet string=w935, array type (2D Dbl)=string[] []) -> (array=w926:string[])  [unwired: 1 in]
            n442 = for {
              tunnel: w927 -> [w972] mode=indexing
              tunnel: w926 -> [w971]
              tunnel: [w970] -> w925 mode=indexing
              n443 = for {
                tunnel: w972 -> [w975]
                tunnel: [w974] -> w969 mode=indexing
                tunnel: w971 -> [w973] mode=indexing
                n444 = Equal?(x=w975, y=w973) -> (x = y?=w974:bool)
              }
              n445 = Or Array Elements(Boolean array=w969) -> (logical OR=w970:bool)
            }
            n446 = Unbundle By Name(w923) -> ("Mean Centroid X"=w963:dbl[][], "Mean Centroid Y"=w962:dbl[][], "Centroid X"=w965:dbl[][], "Centroid Y"=w964:dbl[][])
            n447 = call <vilib>:"Build State String with Arguments__jki_lib_state_machine.vi"("Arguments (\"\")"=w935, "State"="stats") -> ("State with Arguments"=w936:string)  [unwired: 4 in]
            n448 = call <vilib>:"Add State(s) to Queue__jki_lib_state_machine.vi"("State(s) in Front (\"\")"=w936, "State(s) in (\"\")"=w934) -> ("States Out"=w933:string)  [unwired: 13 in]
            n449 = for {
              tunnel: w965 -> [w1025]
              tunnel: w964 -> [w1024]
              tunnel: w963 -> [w1023]
              tunnel: w962 -> [w1022]
              tunnel: [w1021] -> w949 mode=indexing
              tunnel: [w1020] -> w960 mode=indexing
              tunnel: w959 -> [w1019] mode=indexing
              tunnel: w958 -> [w1018]
              tunnel: w957 -> [w1017]
              tunnel: [w1016] -> w924 mode=indexing
              tunnel: [w1015] -> w950 mode=indexing
              tunnel: w956 -> [w1014]
              tunnel: w955 -> [w1013]
              tunnel: [w1012] -> w954 mode=indexing
              tunnel: w952 -> [w1011]
              tunnel: [w1010] -> w951 mode=indexing
              tunnel: w932 -> [w1002]
              tunnel: w931 -> [w1001]
              tunnel: w930 -> [w1000]
              tunnel: [w980] -> w929 mode=indexing
              tunnel: [w979] -> w928 mode=indexing
              tunnel: w925 -> [w978]
              i -> [w977]
              n450 = Unbundle By Name(w1019) -> ("Target.X::12"=w984:refnum<vi>, "Target.Y::12"=w983:refnum<vi>)
              n451 = Index Array(array=w1002, index (row)=w977) -> (element=w1005:dbl[])  [unwired: 1 in]
              n452 = Index Array(array=w1001, index=w977) -> (element=w1004:cluster{"Ref X":refnum<vi>, "Ref Y":refnum<vi>})
              n453 = Index Array(array=w1000, index (row)=w977) -> (element=w1009:dbl[])  [unwired: 1 in]
              n454 = Index Array(array=w978, index=w977) -> (element=w976:bool)
              n455 = Index Array(array=w1023, index (row)=w977) -> (element=w996:dbl[])  [unwired: 1 in]
              n456 = Index Array(array=w1022, index (row)=w977) -> (element=w997:dbl[])  [unwired: 1 in]
              n457 = Index Array(array=w1025, index (row)=w977) -> (element=w999:dbl[])  [unwired: 1 in]
              n458 = Index Array(array=w1024, index (row)=w977) -> (element=w998:dbl[])  [unwired: 1 in]
              n459 = Index Array(array=w1018, index (row)=w977) -> (element=w992:dbl[])  [unwired: 1 in]
              n460 = Index Array(array=w1017, index (row)=w977) -> (element=w991:dbl[])  [unwired: 1 in]
              n461 = Index Array(array=w1014, index (row)=w977) -> (element=w989:dbl[])  [unwired: 1 in]
              n462 = Index Array(array=w1013, index (row)=w977) -> (element=w988:dbl[])  [unwired: 1 in]
              n463 = Index Array(array=w1011, index (row)=w977) -> (element=w985:timestamp[])  [unwired: 1 in]
              n464 = Unbundle By Name(w1004) -> ("Ref X"=w1003:refnum<vi>, "Ref Y"=w1007:refnum<vi>)
              n465 = property class="DigNum (strict)"(reference=w984) -> ("Value"=w982:dbl)  [unwired: 1 in, 2 out]
              n466 = property class="DigNum (strict)"(reference=w983) -> ("Value"=w981:dbl)  [unwired: 1 in, 2 out]
              n467 = call <vilib>:"Std Deviation and Variance.vi"("X"=w999) -> ("mean"=w995:dbl)  [unwired: 1 in, 2 out]
              n468 = call <vilib>:"Std Deviation and Variance.vi"("X"=w998) -> ("mean"=w994:dbl)  [unwired: 1 in, 2 out]
              n469 = call <vilib>:"Std Deviation and Variance.vi"("X"=w989) -> ("mean"=w987:dbl)  [unwired: 1 in, 2 out]
              n470 = Get Date/Time In Seconds() -> (seconds since 1Jan1904=w986:timestamp)
              n471 = property class="DigNum (strict)"(reference=w1003) -> ("Value"=w1006:dbl)  [unwired: 1 in, 2 out]
              n472 = property class="DigNum (strict)"(reference=w1007) -> ("Value"=w1008:dbl)  [unwired: 1 in, 2 out]
              n473 = Subtract(x=w982, y=w995) -> (x-y=w993:dbl)
              n474 = Subtract(x=w981, y=w994) -> (x-y=w990:dbl)
              n475 = case shown="True" w976 {
                tunnel: [w1038 w1057] -> w1021
                tunnel: [w1026 w1056] -> w1020
                tunnel: [w1027 w1055] -> w1016
                tunnel: [w1028 w1054] -> w1015
                tunnel: [w1029 w1053] -> w1012
                tunnel: [w1030 w1052] -> w1010
                tunnel: w997 -> [w1036 w1051]
                tunnel: w996 -> [w1037 w1050]
                tunnel: w995 -> [_ w1049]
                tunnel: w994 -> [_ w1048]
                tunnel: w993 -> [_ w1047]
                tunnel: w992 -> [w1035 w1046]
                tunnel: w991 -> [w1034 w1045]
                tunnel: w990 -> [_ w1044]
                tunnel: w988 -> [w1033 w1043]
                tunnel: w987 -> [_ w1042]
                tunnel: w986 -> [w1031 w1041]
                tunnel: w985 -> [w1032 w1040]
                frame False {
                  w1039 = 0.0
                  n476 = Build Array (concatenate)(w1037, w1039) -> (w1038:dbl[])
                  n477 = Build Array (concatenate)(w1036, w1039) -> (w1026:dbl[])
                  n478 = Build Array (concatenate)(w1035, w1039) -> (w1027:dbl[])
                  n479 = Build Array (concatenate)(w1034, w1039) -> (w1028:dbl[])
                  n480 = Build Array (concatenate)(w1033, w1039) -> (w1029:dbl[])
                  n481 = Build Array (concatenate)(w1032, w1031) -> (w1030:timestamp[])
                }
                frame True {
                  n482 = Build Array (concatenate)(w1050, w1049) -> (w1057:dbl[])
                  n483 = Build Array (concatenate)(w1051, w1048) -> (w1056:dbl[])
                  n484 = Build Array (concatenate)(w1046, w1047) -> (w1055:dbl[])
                  n485 = Build Array (concatenate)(w1045, w1044) -> (w1054:dbl[])
                  n486 = Build Array (concatenate)(w1043, w1042) -> (w1053:dbl[])
                  n487 = Build Array (concatenate)(w1040, w1041) -> (w1052:timestamp[])
                }
              }
              n488 = Build Array (concatenate)(w1005, w1006) -> (w980:dbl[])
              n489 = Build Array (concatenate)(w1009, w1008) -> (w979:dbl[])
            }
            n490 = local write "Numeric"(0.0 ("Numeric")) -> ()
            n491 = Array Size(array=w924) -> (size(s)=w948:i32[])
            n492 = Index Array(array=w948, index=1) -> (element=w946:i32)
            "History Index" <- w946
            n493 = call <vilib>:"Add State(s) to Queue__jki_lib_state_machine.vi"("State(s) in (\"\")"=w933, "State(s) at Back (\"\")"="Check Move\ntdms" ("State(s) at Back (\"\")")) -> ("States Out"=w940:string)  [unwired: 13 in]
            n494 = Unbundle By Name(w923) -> ("img to avg"=w920:i32)
            n495 = Initialize Array(0.0 ("element"), 12 ("dimension size"), w920) -> (w919:dbl[][])
            n496 = Greater?(x=w946, y="History Size") -> (0:w944:bool)
            n497 = Bundle By Name(cluster=w923, "Centroid X"=w919, "Centroid Y"=w919, "Mean Centroid X"=w949, "Mean Centroid Y"=w960, "Offset X"=w924, "Offset Y"=w950, "Mean Size"=w954, "Size"=w919, "Time"=w951, "Motor X"=w929, "Motor Y"=w928) -> (w961:T37)
            n498 = Select(t="history" ("State(s) at Back (\"\")"), s=w944, f="") -> (s? t:f=w941:string)
            n499 = call <vilib>:"Add State(s) to Queue__jki_lib_state_machine.vi"("State(s) in (\"\")"=w940, "State(s) at Back (\"\")"=w941) -> ("States Out"=w939:string)  [unwired: 13 in]
          }
          frame "Check Move" {
            (unwired) "Device Ini" ("State(s) in Front (\"\")")
            n500 = Unbundle By Name(w1062) -> ("move properties"=w1076:T2[], "Mean Size"=w1075:dbl[][], "move properties"=w1074:T2[], "Offset X"=w1073:dbl[][], "Offset Y"=w1072:dbl[][], "active cams"=w1071:string[])
            n501 = Unbundle By Name(w1062) -> ("steps speed X"=w1061:dbl[], "steps speed Y"=w1060:dbl[])
            n502 = for {
              tunnel: w1074 -> [w1119]
              tunnel: w1073 -> [w1117]
              tunnel: w1072 -> [w1115]
              tunnel: w1075 -> [w1122]
              tunnel: [w1113] -> w1070 mode=indexing
              tunnel: [w1126] -> w1069 mode=indexing
              tunnel: w1071 -> [w1123] mode=indexing
              tunnel: [w1147] -> w1077 mode=indexing
              tunnel: [w1146] -> w1067 mode=indexing
              tunnel: w1076 -> [w1106]
              tunnel: [w1108] -> w1066 mode=indexing
              tunnel: [w1107] -> w1065 mode=indexing
              tunnel: "Speedmode @" -> [w1112]
              tunnel: w1063 -> [w1124]
              shift-right: [w1099] -> w1059
              shift-left: w1061 -> [w1104]
              shift-right: [w1098] -> w1058
              shift-left: w1060 -> [w1103]
              n503 = call-poly <userlib>:"Filter 1D Array__ogtk.vi"("items to filter"=w1123, "array"=w1124) -> ("filtered item indices"=w1125:i32[])  [unwired: 4 in, 1 out]
              n504 = Index Array(array=w1125) -> (element=w1102:i32)  [unwired: 1 in]
              n505 = Index Array(array=w1106, index=w1102) -> (element=w1121:T2)
              n506 = Index Array(array=w1122, index (row)=w1102) -> (element=w1120:dbl[])  [unwired: 1 in]
              n507 = Index Array(array=w1119, index=w1102) -> (element=w1118:T2)
              n508 = Index Array(array=w1117, index (row)=w1102) -> (element=w1116:dbl[])  [unwired: 1 in]
              n509 = Index Array(array=w1115, index (row)=w1102) -> (element=w1114:dbl[])  [unwired: 1 in]
              n510 = Unbundle By Name(w1118) -> ("Tolerance [%]"=w1140:dbl)
              n511 = Reverse 1D Array(array=w1116) -> (reversed array=w1145:dbl[])
              n512 = Reverse 1D Array(array=w1114) -> (reversed array=w1144:dbl[])
              n513 = Reverse 1D Array(array=w1120) -> (reversed array=w1139:dbl[])
              n514 = Unbundle By Name(w1121) -> ("Stepsize"=w1105:dbl, "enable feedback"=w1129:bool)
              n515 = Index Array(array=w1145) -> (element=w1143:dbl)  [unwired: 1 in]
              n516 = Index Array(array=w1144) -> (element=w1142:dbl)  [unwired: 1 in]
              n517 = Index Array(array=w1139) -> (element=w1138:dbl)  [unwired: 1 in]
              n518 = Absolute Value(x=w1143) -> (abs(x)=w1109:dbl)
              n519 = Absolute Value(x=w1142) -> (abs(x)=w1110:dbl)
              n520 = Square Root(x=w1138) -> (sqrt(x)=w1137:dbl)
              n521 = Divide(x=w1140, y=100.0) -> (x/y=w1136:dbl)
              n522 = Multiply(x=w1137, y=w1136) -> (x*y=w1111:dbl)
              n523 = Not Equal To 0?(x=w1110) -> (x != 0?=w1127:bool)
              n524 = Not Equal To 0?(x=w1109) -> (x != 0?=w1131:bool)
              n525 = Greater Or Equal?(x=w1109, y=w1111) -> (x >= y?=w1130:bool)
              n526 = Greater Or Equal?(x=w1110, y=w1111) -> (x >= y?=w1128:bool)
              n527 = Compound Arithmetic op=AND(w1129, w1131, w1130) -> (w1113:bool)
              n528 = Compound Arithmetic op=AND(w1129, w1128, w1127) -> (w1126:bool)
              n529 = call "speedmode.vi"("offset X"=w1109, "offset Y"=w1110, "beamsize x tolerance"=w1111, "Speedmode @"=w1112, "step size"=w1105) -> ("steps speed Y"=w1100:dbl, "steps speed X"=w1101:dbl, "speedmode X"=w1108:bool, "speedmode Y"=w1107:bool)  [unwired: 3 in]
              n530 = Boolean To (0,1)(Boolean=w1126) -> (0, 1=w1132:i16)
              n531 = Replace Array Subset(array=w1103, new element=w1100, index=w1102) -> (w1098:dbl[])
              n532 = Replace Array Subset(array=w1104, new element=w1101, index=w1102) -> (w1099:dbl[])
              n533 = Multiply(x=w1132, y=w1110) -> (x*y=w1133:dbl)
              n534 = Boolean To (0,1)(Boolean=w1113) -> (0, 1=w1135:i16)
              n535 = Multiply(x=w1135, y=w1109) -> (x*y=w1134:dbl)
              n536 = Bundle(w1133, "GUIdevice 8"=w1123) -> (w1146:cluster{dbl, "GUIdevice 8":string})  [unwired: 1 in]
              n537 = Bundle(w1134, "GUIdevice 8"=w1123) -> (w1147:cluster{dbl, "GUIdevice 8":string})  [unwired: 1 in]
            }
            "required X" <- w1070
            "required Y" <- w1069
            "speedmode X" <- w1066
            "speedmode Y" <- w1065
            n538 = case shown="True" "Align" {
              tunnel: w1077 -> [w1153 w1158]
              tunnel: w1067 -> [w1152 w1155]
              tunnel: [w1151 w1157] -> w1080
              tunnel: [w1150 w1154] -> w1079
              frame False {
                n539 = Sort 1D Array(array=w1152) -> (sorted array=w1149:cluster{dbl, "GUIdevice 8":string}[])
                n540 = Sort 1D Array(array=w1153) -> (sorted array=w1148:cluster{dbl, "GUIdevice 8":string}[])
                n541 = Reverse 1D Array(array=w1149) -> (reversed array=w1150:cluster{dbl, "GUIdevice 8":string}[])
                n542 = Reverse 1D Array(array=w1148) -> (reversed array=w1151:cluster{dbl, "GUIdevice 8":string}[])
              }
              frame True {
                w1156 = cluster{dbl, "GUIdevice 8":string}[] [] ("Array")
                n543 = for {
                  shift-right: [w1168] -> w1157
                  shift-left: w1156 -> [w1170]
                  tunnel: w1158 -> [w1169] mode=indexing
                  n544 = Unbundle(w1169) -> (w1172:dbl)  [unwired: 1 out]
                  n545 = Not Equal To 0?(x=w1172) -> (x != 0?=w1171:bool)
                  n546 = case shown="True" w1171 {
                    tunnel: w1170 -> [w1173 w1176]
                    tunnel: w1169 -> [_ w1175]
                    tunnel: [w1173 w1174] -> w1168
                    frame False {
                    }
                    frame True {
                      n547 = Build Array (concatenate)(w1176, w1175) -> (w1174:cluster{dbl, "GUIdevice 8":string}[])
                    }
                  }
                }
                n548 = for {
                  shift-right: [w1159] -> w1154
                  shift-left: w1156 -> [w1161]
                  tunnel: w1155 -> [w1160] mode=indexing
                  n549 = Unbundle(w1160) -> (w1163:dbl)  [unwired: 1 out]
                  n550 = Not Equal To 0?(x=w1163) -> (x != 0?=w1162:bool)
                  n551 = case shown="True" w1162 {
                    tunnel: w1161 -> [w1164 w1167]
                    tunnel: w1160 -> [_ w1166]
                    tunnel: [w1164 w1165] -> w1159
                    frame False {
                    }
                    frame True {
                      n552 = Build Array (concatenate)(w1167, w1166) -> (w1165:cluster{dbl, "GUIdevice 8":string}[])
                    }
                  }
                }
              }
            }
            n553 = call <vilib>:"Add State(s) to Queue__jki_lib_state_machine.vi"("State(s) in (\"\")"=w1083) -> ("States Out"=w1082:string)  [unwired: 14 in]
            n554 = Bundle By Name(cluster=w1062, "steps speed X"=w1059, "steps speed Y"=w1058, "speedmode X"=w1066, "speedmode Y"=w1065) -> (w1064:T37)
            n555 = Index Array(array=w1079) -> (element=w1084:cluster{dbl, "GUIdevice 8":string})  [unwired: 1 in]
            n556 = Index Array(array=w1080) -> (element=w1085:cluster{dbl, "GUIdevice 8":string})  [unwired: 1 in]
            n557 = Empty Array?(array=w1079) -> (empty?=w1087:bool)
            n558 = Unbundle(w1085) -> (w1093:dbl)  [unwired: 1 out]
            n559 = Unbundle(w1084) -> (w1089:dbl)  [unwired: 1 out]
            n560 = Unbundle By Name(w1064) -> ("Feedback global"=w1094:bool)
            n561 = Empty Array?(array=w1080) -> (empty?=w1091:bool)
            n562 = property on="autodetect" class="Bool (strict)"("Value"=FALSE ("autodetect")) -> ()  [unwired: 2 in, 2 out]
            n563 = Equal To 0?(x=w1093) -> (x = 0?=w1092:bool)
            n564 = Equal To 0?(x=w1089) -> (x = 0?=w1088:bool)
            n565 = Or(x=w1092, y=w1091) -> (x .or. y?=w1090:bool)
            n566 = Or(x=w1088, y=w1087) -> (x .or. y?=w1086:bool)
            n567 = case shown="True" w1094 {
              tunnel: w1090 -> [_ w1184]
              tunnel: w1080 -> [_ w1183]
              tunnel: w1086 -> [_ w1181]
              tunnel: w1079 -> [_ w1180]
              tunnel: w1082 -> [w1177 w1179]
              tunnel: [w1177 w1178] -> w1095
              frame False {
              }
              frame True {
                n568 = case shown="False" w1184 {
                  tunnel: w1183 -> [w1200 _]
                  tunnel: w1179 -> [w1196 w1201]
                  tunnel: [w1194 w1201] -> w1182
                  frame False {
                    n569 = Index Array(array=w1200) -> (element=w1199:cluster{dbl, "GUIdevice 8":string})  [unwired: 1 in]
                    n570 = Unbundle By Name(w1199) -> ("GUIdevice 8"=w1198:string)
                    n571 = Wait (ms)(milliseconds to wait=u32 100) -> ()  [unwired: 1 out]
                    n572 = call <vilib>:"Build State String with Arguments__jki_lib_state_machine.vi"("Arguments (\"\")"=w1198, "State"="Move X") -> ("State with Arguments"=w1195:string)  [unwired: 4 in]
                    n573 = call <vilib>:"Add State(s) to Queue__jki_lib_state_machine.vi"("State(s) in (\"\")"=w1196, "State(s) at Back (\"\")"=w1195) -> ("States Out"=w1194:string)  [unwired: 13 in]
                  }
                  frame True {
                  }
                }
                n574 = case shown="False" w1181 {
                  tunnel: w1180 -> [w1191 _]
                  tunnel: w1182 -> [w1187 w1192]
                  tunnel: [w1185 w1192] -> w1178
                  frame False {
                    n575 = Index Array(array=w1191) -> (element=w1190:cluster{dbl, "GUIdevice 8":string})  [unwired: 1 in]
                    n576 = Unbundle By Name(w1190) -> ("GUIdevice 8"=w1189:string)
                    n577 = call <vilib>:"Build State String with Arguments__jki_lib_state_machine.vi"("Arguments (\"\")"=w1189, "State"="Move Y") -> ("State with Arguments"=w1186:string)  [unwired: 4 in]
                    n578 = call <vilib>:"Add State(s) to Queue__jki_lib_state_machine.vi"("State(s) in (\"\")"=w1187, "State(s) at Back (\"\")"=w1186) -> ("States Out"=w1185:string)  [unwired: 13 in]
                  }
                  frame True {
                  }
                }
              }
            }
            n579 = call <vilib>:"Add State(s) to Queue__jki_lib_state_machine.vi"("State(s) in (\"\")"=w1082, "State(s) at Back (\"\")"=w1095) -> ("States Out"=w1097:string)  [unwired: 13 in]
          }
          frame "Move X" {
            # "Your code here.\n(You can make a copy of, or modify, this frame)"
            n580 = Unbundle By Name(w1205) -> ("Offset X"=w1225:dbl[][])
            n581 = call-poly <userlib>:"Filter 1D Array__ogtk.vi"("items to filter"=w1211, "array"=w1229) -> ("filtered item indices"=w1216:i32[])  [unwired: 4 in, 1 out]
            n582 = Unbundle By Name(w1205) -> ("active axis refs 2"=w1228:T11, "move properties"=w1215:T2[])
            n583 = for {
              tunnel: w1216 -> [w1234] mode=indexing
              tunnel: w1215 -> [w1238]
              shift-right: [w1233] -> w1213
              shift-left: i32[] [] ("filtered item indices") -> [w1236]
              n584 = Index Array(array=w1238, index=w1234) -> (element=w1237:T2)
              n585 = Unbundle By Name(w1237) -> ("enable feedback"=w1235:bool)
              n586 = case shown="True" w1235 {
                tunnel: w1236 -> [w1239 w1242]
                tunnel: w1234 -> [_ w1241]
                tunnel: [w1239 w1240] -> w1233
                frame False {
                }
                frame True {
                  n587 = Build Array (concatenate)(w1242, w1241) -> (w1240:i32[])
                }
              }
            }
            n588 = Index Array(array=w1213) -> (element=w1204:i32)  [unwired: 1 in]
            n589 = Index Array(array=w1225, index (row)=w1204) -> (element=w1224:dbl[])  [unwired: 1 in]
            n590 = Reverse 1D Array(array=w1224) -> (reversed array=w1223:dbl[])
            n591 = Index Array(array=w1228, index=w1204) -> (element=w1227:cluster{"Ref X":refnum<vi>, "Ref Y":refnum<vi>})
            n592 = Index Array(array=w1223) -> (element=w1221:dbl)  [unwired: 1 in]
            n593 = Index Array(array=w1215, index=w1204) -> (element=w1226:T2)
            n594 = Unbundle By Name(w1227) -> ("Ref X"=w1219:refnum<vi>, "Ref Y"=w1218:refnum<vi>)
            n595 = Unbundle By Name(w1226) -> ("Invert Direction X"=w1203:bool, "Invert Axis"=w1222:bool, "enable feedback"=w1217:bool)
            n596 = Greater Or Equal To 0?(x=w1221) -> (x >= 0?=w1220:bool)
            n597 = Unbundle By Name(w1205) -> ("steps speed Y"=w1206:dbl[], "steps speed X"=w1207:dbl[])
            n598 = Index Array(array=w1207, index=w1204) -> (element=w1209:dbl)
            n599 = Index Array(array=w1206, index=w1204) -> (element=w1208:dbl)
            n600 = Select(t=w1208, s=w1203, f=w1209) -> (s? t:f=w1202:dbl)
            n601 = case shown="True" w1217 {
              tunnel: w1222 -> [_ w1248]
              tunnel: w1220 -> [_ w1247]
              tunnel: w1202 -> [_ w1246]
              tunnel: w1203 -> [_ w1245]
              tunnel: w1219 -> [_ w1244]
              tunnel: w1218 -> [_ w1243]
              frame False {
              }
              frame True {
                n602 = case shown="False" w1247 {
                  tunnel: w1245 -> [w1256 w1278]
                  tunnel: w1246 -> [w1254 w1276]
                  tunnel: w1248 -> [w1253 w1275]
                  tunnel: w1248 -> [w1252 w1274]
                  tunnel: w1244 -> [w1250 w1272]
                  tunnel: w1243 -> [w1249 w1271]
                  frame True {
                    n603 = case shown="False" w1253 {
                      tunnel: [w1267 w1269] -> w1255
                      tunnel: w1250 -> [w1268 _]
                      tunnel: w1249 -> [_ w1270]
                      frame False {
                        n604 = property class="DigNum (strict)"(reference=w1268) -> ("Value"=w1267:dbl)  [unwired: 1 in, 2 out]
                      }
                      frame True {
                        n605 = property class="DigNum (strict)"(reference=w1270) -> ("Value"=w1269:dbl)  [unwired: 1 in, 2 out]
                      }
                    }
                    n606 = case shown="False" w1256 {
                      tunnel: w1255 -> [w1263 w1266]
                      tunnel: w1254 -> [w1262 w1265]
                      tunnel: [w1261 w1264] -> w1251
                      frame False {
                        n607 = Add(x=w1263, y=w1262) -> (x+y=w1261:dbl)
                      }
                      frame True {
                        n608 = Subtract(x=w1266, y=w1265) -> (x-y=w1264:dbl)
                      }
                    }
                    n609 = case shown="False" w1252 {
                      tunnel: w1251 -> [w1257 w1259]
                      tunnel: w1250 -> [w1258 _]
                      tunnel: w1249 -> [_ w1260]
                      frame False {
                        n610 = property class="DigNum (strict)"(reference=w1258, "Val(Sgnl)"=w1257) -> ()  [unwired: 1 in, 2 out]
                      }
                      frame True {
                        n611 = property class="DigNum (strict)"(reference=w1260, "Val(Sgnl)"=w1259) -> ()  [unwired: 1 in, 2 out]
                      }
                    }
                  }
                  frame False {
                    n612 = case shown="False" w1275 {
                      tunnel: [w1289 w1291] -> w1277
                      tunnel: w1272 -> [w1290 _]
                      tunnel: w1271 -> [_ w1292]
                      frame False {
                        n613 = property class="DigNum (strict)"(reference=w1290) -> ("Value"=w1289:dbl)  [unwired: 1 in, 2 out]
                      }
                      frame True {
                        n614 = property class="DigNum (strict)"(reference=w1292) -> ("Value"=w1291:dbl)  [unwired: 1 in, 2 out]
                      }
                    }
                    n615 = case shown="False" w1278 {
                      tunnel: w1277 -> [w1285 w1288]
                      tunnel: w1276 -> [w1284 w1287]
                      tunnel: [w1283 w1286] -> w1273
                      frame False {
                        n616 = Subtract(x=w1285, y=w1284) -> (x-y=w1283:dbl)
                      }
                      frame True {
                        n617 = Add(x=w1288, y=w1287) -> (x+y=w1286:dbl)
                      }
                    }
                    n618 = case shown="False" w1274 {
                      tunnel: w1273 -> [w1279 w1281]
                      tunnel: w1272 -> [w1280 _]
                      tunnel: w1271 -> [_ w1282]
                      frame False {
                        n619 = property class="DigNum (strict)"(reference=w1280, "Val(Sgnl)"=w1279) -> ()  [unwired: 1 in, 2 out]
                      }
                      frame True {
                        n620 = property class="DigNum (strict)"(reference=w1282, "Val(Sgnl)"=w1281) -> ()  [unwired: 1 in, 2 out]
                      }
                    }
                  }
                }
              }
            }
            n621 = call <vilib>:"Build State String with Arguments__jki_lib_state_machine.vi"("Arguments (\"\")"=w1211, "State"="Wait" ("State(s) in Front (\"\")")) -> ("State with Arguments"=w1210:string)  [unwired: 4 in]
            n622 = call <vilib>:"Add State(s) to Queue__jki_lib_state_machine.vi"("State(s) in Front (\"\")"=w1210, "State(s) in (\"\")"=w1232) -> ("States Out"=w1231:string)  [unwired: 13 in]
            "Moving X" <- w1211
          }
          frame "ManMove X" {
            # "Your code here.\n(You can make a copy of, or modify, this frame)"
            n623 = Equal?(x=w1298, y="Right") -> (x = y?=w1299:bool)
            n624 = Unbundle By Name(w1308) -> ("move properties"=w1303:T2[], "active ccd"=w1296:i32, "active man refs"=w1301:cluster{"Ref X":refnum<vi>, "Ref Y":refnum<vi>}, "active cams"=w1297:string[])
            n625 = Index Array(array=w1297, index=w1296) -> (element=w1294:string)
            n626 = Index Array(array=w1303, index=w1296) -> (element=w1309:T2)
            n627 = Unbundle By Name(w1301) -> ("Ref X"=w1305:refnum<vi>, "Ref Y"=w1304:refnum<vi>)
            n628 = Unbundle By Name(w1309) -> ("Invert Direction X"=w1306:bool, "Invert Axis"=w1307:bool)
            n629 = call <vilib>:"Build State String with Arguments__jki_lib_state_machine.vi"("Arguments (\"\")"=w1294, "State"="Wait" ("State(s) in Front (\"\")")) -> ("State with Arguments"=w1293:string)  [unwired: 4 in]
            n630 = call <vilib>:"Add State(s) to Queue__jki_lib_state_machine.vi"("State(s) in Front (\"\")"=w1293, "State(s) in (\"\")"=w1312) -> ("States Out"=w1311:string)  [unwired: 13 in]
            n631 = case shown="False" w1299 {
              tunnel: w1306 -> [w1320 w1342]
              tunnel: "StepSize" -> [w1318 w1340]
              tunnel: w1307 -> [w1317 w1339]
              tunnel: w1307 -> [w1316 w1338]
              tunnel: w1305 -> [w1314 w1336]
              tunnel: w1304 -> [w1313 w1335]
              frame True {
                n632 = case shown="False" w1317 {
                  tunnel: [w1331 w1333] -> w1319
                  tunnel: w1314 -> [w1332 _]
                  tunnel: w1313 -> [_ w1334]
                  frame False {
                    n633 = property class="DigNum (strict)"(reference=w1332) -> ("Value"=w1331:dbl)  [unwired: 1 in, 2 out]
                  }
                  frame True {
                    n634 = property class="DigNum (strict)"(reference=w1334) -> ("Value"=w1333:dbl)  [unwired: 1 in, 2 out]
                  }
                }
                n635 = case shown="False" w1320 {
                  tunnel: w1319 -> [w1327 w1330]
                  tunnel: w1318 -> [w1326 w1329]
                  tunnel: [w1325 w1328] -> w1315
                  frame False {
                    n636 = Add(x=w1327, y=w1326) -> (x+y=w1325:dbl)
                  }
                  frame True {
                    n637 = Subtract(x=w1330, y=w1329) -> (x-y=w1328:dbl)
                  }
                }
                n638 = case shown="False" w1316 {
                  tunnel: w1315 -> [w1321 w1323]
                  tunnel: w1314 -> [w1322 _]
                  tunnel: w1313 -> [_ w1324]
                  frame False {
                    n639 = property class="DigNum (strict)"(reference=w1322, "Val(Sgnl)"=w1321) -> ()  [unwired: 1 in, 2 out]
                  }
                  frame True {
                    n640 = property class="DigNum (strict)"(reference=w1324, "Val(Sgnl)"=w1323) -> ()  [unwired: 1 in, 2 out]
                  }
                }
              }
              frame False {
                n641 = case shown="False" w1339 {
                  tunnel: [w1353 w1355] -> w1341
                  tunnel: w1336 -> [w1354 _]
                  tunnel: w1335 -> [_ w1356]
                  frame False {
                    n642 = property class="DigNum (strict)"(reference=w1354) -> ("Value"=w1353:dbl)  [unwired: 1 in, 2 out]
                  }
                  frame True {
                    n643 = property class="DigNum (strict)"(reference=w1356) -> ("Value"=w1355:dbl)  [unwired: 1 in, 2 out]
                  }
                }
                n644 = case shown="True" w1342 {
                  tunnel: w1341 -> [w1349 w1352]
                  tunnel: w1340 -> [w1348 w1351]
                  tunnel: [w1347 w1350] -> w1337
                  frame False {
                    n645 = Subtract(x=w1349, y=w1348) -> (x-y=w1347:dbl)
                  }
                  frame True {
                    n646 = Add(x=w1352, y=w1351) -> (x+y=w1350:dbl)
                  }
                }
                n647 = case shown="False" w1338 {
                  tunnel: w1337 -> [w1343 w1345]
                  tunnel: w1336 -> [w1344 _]
                  tunnel: w1335 -> [_ w1346]
                  frame False {
                    n648 = property class="DigNum (strict)"(reference=w1344, "Val(Sgnl)"=w1343) -> ()  [unwired: 1 in, 2 out]
                  }
                  frame True {
                    n649 = property class="DigNum (strict)"(reference=w1346, "Val(Sgnl)"=w1345) -> ()  [unwired: 1 in, 2 out]
                  }
                }
              }
            }
          }
          frame "ManMove Y" {
            # "Your code here.\n(You can make a copy of, or modify, this frame)"
            n650 = Equal?(x=w1362, y="Down") -> (x = y?=w1366:bool)
            n651 = Unbundle By Name(w1372) -> ("active cams"=w1361:string[], "move properties"=w1371:T2[], "active ccd"=w1360:i32, "active man refs"=w1370:cluster{"Ref X":refnum<vi>, "Ref Y":refnum<vi>})
            n652 = Index Array(array=w1361, index=w1360) -> (element=w1358:string)
            n653 = property on="StepSize" class="DigNum (strict)"() -> ("Value"=w1363:dbl)  [unwired: 2 in, 2 out]
            n654 = Index Array(array=w1371, index=w1360) -> (element=w1373:T2)
            n655 = Unbundle By Name(w1370) -> ("Ref Y"=w1365:refnum<vi>, "Ref X"=w1364:refnum<vi>)
            n656 = Unbundle By Name(w1373) -> ("Invert Direction Y"=w1368:bool, "Invert Axis"=w1367:bool)
            n657 = call <vilib>:"Build State String with Arguments__jki_lib_state_machine.vi"("Arguments (\"\")"=w1358, "State"="Wait" ("State(s) in Front (\"\")")) -> ("State with Arguments"=w1357:string)  [unwired: 4 in]
            n658 = call <vilib>:"Add State(s) to Queue__jki_lib_state_machine.vi"("State(s) in Front (\"\")"=w1357, "State(s) in (\"\")"=w1376) -> ("States Out"=w1375:string)  [unwired: 13 in]
            n659 = case shown="True" w1366 {
              tunnel: w1368 -> [w1384 w1406]
              tunnel: w1363 -> [w1382 w1404]
              tunnel: w1367 -> [w1381 w1403]
              tunnel: w1367 -> [w1380 w1402]
              tunnel: w1365 -> [w1378 w1400]
              tunnel: w1364 -> [w1377 w1399]
              frame True {
                n660 = case shown="False" w1381 {
                  tunnel: [w1395 w1397] -> w1383
                  tunnel: w1378 -> [w1396 _]
                  tunnel: w1377 -> [_ w1398]
                  frame False {
                    n661 = property class="DigNum (strict)"(reference=w1396) -> ("Value"=w1395:dbl)  [unwired: 1 in, 2 out]
                  }
                  frame True {
                    n662 = property class="DigNum (strict)"(reference=w1398) -> ("Value"=w1397:dbl)  [unwired: 1 in, 2 out]
                  }
                }
                n663 = case shown="False" w1384 {
                  tunnel: w1383 -> [w1391 w1394]
                  tunnel: w1382 -> [w1390 w1393]
                  tunnel: [w1389 w1392] -> w1379
                  frame False {
                    n664 = Add(x=w1391, y=w1390) -> (x+y=w1389:dbl)
                  }
                  frame True {
                    n665 = Subtract(x=w1394, y=w1393) -> (x-y=w1392:dbl)
                  }
                }
                n666 = case shown="False" w1380 {
                  tunnel: w1379 -> [w1385 w1387]
                  tunnel: w1378 -> [w1386 _]
                  tunnel: w1377 -> [_ w1388]
                  frame False {
                    n667 = property class="DigNum (strict)"(reference=w1386, "Val(Sgnl)"=w1385) -> ()  [unwired: 1 in, 2 out]
                  }
                  frame True {
                    n668 = property class="DigNum (strict)"(reference=w1388, "Val(Sgnl)"=w1387) -> ()  [unwired: 1 in, 2 out]
                  }
                }
              }
              frame False {
                n669 = case shown="False" w1403 {
                  tunnel: [w1417 w1419] -> w1405
                  tunnel: w1400 -> [w1418 _]
                  tunnel: w1399 -> [_ w1420]
                  frame False {
                    n670 = property class="DigNum (strict)"(reference=w1418) -> ("Value"=w1417:dbl)  [unwired: 1 in, 2 out]
                  }
                  frame True {
                    n671 = property class="DigNum (strict)"(reference=w1420) -> ("Value"=w1419:dbl)  [unwired: 1 in, 2 out]
                  }
                }
                n672 = case shown="False" w1406 {
                  tunnel: w1405 -> [w1413 w1416]
                  tunnel: w1404 -> [w1412 w1415]
                  tunnel: [w1411 w1414] -> w1401
                  frame False {
                    n673 = Subtract(x=w1413, y=w1412) -> (x-y=w1411:dbl)
                  }
                  frame True {
                    n674 = Add(x=w1416, y=w1415) -> (x+y=w1414:dbl)
                  }
                }
                n675 = case shown="False" w1402 {
                  tunnel: w1401 -> [w1407 w1409]
                  tunnel: w1400 -> [w1408 _]
                  tunnel: w1399 -> [_ w1410]
                  frame False {
                    n676 = property class="DigNum (strict)"(reference=w1408, "Val(Sgnl)"=w1407) -> ()  [unwired: 1 in, 2 out]
                  }
                  frame True {
                    n677 = property class="DigNum (strict)"(reference=w1410, "Val(Sgnl)"=w1409) -> ()  [unwired: 1 in, 2 out]
                  }
                }
              }
            }
          }
          frame "Move Y" {
            # "Your code here.\n(You can make a copy of, or modify, this frame)"
            n678 = Unbundle By Name(w1428) -> ("Offset Y"=w1444:dbl[][])
            n679 = call-poly <userlib>:"Filter 1D Array__ogtk.vi"("items to filter"=w1430, "array"=w1448) -> ("filtered item indices"=w1435:i32[])  [unwired: 4 in, 1 out]
            n680 = Unbundle By Name(w1428) -> ("active axis refs 2"=w1447:T11, "move properties"=w1433:T2[])
            n681 = for {
              tunnel: w1435 -> [w1453] mode=indexing
              tunnel: w1433 -> [w1457]
              shift-right: [w1452] -> w1434
              shift-left: i32[] [] ("filtered item indices") -> [w1455]
              n682 = Index Array(array=w1457, index=w1453) -> (element=w1456:T2)
              n683 = Unbundle By Name(w1456) -> ("enable feedback"=w1454:bool)
              n684 = case shown="True" w1454 {
                tunnel: w1455 -> [w1458 w1461]
                tunnel: w1453 -> [_ w1460]
                tunnel: [w1458 w1459] -> w1452
                frame False {
                }
                frame True {
                  n685 = Build Array (concatenate)(w1461, w1460) -> (w1459:i32[])
                }
              }
            }
            n686 = Index Array(array=w1434) -> (element=w1425:i32)  [unwired: 1 in]
            n687 = Index Array(array=w1444, index (row)=w1425) -> (element=w1443:dbl[])  [unwired: 1 in]
            n688 = Reverse 1D Array(array=w1443) -> (reversed array=w1442:dbl[])
            n689 = Index Array(array=w1447, index=w1425) -> (element=w1446:cluster{"Ref X":refnum<vi>, "Ref Y":refnum<vi>})
            n690 = Index Array(array=w1442) -> (element=w1440:dbl)  [unwired: 1 in]
            n691 = Index Array(array=w1433, index=w1425) -> (element=w1445:T2)
            n692 = Unbundle By Name(w1446) -> ("Ref Y"=w1438:refnum<vi>, "Ref X"=w1437:refnum<vi>)
            n693 = Unbundle By Name(w1428) -> ("steps speed X"=w1427:dbl[], "steps speed Y"=w1426:dbl[])
            n694 = Unbundle By Name(w1445) -> ("Invert Direction Y"=w1422:bool, "Invert Axis"=w1441:bool, "enable feedback"=w1436:bool)
            n695 = Greater Or Equal To 0?(x=w1440) -> (x >= 0?=w1439:bool)
            n696 = Index Array(array=w1427, index=w1425) -> (element=w1424:dbl)
            n697 = Index Array(array=w1426, index=w1425) -> (element=w1423:dbl)
            n698 = Select(t=w1424, s=w1422, f=w1423) -> (s? t:f=w1421:dbl)
            n699 = case shown="True" w1436 {
              tunnel: w1441 -> [_ w1467]
              tunnel: w1439 -> [_ w1466]
              tunnel: w1421 -> [_ w1465]
              tunnel: w1422 -> [_ w1464]
              tunnel: w1438 -> [_ w1463]
              tunnel: w1437 -> [_ w1462]
              frame False {
              }
              frame True {
                n700 = case shown="True" w1466 {
                  tunnel: w1464 -> [w1475 w1497]
                  tunnel: w1465 -> [w1473 w1495]
                  tunnel: w1467 -> [w1472 w1494]
                  tunnel: w1467 -> [w1471 w1493]
                  tunnel: w1463 -> [w1469 w1491]
                  tunnel: w1462 -> [w1468 w1490]
                  frame True {
                    n701 = case shown="False" w1472 {
                      tunnel: [w1486 w1488] -> w1474
                      tunnel: w1469 -> [w1487 _]
                      tunnel: w1468 -> [_ w1489]
                      frame False {
                        n702 = property class="DigNum (strict)"(reference=w1487) -> ("Value"=w1486:dbl)  [unwired: 1 in, 2 out]
                      }
                      frame True {
                        n703 = property class="DigNum (strict)"(reference=w1489) -> ("Value"=w1488:dbl)  [unwired: 1 in, 2 out]
                      }
                    }
                    n704 = case shown="False" w1475 {
                      tunnel: w1474 -> [w1482 w1485]
                      tunnel: w1473 -> [w1481 w1484]
                      tunnel: [w1480 w1483] -> w1470
                      frame False {
                        n705 = Add(x=w1482, y=w1481) -> (x+y=w1480:dbl)
                      }
                      frame True {
                        n706 = Subtract(x=w1485, y=w1484) -> (x-y=w1483:dbl)
                      }
                    }
                    n707 = case shown="False" w1471 {
                      tunnel: w1470 -> [w1476 w1478]
                      tunnel: w1469 -> [w1477 _]
                      tunnel: w1468 -> [_ w1479]
                      frame False {
                        n708 = property class="DigNum (strict)"(reference=w1477, "Val(Sgnl)"=w1476) -> ()  [unwired: 1 in, 2 out]
                      }
                      frame True {
                        n709 = property class="DigNum (strict)"(reference=w1479, "Val(Sgnl)"=w1478) -> ()  [unwired: 1 in, 2 out]
                      }
                    }
                  }
                  frame False {
                    n710 = case shown="False" w1494 {
                      tunnel: [w1508 w1510] -> w1496
                      tunnel: w1491 -> [w1509 _]
                      tunnel: w1490 -> [_ w1511]
                      frame False {
                        n711 = property class="DigNum (strict)"(reference=w1509) -> ("Value"=w1508:dbl)  [unwired: 1 in, 2 out]
                      }
                      frame True {
                        n712 = property class="DigNum (strict)"(reference=w1511) -> ("Value"=w1510:dbl)  [unwired: 1 in, 2 out]
                      }
                    }
                    n713 = case shown="False" w1497 {
                      tunnel: w1496 -> [w1504 w1507]
                      tunnel: w1495 -> [w1503 w1506]
                      tunnel: [w1502 w1505] -> w1492
                      frame False {
                        n714 = Subtract(x=w1504, y=w1503) -> (x-y=w1502:dbl)
                      }
                      frame True {
                        n715 = Add(x=w1507, y=w1506) -> (x+y=w1505:dbl)
                      }
                    }
                    n716 = case shown="False" w1493 {
                      tunnel: w1492 -> [w1498 w1500]
                      tunnel: w1491 -> [w1499 _]
                      tunnel: w1490 -> [_ w1501]
                      frame False {
                        n717 = property class="DigNum (strict)"(reference=w1499, "Val(Sgnl)"=w1498) -> ()  [unwired: 1 in, 2 out]
                      }
                      frame True {
                        n718 = property class="DigNum (strict)"(reference=w1501, "Val(Sgnl)"=w1500) -> ()  [unwired: 1 in, 2 out]
                      }
                    }
                  }
                }
              }
            }
            n719 = call <vilib>:"Build State String with Arguments__jki_lib_state_machine.vi"("Arguments (\"\")"=w1430, "State"="Wait" ("State(s) in Front (\"\")")) -> ("State with Arguments"=w1429:string)  [unwired: 4 in]
            n720 = call <vilib>:"Add State(s) to Queue__jki_lib_state_machine.vi"("State(s) in Front (\"\")"=w1429, "State(s) in (\"\")"=w1451) -> ("States Out"=w1450:string)  [unwired: 13 in]
            "Moving Y" <- w1430
          }
          frame "Wait" {
            # "Your code here.\n(You can make a copy of, or modify, this frame)"
            n721 = flat-sequence {
              tunnel: T20."Disabled and Grayed Out" ("Disabled") -> [w1528]
              tunnel: w1518 -> [w1537]
              tunnel: w1517 -> [w1536]
              tunnel: [w1535] -> w1516
              tunnel: w1515 -> [w1534]
              tunnel: w1514 -> [w1533]
              tunnel: T20."Enabled" ("Disabled") -> [w1547]
              frame #0 {
                n722 = property on="Right" class="Bool (strict)"("DisabledEnum"=w1528) -> ()  [unwired: 2 in, 2 out]
                n723 = property on="Up" class="Bool (strict)"("DisabledEnum"=w1528) -> ()  [unwired: 2 in, 2 out]
                n724 = property on="Left" class="Bool (strict)"("DisabledEnum"=w1528) -> ()  [unwired: 2 in, 2 out]
                n725 = property on="Down" class="Bool (strict)"("DisabledEnum"=w1528) -> ()  [unwired: 2 in, 2 out]
                n726 = property on="StepSize" class="DigNum (strict)"("DisabledEnum"=w1528) -> ()  [unwired: 2 in, 2 out]
              }
              frame #1 {
                n727 = Wait (ms)(milliseconds to wait=u32 1000) -> ()  [unwired: 1 out]
              }
              frame #2 {
                n728 = property on="Moving Y" class="Str"("Value"="") -> ()  [unwired: 2 in, 2 out]
                n729 = property on="Moving X" class="Str"("Value"="") -> ()  [unwired: 2 in, 2 out]
              }
              frame #3 {
                n730 = Equal?(x=w1533, y=w1534) -> (x = y?=w1532:bool)
                n731 = case shown="True" w1532 {
                  tunnel: w1537 -> [_ w1544]
                  tunnel: w1536 -> [w1538 w1541]
                  tunnel: [w1538 w1539] -> w1535
                  frame False {
                  }
                  frame True {
                    n732 = Unbundle By Name(w1544) -> ("Ref X"=w1543:refnum<vi>, "Ref Y"=w1542:refnum<vi>)
                    n733 = property class="DigNum (strict)"(reference=w1543, error in=w1541) -> (error out=w1540:errorcluster, "Value"=w1546:dbl)  [unwired: 1 out]
                    n734 = property class="DigNum (strict)"(reference=w1542, error in=w1540) -> (error out=w1539:errorcluster, "Value"=w1545:dbl)  [unwired: 1 out]
                    n735 = property on="Position 1" class="DigNum (strict)"("Value"=w1546) -> ()  [unwired: 2 in, 2 out]
                    n736 = property on="Position 2" class="DigNum (strict)"("Value"=w1545) -> ()  [unwired: 2 in, 2 out]
                  }
                }
              }
              frame #4 {
                n737 = property on="Right" class="Bool (strict)"("DisabledEnum"=w1547) -> ()  [unwired: 2 in, 2 out]
                n738 = property on="Up" class="Bool (strict)"("DisabledEnum"=w1547) -> ()  [unwired: 2 in, 2 out]
                n739 = property on="Left" class="Bool (strict)"("DisabledEnum"=w1547) -> ()  [unwired: 2 in, 2 out]
                n740 = property on="Down" class="Bool (strict)"("DisabledEnum"=w1547) -> ()  [unwired: 2 in, 2 out]
                n741 = property on="StepSize" class="DigNum (strict)"("DisabledEnum"=w1547) -> ()  [unwired: 2 in, 2 out]
              }
            }
            n742 = call-poly <userlib>:"Filter 1D Array__ogtk.vi"("items to filter"=w1521, "array"=w1522) -> ("filtered item indices"=w1520:i32[])  [unwired: 4 in, 1 out]
            n743 = Index Array(array=w1520) -> (element=w1515:i32)  [unwired: 1 in]
            n744 = Unbundle By Name(w1523) -> ("active axis refs 2"=w1519:T11, "active ccd"=w1514:i32)
            n745 = Index Array(array=w1519, index=w1515) -> (element=w1518:cluster{"Ref X":refnum<vi>, "Ref Y":refnum<vi>})
            n746 = call <vilib>:"Add State(s) to Queue__jki_lib_state_machine.vi"("State(s) in (\"\")"=w1527) -> ("States Out"=w1526:string)  [unwired: 14 in]
            n747 = local read "Mean Centroid X"() -> (w1524:dbl[][])
            n748 = Bundle By Name(cluster=w1523, "Mean Centroid X"=w1524, "Mean Centroid Y"=w1524) -> (w1525:T37)
          }
          frame "---------------Statistics--------------" {
            # "Template Separator\n(You can make a copy of, or modify, this frame)"
            n749 = call <vilib>:"Add State(s) to Queue__jki_lib_state_machine.vi"("State(s) in (\"\")"=w1551) -> ("States Out"=w1550:string)  [unwired: 14 in]
          }
          frame "Save Stats" {
            # "Your code here.\n(You can make a copy of, or modify, this frame)"
            n750 = property on="CCD 1" class="XYGraph (strict)"() -> ("Value"=w1562:cluster{timestamp[], dbl[]}[])  [unwired: 2 in, 2 out]
            n751 = property on="CCD 2" class="XYGraph (strict)"() -> ("Value"=w1561:cluster{timestamp[], dbl[]}[])  [unwired: 2 in, 2 out]
            n752 = property on="CCD 3" class="XYGraph (strict)"() -> ("Value"=w1560:cluster{timestamp[], dbl[]}[])  [unwired: 2 in, 2 out]
            n753 = property on="CCD 4" class="XYGraph (strict)"() -> ("Value"=w1559:cluster{timestamp[], dbl[]}[])  [unwired: 2 in, 2 out]
            n754 = property on="CCD 5" class="XYGraph (strict)"() -> ("Value"=w1558:cluster{timestamp[], dbl[]}[])  [unwired: 2 in, 2 out]
            n755 = property on="CCD 6" class="XYGraph (strict)"() -> ("Value"=w1557:cluster{timestamp[], dbl[]}[])  [unwired: 2 in, 2 out]
            n756 = property on="CCD 7" class="XYGraph (strict)"() -> ("Value"=w1556:cluster{timestamp[], dbl[]}[])  [unwired: 2 in, 2 out]
            n757 = property on="CCD 8" class="XYGraph (strict)"() -> ("Value"=w1555:cluster{timestamp[], dbl[]}[])  [unwired: 2 in, 2 out]
            n758 = Build Array(w1562, w1561, w1560, w1559, w1558, w1557, w1556, w1555) -> (w1554:cluster{timestamp[], dbl[]}[][])
            n759 = disable-structure shown="Disabled" {
              disable-tunnel: w1566 -> [w1570 _]
              disable-tunnel: [w1569 _] -> w1565
              disable-tunnel: w1554 -> [w1568 _]
              disable-tunnel: w1553 -> [w1567 _]
              frame Disabled {
                n760 = for {
                  tunnel: w1568 -> [w1573] mode=indexing
                  tunnel: w1567 -> [w1572] mode=indexing
                  n761 = Empty String/Path?(string/path=w1572) -> (empty?=w1571:bool)
                  n762 = case shown="False" w1571 {
                    tunnel: w1573 -> [w1579 _]
                    tunnel: w1572 -> [w1577 _]
                    frame False {
                      n763 = Index Array(array=w1579, index #1=0 ("index"), index #2=1 ("index"), index #3=2 ("index"), index #4=3 ("index")) -> (element #1=w1614:cluster{timestamp[], dbl[]}, element #2=w1608:cluster{timestamp[], dbl[]}, element #3=w1607:cluster{timestamp[], dbl[]}, element #4=w1606:cluster{timestamp[], dbl[]})  [unwired: 1 in, 1 out]
                      n764 = Concatenate Strings(w1577, ".dat" ("string")) -> (w1575:string)
                      n765 = Unbundle(w1614) -> (w1613:timestamp[], w1591:dbl[])
                      n766 = Unbundle(w1608) -> (w1582:dbl[])  [unwired: 1 out]
                      n767 = Unbundle(w1607) -> (w1581:dbl[])  [unwired: 1 out]
                      n768 = Unbundle(w1606) -> (w1580:dbl[])  [unwired: 1 out]
                      n769 = Build Path(base path="save path", name or relative path=w1575) -> (appended path=w1574:path)
                      n770 = for {
                        tunnel: w1613 -> [w1616] mode=indexing
                        tunnel: [w1615] -> w1589 mode=indexing
                        n771 = Format Date/Time String(time format string (%c)="%Y%m%d%H%M%S", seconds (now)=w1616) -> (date/time string=w1615:string)  [unwired: 1 in]
                      }
                      n772 = Array Size(array=w1591) -> (size(s)=w1592:i32)
                      n773 = Number To Fractional String(number=w1591) -> (F-format string=w1588:string[])  [unwired: 3 in]
                      n774 = Number To Fractional String(number=w1582) -> (F-format string=w1585:string[])  [unwired: 3 in]
                      n775 = Number To Fractional String(number=w1581) -> (F-format string=w1584:string[])  [unwired: 3 in]
                      n776 = Number To Fractional String(number=w1580) -> (F-format string=w1583:string[])  [unwired: 3 in]
                      n777 = Initialize Array("", w1592, 5 ("dimension size")) -> (w1590:string[][])
                      n778 = Insert Into Array(array=w1590, index (col)=0 ("disabled index (col)"), new element=w1589) -> (w1600:string[][])  [unwired: 1 in]
                      n779 = Insert Into Array(array=w1600, index (col)=1 ("disabled index (col)"), new element=w1588) -> (w1599:string[][])  [unwired: 1 in]
                      n780 = Insert Into Array(array=w1599, index (col)=2 ("disabled index (col)"), new element=w1585) -> (w1603:string[][])  [unwired: 1 in]
                      n781 = Insert Into Array(array=w1603, index (col)=3 ("disabled index (col)"), new element=w1584) -> (w1604:string[][])  [unwired: 1 in]
                      n782 = Insert Into Array(array=w1604, index (col)=4 ("disabled index (col)"), new element=w1583) -> (w1605:string[][])  [unwired: 1 in]
                      n783 = Insert Into Array(array=w1605, index (row)=0, new element=string[] ["time", "Centroid X", "Centroid Y", "Motor Axis 1", "Motor Axis 2"] ("new element/subarray 2")) -> (w1587:string[][])  [unwired: 1 in]
                      n784 = call-poly <vilib>:"Write To Spreadsheet File.vi"("2D data"=w1587, "file path (dialog if empty)"=w1574) -> ()  [unwired: 6 in, 1 out]
                    }
                    frame True {
                    }
                  }
                }
                n785 = call <vilib>:"Add State(s) to Queue__jki_lib_state_machine.vi"("State(s) in (\"\")"=w1570) -> ("States Out"=w1569:string)  [unwired: 14 in]
              }
              frame Enabled {
              }
            }
            n786 = property on="Save Stats" class="Bool (strict)"("Value"=FALSE ("Save Stats")) -> ()  [unwired: 2 in, 2 out]
          }
          frame "tdms" {
            w1627 = 21600.0 ("new tdms")
            # "Your code here.\n(You can make a copy of, or modify, this frame)"
            n787 = Unbundle By Name(w1636) -> ("active cams"=w1620:string[], "Data Value Reference out"=w1635:refnum<k34>, "Offset X"=w1634:dbl[][], "Offset Y"=w1633:dbl[][], "active axis refs 2"=w1632:T11)
            n788 = for {
              tunnel: w1634 -> [w1683]
              tunnel: w1633 -> [w1682]
              tunnel: w1620 -> [w1646] mode=indexing
              tunnel: w1635 -> [w1647]
              tunnel: w1632 -> [w1668]
              tunnel: w1638 -> [w1652]
              tunnel: [w1650] -> w1637
              i -> [w1669]
              n789 = Index Array(array=w1683, index (row)=w1669) -> (element=w1681:dbl[])  [unwired: 1 in]
              n790 = Index Array(array=w1682, index (row)=w1669) -> (element=w1680:dbl[])  [unwired: 1 in]
              n791 = Index Array(array=w1668, index=w1669) -> (element=w1667:cluster{"Ref X":refnum<vi>, "Ref Y":refnum<vi>})
              n792 = Reverse 1D Array(array=w1680) -> (reversed array=w1678:dbl[])
              n793 = Reverse 1D Array(array=w1681) -> (reversed array=w1679:dbl[])
              n794 = Unbundle By Name(w1667) -> ("Ref X"=w1666:refnum<vi>, "Ref Y"=w1665:refnum<vi>)
              n795 = Index Array(array=w1679) -> (element=w1677:dbl)  [unwired: 1 in]
              n796 = Index Array(array=w1678) -> (element=w1676:dbl)  [unwired: 1 in]
              n797 = property class="DigNum (strict)"(reference=w1666, error in=w1652) -> (error out=w1651:errorcluster, "Value"=w1660:dbl)  [unwired: 1 out]
              n798 = Build Array(w1677) -> (w1649:dbl[])
              n799 = Build Array(w1676) -> (w1671:dbl[])
              n800 = Get Date/Time In Seconds() -> (seconds since 1Jan1904=w1648:timestamp)
              n801 = Build Array(w1648) -> (w1644:timestamp[])
              n802 = property class="DigNum (strict)"(reference=w1665, error in=w1651) -> (error out=w1642:errorcluster, "Value"=w1654:dbl)  [unwired: 1 out]
              n803 = Build Array(w1660) -> (w1659:dbl[])
              n804 = TDMS Write(0:w1647, 5:w1646, 7:"time", 9:w1644, 11:w1642) -> (4:w1643:refnum<k34>, 15:w1641:errorcluster)  [unwired: 1 in, 2 out]
              n805 = Build Array(w1654) -> (w1653:dbl[])
              n806 = TDMS Write(0:w1643, 5:w1646, 7:"centroid X", 9:w1649, 11:w1641) -> (4:w1674:refnum<k34>, 6:w1673:string, 15:w1672:errorcluster)  [unwired: 1 in, 1 out]
              n807 = TDMS Write(0:w1674, 5:w1673, 7:"centroid Y", 9:w1671, 11:w1672) -> (4:w1663:refnum<k34>, 6:w1662:string, 15:w1664:errorcluster)  [unwired: 1 in, 1 out]
              n808 = TDMS Write(0:w1663, 5:w1662, 7:"Motor Axis 1", 9:w1659, 11:w1664) -> (4:w1658:refnum<k34>, 6:w1657:string, 15:w1655:errorcluster)  [unwired: 1 in, 1 out]
              n809 = TDMS Write(0:w1658, 5:w1657, 7:"Motor Axis 2", 9:w1653, 11:w1655) -> (15:w1650:errorcluster)  [unwired: 1 in, 3 out]
            }
            n810 = property on="millisecond timer value" class="DigNum (strict)"() -> ("Value"=w1619:u32)  [unwired: 2 in, 2 out]
            n811 = Tick Count (ms)() -> (millisecond timer value=w1618:u32)
            n812 = Unbundle By Name(w1636) -> ()  [unwired: 1 out]
            n813 = Subtract(x=w1618, y=w1619) -> (x-y=w1622:u32)
            n814 = Divide(x=w1622, y=u32 1000) -> (x/y=w1624:dbl)
            n815 = Quotient & Remainder(x=w1624, y=w1627) -> (x-y*floor(x/y)=w1625:dbl)  [unwired: 1 out]
            n816 = Subtract(x=w1627, y=20.0) -> (x-y=w1629:dbl)
            n817 = Greater?(x=w1625, y=w1629) -> (0:w1626:bool)
            n818 = Select(t="newtdms", s=w1626, f="") -> (s? t:f=w1621:string)
            n819 = call <vilib>:"Add State(s) to Queue__jki_lib_state_machine.vi"("State(s) in (\"\")"=w1640, "State(s) at Back (\"\")"=w1621) -> ("States Out"=w1639:string)  [unwired: 13 in]
          }
          frame "Reset History" {
            # "Your code here.\n(You can make a copy of, or modify, this frame)"
            n820 = for {
              N: 1 -> [_]
              shift-right: [w1693] -> w1685
              shift-left: timestamp[][] [] ("Time") -> [w1695]
              n821 = for {
                N: 12 -> [_]
                tunnel: w1695 -> [w1698] mode=indexing
                tunnel: [w1696] -> w1693 mode=indexing
                n822 = Get Date/Time In Seconds() -> (seconds since 1Jan1904=w1697:timestamp)
                n823 = Build Array (concatenate)(w1698, w1697) -> (w1696:timestamp[])
              }
            }
            n824 = local read "Offset X"() -> (w1684:dbl[][])
            n825 = Bundle By Name(cluster=w1689, "Offset X"=w1684, "Offset Y"=w1684, "Time"=w1685, "Motor X"=w1684) -> (w1688:T37)
            n826 = call <vilib>:"Add State(s) to Queue__jki_lib_state_machine.vi"("State(s) in (\"\")"=w1692) -> ("States Out"=w1691:string)  [unwired: 14 in]
          }
          frame "New Category: 2" {
            # "Your code here.\n(You can make a copy of, or modify, this frame)"
            n827 = call <vilib>:"Add State(s) to Queue__jki_lib_state_machine.vi"("State(s) in (\"\")"=w1702) -> ("States Out"=w1701:string)  [unwired: 14 in]
          }
          frame "stats" {
            # "Your code here.\n(You can make a copy of, or modify, this frame)"
            n828 = Unbundle By Name(w1716) -> ("Offset X"=w1714:dbl[][], "Offset Y"=w1713:dbl[][], "Time"=w1712:timestamp[][], "Motor X"=w1711:dbl[][], "Motor Y"=w1710:dbl[][], "Data Value Reference out"=w1706:refnum<k34>)
            n829 = TDMS List Contents(4:w1705, 7:w1706) -> (0:w1709:errorcluster, 2:w1707:string[], 3:w1708:refnum<k34>)  [unwired: 1 in, 1 out]
            n830 = for {
              tunnel: w1709 -> [w1761]
              tunnel: [w1747] -> w1704 mode=indexing
              tunnel: [w1746] -> w1703
              tunnel: [w1745] -> _
              tunnel: w1708 -> [w1744]
              tunnel: w1707 -> [w1743] mode=indexing
              w1762 = dbl[] [] ("appended array")
              n831 = TDMS Read(0:w1744, 5:w1743, 7:"time", 11:w1761, 12:timestamp[] [] ("appended array")) -> (4:w1776:refnum<k34>, 6:w1772:string, 10:w1753:timestamp[], 15:w1760:errorcluster)  [unwired: 3 in, 2 out]
              n832 = TDMS Read(0:w1776, 5:w1772, 7:"centroid X", 11:w1760, 12:w1762) -> (4:w1775:refnum<k34>, 6:w1771:string, 10:w1756:dbl[], 15:w1759:errorcluster)  [unwired: 3 in, 2 out]
              n833 = TDMS Read(0:w1775, 5:w1771, 7:"centroid Y", 11:w1759, 12:w1762) -> (4:w1774:refnum<k34>, 6:w1770:string, 10:w1755:dbl[], 15:w1758:errorcluster)  [unwired: 3 in, 2 out]
              n834 = TDMS Read(0:w1774, 5:w1770, 7:"Motor Axis 1", 11:w1758, 12:w1762) -> (4:w1773:refnum<k34>, 6:w1769:string, 10:w1754:dbl[], 15:w1757:errorcluster)  [unwired: 3 in, 2 out]
              n835 = TDMS Read(0:w1773, 5:w1769, 7:"Motor Axis 2", 11:w1757, 12:w1762) -> (4:w1745:refnum<k34>, 10:w1752:dbl[], 15:w1746:errorcluster)  [unwired: 3 in, 3 out]
              n836 = Bundle("appended array"=w1753, "appended array"=w1756) -> (w1751:T39)  [unwired: 1 in]
              n837 = Bundle("appended array"=w1753, "appended array"=w1755) -> (w1750:T39)  [unwired: 1 in]
              n838 = Bundle("appended array"=w1753, "appended array"=w1754) -> (w1749:T39)  [unwired: 1 in]
              n839 = Bundle("appended array"=w1753, "appended array"=w1752) -> (w1748:T39)  [unwired: 1 in]
              n840 = Build Array(w1751, w1750, w1749, w1748) -> (w1747:T40)
            }
            n841 = disable-structure shown="Disabled" {
              disable-tunnel: w1715 -> [w1783 _]
              disable-tunnel: w1714 -> [w1782 _]
              disable-tunnel: w1713 -> [w1781 _]
              disable-tunnel: w1712 -> [w1780 _]
              disable-tunnel: w1711 -> [w1779 _]
              disable-tunnel: w1710 -> [w1778 _]
              disable-tunnel: [w1777 _] -> _
              frame Disabled {
                n842 = for {
                  tunnel: w1783 -> [_] mode=indexing
                  tunnel: w1782 -> [w1793]
                  tunnel: w1781 -> [w1792]
                  tunnel: w1780 -> [w1791]
                  tunnel: w1779 -> [w1787]
                  tunnel: w1778 -> [w1786]
                  tunnel: [w1795] -> w1777 mode=indexing
                  i -> [w1794]
                  n843 = Index Array(array=w1792, index (row)=w1794) -> (element=w1788:dbl[])  [unwired: 1 in]
                  n844 = Index Array(array=w1793, index (row)=w1794) -> (element=w1789:dbl[])  [unwired: 1 in]
                  n845 = Index Array(array=w1787, index (row)=w1794) -> (element=w1785:dbl[])  [unwired: 1 in]
                  n846 = Index Array(array=w1786, index (row)=w1794) -> (element=w1784:dbl[])  [unwired: 1 in]
                  n847 = Index Array(array=w1791, index (row)=w1794) -> (element=w1790:timestamp[])  [unwired: 1 in]
                  n848 = Bundle("Time"=w1790, "Motor X"=w1785) -> (w1798:cluster{"Time":timestamp[], "Motor X":dbl[]})  [unwired: 1 in]
                  n849 = Bundle("Time"=w1790, "Motor Y"=w1784) -> (w1799:cluster{"Time":timestamp[], "Motor Y":dbl[]})  [unwired: 1 in]
                  n850 = Bundle("Time"=w1790, "Offset X"=w1789) -> (w1797:cluster{"Time":timestamp[], "Offset X":dbl[]})  [unwired: 1 in]
                  n851 = Bundle("Time"=w1790, "Offset Y"=w1788) -> (w1796:cluster{"Time":timestamp[], "Offset Y":dbl[]})  [unwired: 1 in]
                  n852 = Build Array(w1796, w1797, w1798, w1799) -> (w1795:cluster{"Time":timestamp[], "Motor Y":dbl[]}[])
                }
              }
              frame Enabled {
              }
            }
            n853 = call <vilib>:"Add State(s) to Queue__jki_lib_state_machine.vi"("State(s) in (\"\")"=w1742) -> ("States Out"=w1741:string)  [unwired: 14 in]
            n854 = Index Array(array=w1704, index (row) #1=0 ("index (row)"), index (row) #2=1 ("index (row)"), index (row) #3=2 ("index (row)"), index (row) #4=3 ("index (row)"), index (row) #5=4 ("index (row)"), index (row) #6=5 ("index (row)"), index (row) #7=6 ("index (row)"), index (row) #8=7 ("index (row)"), index (row) #9=8 ("index (row)"), index (row) #10=9 ("index (row)"), index (row) #11=10 ("index (row)"), index (row) #12=11 ("index (row)")) -> (element #1=→"CCD 1":T40, element #2=→"CCD 2":T40, element #3=→"CCD 3":T40, element #4=→"CCD 4":T40, element #5=→"CCD 5":T40, element #6=→"CCD 6":T40, element #7=→"CCD 7":T40, element #8=→"CCD 8":T40, element #9=→"CCD 9":T40, element #10=→"CCD 10":T40, element #11=→"CCD 11":T40, element #12=→"CCD 12":T40)  [unwired: 12 in]
          }
          frame "newtdms" {
            # "Your code here.\n(You can make a copy of, or modify, this frame)"
            n855 = Unbundle By Name(w1836) -> ("Data Value Reference out"=w1824:refnum<k34>, "active cams"=w1819:string[])
            n856 = TDMS Close(8:w1834, 11:w1824) -> (0:w1818:errorcluster)  [unwired: 1 out]
            n857 = Get Date/Time In Seconds() -> (seconds since 1Jan1904=w1812:timestamp)
            n858 = call <vilib>:"Clear Errors.vi"("error in (no error)"=w1818) -> ("error out"=w1805:errorcluster)  [unwired: 6 in]
            n859 = Format Date/Time String(time format string (%c)="%Y%m%d", seconds (now)=w1812) -> (date/time string=w1813:string)  [unwired: 1 in]
            n860 = Format Date/Time String(time format string (%c)="%Y%m%d%H%M", seconds (now)=w1812) -> (date/time string=w1810:string)  [unwired: 1 in]
            n861 = property on="new tdms" class="Bool (strict)"("Value"=FALSE ("new tdms")) -> ()  [unwired: 2 in, 2 out]
            n862 = Get Date/Time In Seconds() -> (seconds since 1Jan1904=w1833:timestamp)
            n863 = Format Date/Time String(time format string (%c)="%Y%m%d%H%M", seconds (now)=w1833) -> (date/time string=w1825:string)  [unwired: 1 in]
            n864 = Build Path(base path=w1806, name or relative path=w1813) -> (appended path=w1814:path)
            n865 = Concatenate Strings(w1825, "Beampointingbooster_PICO.tdms" ("string")) -> (w1831:string)
            n866 = String To Path(string=w1831) -> ()  [unwired: 1 out]
            n867 = Concatenate Strings(w1810, "Beampointing_PICObooster.tdms" ("string")) -> (w1808:string)
            n868 = String To Path(string=w1808) -> (path=w1803:path)
            n869 = call <vilib>:"Check if File or Folder Exists.vi"("error in (no error)"=w1805, "path"=w1814) -> ("error out"=w1817:errorcluster, "file or folder exists?"=w1815:bool, "dup path"=w1816:path)  [unwired: 7 in]
            n870 = case shown="False" w1815 {
              tunnel: w1816 -> [w1842 w1844]
              tunnel: [w1841 w1844] -> w1802
              tunnel: w1817 -> [w1840 w1843]
              tunnel: [w1839 w1843] -> w1804
              frame False {
                n871 = Create Folder(path (use dialog)=w1842, error in=w1840) -> (created path=w1841:path, error out=w1839:errorcluster)  [unwired: 1 in, 1 out]
              }
              frame True {
              }
            }
            n872 = call <vilib>:"Add State(s) to Queue__jki_lib_state_machine.vi"("State(s) in (\"\")"=w1838) -> ("States Out"=w1837:string)  [unwired: 14 in]
            n873 = Build Path(base path=w1802, name or relative path=w1803) -> (appended path=w1826:path)
            n874 = TDMS Open(6:FALSE ("disable buffering (T)"), 7:enum16{"1.0", "2.0"}."2.0" ("file format version (2.0)"), 8:w1804, 10:T17."create or replace" ("operation"), 11:w1826) -> (0:w1822:errorcluster, 3:w1821:refnum<k34>)  [unwired: 2 in]
            n875 = call "TDMSbuffersize.vi"("error in (no error)"=w1822, "group names"=w1819, "Data Value Reference in"=w1821) -> ("error out"=w1801:errorcluster, "Data Value Reference out"=w1820:refnum<k34>)  [unwired: 7 in]
            n876 = Bundle By Name(cluster=w1836, "Data Value Reference out"=w1820) -> (w1835:T37)
            n877 = call <vilib>:"Clear Errors.vi"("error in (no error)"=w1801) -> ("error out"=w1800:errorcluster)  [unwired: 6 in]
          }
          frame "Center" {
            # "Your code here.\n(You can make a copy of, or modify, this frame)"
            n878 = control-ref of="image::1"() -> (w1859:refnum<vi>)
            n879 = control-ref of="image::2"() -> (w1858:refnum<vi>)
            n880 = control-ref of="image::3"() -> (w1857:refnum<vi>)
            n881 = control-ref of="image::4"() -> (w1856:refnum<vi>)
            n882 = control-ref of="image::5"() -> (w1855:refnum<vi>)
            n883 = control-ref of="image::6"() -> (w1854:refnum<vi>)
            n884 = control-ref of="image::7"() -> (w1853:refnum<vi>)
            n885 = control-ref of="image::8"() -> (w1852:refnum<vi>)
            n886 = control-ref of="image::9"() -> (w1851:refnum<vi>)
            n887 = control-ref of="image::10"() -> (w1850:refnum<vi>)
            n888 = control-ref of="image::11"() -> (w1849:refnum<vi>)
            n889 = control-ref of="image::12"() -> (w1848:refnum<vi>)
            n890 = for {
              tunnel: [w1868] -> w1847 mode=indexing
              tunnel: w1846 -> [w1867] mode=indexing
              n891 = Unbundle By Name(w1867) -> ("Target.X::12"=w1866:refnum<vi>, "Target.Y::12"=w1865:refnum<vi>)
              n892 = property class="DigNum (strict)"(reference=w1866) -> ("Value"=w1869:dbl)  [unwired: 1 in, 2 out]
              n893 = property class="DigNum (strict)"(reference=w1865) -> ("Value"=w1870:dbl)  [unwired: 1 in, 2 out]
              n894 = Bundle("Value"=w1869, "Value"=w1870) -> (w1868:cluster{"Value":dbl, "Value":dbl})  [unwired: 1 in]
            }
            n895 = call <vilib>:"Add State(s) to Queue__jki_lib_state_machine.vi"("State(s) in (\"\")"=w1864) -> ("States Out"=w1863:string)  [unwired: 14 in]
            n896 = Build Array(w1859, w1858, w1857, w1856, w1855, w1854, w1853, w1852, w1851, w1850, w1849, w1848) -> (w1860:refnum<vi>[])
            n897 = for {
              tunnel: w1860 -> [w1872] mode=indexing
              tunnel: w1847 -> [w1871] mode=indexing
              n898 = property class="ImageControl"(reference=w1872, "Image Center Position"=w1871) -> ()  [unwired: 1 in, 2 out]
            }
            n899 = property on="Center" class="Bool (strict)"("Value"=FALSE ("Center")) -> ()  [unwired: 2 in, 2 out]
          }
          frame "ImgToAvg" {
            n900 = Decimal String To Number(string=w1882) -> (number=w1879:i32)  [unwired: 2 in, 1 out]
            n901 = Bundle By Name(cluster=w1881, "img to avg"=w1879) -> (w1880:T37)
            n902 = call <vilib>:"Build State String with Arguments__jki_lib_state_machine.vi"("Arguments (\"\")"="T" ("Arguments (\"\")"), "State"=" Device Ini") -> ("State with Arguments"=w1873:string)  [unwired: 4 in]
            n903 = call <vilib>:"Add State(s) to Queue__jki_lib_state_machine.vi"("State(s) in Front (\"\")"=w1873, "State(s) in (\"\")"=w1878) -> ("States Out"=w1877:string)  [unwired: 13 in]
          }
          frame "history" {
            # "Your code here.\n(You can make a copy of, or modify, this frame)"
            n904 = Unbundle By Name(w1892) -> ("Offset X"=w1898:dbl[][], "Offset Y"=w1897:dbl[][], "Mean Centroid X"=w1896:dbl[][], "Mean Centroid Y"=w1895:dbl[][], "Motor X"=w1894:dbl[][], "Motor Y"=w1893:dbl[][], "Time"=w1884:timestamp[][])
            n905 = for {
              tunnel: w1898 -> [w1916] mode=indexing
              tunnel: w1897 -> [w1914] mode=indexing
              tunnel: w1896 -> [w1913] mode=indexing
              tunnel: w1895 -> [w1912] mode=indexing
              tunnel: w1894 -> [w1911] mode=indexing
              tunnel: w1893 -> [w1910] mode=indexing
              tunnel: [w1915] -> w1890 mode=indexing
              tunnel: [w1909] -> w1889 mode=indexing
              tunnel: [w1905] -> w1888 mode=indexing
              tunnel: [w1908] -> w1887 mode=indexing
              tunnel: [w1907] -> w1886 mode=indexing
              tunnel: [w1906] -> w1885 mode=indexing
              tunnel: w1884 -> [w1904] mode=indexing
              tunnel: [w1902] -> w1883 mode=indexing
              w1903 = 0
              n906 = Delete From Array(array=w1911, index=w1903) -> (array with subset deleted=w1907:dbl[])  [unwired: 1 in, 1 out]
              n907 = Delete From Array(array=w1910, index=w1903) -> (array with subset deleted=w1906:dbl[])  [unwired: 1 in, 1 out]
              n908 = Delete From Array(array=w1904, index=w1903) -> (array with subset deleted=w1902:timestamp[])  [unwired: 1 in, 1 out]
              n909 = Delete From Array(array=w1913, index=w1903) -> (array with subset deleted=w1905:dbl[])  [unwired: 1 in, 1 out]
              n910 = Delete From Array(array=w1912, index=w1903) -> (array with subset deleted=w1908:dbl[])  [unwired: 1 in, 1 out]
              n911 = Delete From Array(array=w1914, index=w1903) -> (array with subset deleted=w1909:dbl[])  [unwired: 1 in, 1 out]
              n912 = Delete From Array(array=w1916, index=w1903) -> (array with subset deleted=w1915:dbl[])  [unwired: 1 in, 1 out]
            }
            n913 = call <vilib>:"Add State(s) to Queue__jki_lib_state_machine.vi"("State(s) in (\"\")"=w1901) -> ("States Out"=w1900:string)  [unwired: 14 in]
            n914 = Bundle By Name(cluster=w1892, "Offset X"=w1890, "Offset Y"=w1889, "Mean Centroid X"=w1888, "Mean Centroid Y"=w1887, "Motor X"=w1886, "Motor Y"=w1885, "Time"=w1883) -> (w1891:T37)
          }
        }
        n915 = property on="Box" class="Arr (strict)"() -> ("Value"=w141:T6)  [unwired: 2 in, 2 out]
        n916 = for {
          tunnel: w143 -> [w175]
          tunnel: w142 -> [w176]
          tunnel: w139 -> [w156] mode=indexing
          tunnel: w141 -> [w172] mode=indexing
          tunnel: "ljloj" ("overlay name") -> [w160]
          i -> [w162]
          n917 = call-poly <userlib>:"Filter 1D Array__ogtk.vi"("items to filter"=w156, "array"=w176) -> ("filtered item indices"=w177:i32[])  [unwired: 4 in, 1 out]
          n918 = Index Array(array=w177) -> (element=w173:i32)  [unwired: 1 in]
          n919 = Index Array(array=w175, index=w173) -> (element=w174:T31)
          n920 = Unbundle By Name(w174) -> ("Target.X::12"=w179:refnum<vi>, "Target.Y::12"=w178:refnum<vi>)
          n921 = property class="DigNum (strict)"(reference=w179) -> ("Value"=w169:dbl)  [unwired: 1 in, 2 out]
          n922 = property class="DigNum (strict)"(reference=w178) -> ("Value"=w168:dbl)  [unwired: 1 in, 2 out]
          n923 = Bundle By Name(cluster=T14 {"Draw"=TRUE, "Target"={"x"=20.0, "y"=20.0}, "Size"={"x"=20.0, "y"=20.0}, "Angle"=1250067.0, "Color"=1250067} ("Crosshair"), "Draw"=TRUE, "Target.x"=w169, "Target.y"=w168, "Size"=cluster{"xhair size":dbl, "xhair size 2":dbl} {"xhair size"=25.0, "xhair size 2"=25.0} ("size"), "Color"=u32 16774656, "Angle"=0.0) -> (w164:T14)
          n924 = call "draw crosshair imaq.vi"("overlay name"="donotrename", "Crosshair"=w164, "Bounding Rectangle"=T15 {"Left"=0, "Top"=0, "Right"=0, "Bottom"=0}, "image in"=w156) -> ("error out"=→"error out":errorcluster, "image out"=w155:T9)  [unwired: 6 in]
          n925 = call "draw box imaq.vi"("Color"=u32 1244928, "Rectangle"=w172, "image in"=w155) -> ("error out"=→"error out 3":errorcluster)  [unwired: 7 in, 1 out]
          n926 = Number To Decimal String(number=w162) -> (decimal integer string=w161:string)  [unwired: 1 in]
          n927 = Concatenate Strings(w161, w160) -> ()  [unwired: 1 out]
        }
      }
      n928 = call "supergui create stop queue.vi"() -> ("STOP Queue out"=w52:refnum<queue>)  [unwired: 11 in]
      n929 = control-ref of="This Application"() -> (w127:refnum<vi>)
      n930 = control-ref of="This VI"() -> (w131:refnum<vi>)
      n931 = Current VI's Menubar() -> (w130:refnum<k9>)
      n932 = call "GUI_Master_subvi_reentrant_queues.vi"("STOP Queue in"=w52, "This Application"=w127, "error in (no error)"=w128, "tcp data event"=w126, "Caller menu reference"=w130, "Caller VI ref"=w131) -> ("error out"=→"error IO 2":errorcluster)  [unwired: 5 in]
      n933 = Unbundle By Name(w84) -> ("Data Value Reference out"=w83:refnum<k34>)
      n934 = for {
        tunnel: w113 -> [w135] mode=indexing
        tunnel: w112 -> [w134]
        tunnel: [w133] -> w82
        n935 = call "IMAQ Dispose"("Image"=w135, "error in (no error)"=w134) -> ("error out"=w133:errorcluster)  [unwired: 4 in]
      }
      n936 = TDMS Close(8:w82, 11:w83) -> (0:w54:errorcluster)  [unwired: 1 out]
      n937 = Release Queue(queue=w52, error in (no error)=w54) -> (error out=→"error out 2":errorcluster)  [unwired: 1 in, 2 out]
      "Names" <- w57
    }
  }
